vi "AlgoVita Telemetry Tool.vi"() -> ()   [LabVIEW 2020]
uses:
  Typedef Command List.ctl
  <vilib>/Instr/_visa.llb/VISA Configure Serial Port (Instr).vi
  MICS_ID Global.vi
panel:
  out "CRC Errors":u16=2650
  out "Corrected Blocks":u16=2650
  in  "PRIMARY MICS Dongle Address":refnum<visa-resource-name>="COM5"
  out "MAX_RETRIES":bool
  in  "stop":bool
  out "ERROR":bool
  out "SESSION":bool
  out "IDLE":bool
  out "Response":string
  in  "Tab Control":T1(tab)
  in  "Open Session":bool caption="Search for Device"
  in  "Close Session":bool caption="Search for Device"
  in  "Detected MICS IDs":i32(listbox)
  out "Error Monitor":errorcluster
  in  "Dongle Reset":bool caption="Search for Device"
  in  "BASE STATION RF CONTROL":T2={"CCA Mode"=FALSE, "Manual RF CH:"=2, "Base Station CCA Results"=[], "Update CCA"=FALSE, "RSSI Measurement"=0, "Use Averaging?"=TRUE, "400MHz Wakeup"=FALSE, "Listen\nfor\nEmergency"=FALSE} {"RSSI Measurement" items=["External ADC"=0, "Internal ADC"=2]; "Manual RF CH:" max=11 step=1}
  in  "SESSION CONTROL":T3={"TARGET MICS ID"=0, "EXID"=16773121, "Company ID"=187, "Antenna Calibration "=TRUE} {"Company ID" format="%02x"; "EXID" format="%06x"; "TARGET MICS ID" format="%06x"}
  out "LINK QUALITY":T4={"MAX_BIT_ERROR"=FALSE, "MAX_RETRIES"=FALSE, "Corrected Blocks"=2650, "CRC Errors"=2650}
  out "DATA STATUS":T5={"TX_BlockCount"=2650, "RX_BlockCount"=2650, "DataErrorCount"=2650}
  out "STATUS FLAGS":T6
  out "LINK STATUS":T7={"ImplantID"=0, "CompanyID"=0, "RF_Channel"=4, "RX_Mod"=0, "TX_Mod"=0, "TXBlockSize"=15, "RXBlockSize"=15, "BlocksPerPack"=31} {"BlocksPerPack" items=["1"=1, "2"=2, "3"=3, "4"=4, "5"=5, "6"=6, "7"=7, "8"=8, "9"=9, "10"=10, "11"=11, "12"=12, "13"=13, "14"=14, "15"=15, "16"=16, "17"=17, "18"=18, "19"=19, "20"=20, "21"=21, "22"=22, "23"=23, "24"=24, "25"=25, "26"=26, "27"=27, "28"=28, "29"=29, "30"=30, "31"=31]; "RXBlockSize" items=["2"=2, "3"=3, "4"=4, "5"=5, "6"=6, "7"=7, "8"=8, "9"=9, "10"=10, "11"=11, "12"=12, "13"=13, "14"=14, "15"=15, "16"=16, "17"=17, "18"=18, "19"=19, "20"=20, "21"=21, "22"=22, "23"=23, "24"=24, "25"=25, "26"=26, "27"=27, "28"=28, "29"=29, "30"=30, "31"=31]; "TXBlockSize" items=["2"=2, "3"=3, "4"=4, "5"=5, "6"=6, "7"=7, "8"=8, "9"=9, "10"=10, "11"=11, "12"=12, "13"=13, "14"=14, "15"=15, "16"=16, "17"=17, "18"=18, "19"=19, "20"=20, "21"=21, "22"=22, "23"=23, "24"=24, "25"=25, "26"=26, "27"=27, "28"=28, "29"=29, "30"=30, "31"=31]; "TX_Mod" items=["2FSK-FB"=0, "2FSK"=2, "4FSK"=3]; "RX_Mod" items=["2FSK-FB"=0, "2FSK"=8, "4FSK"=12]; "RF_Channel" items=["0", "1", "2", "3", "4", "5", "6", "7", "8", "9"]; "CompanyID" format="%02x"; "ImplantID" format="%06x"}
  out "BASE STATION INFO":string
  in  "Query Error":bool caption="Search for Device"
  in  "BaseStationInfo":enum32{"Type", "Name", "Version", "Error"}(radio)=enum."Error"
  in  "Search for Device":bool
  in  "Device Found?":bool
  in  "Dwell Time (mS)":u32=250
  out "Time to Open Session, Secs":dbl
  out "Error Flag":string="ERROR"
  in  "Clear Error":bool caption="Search for Device"
  in  "TelemGetZarlinkTrim1":bool caption="Search for Device"
  in  "TelemGetGenCals":bool caption="Search for Device"
  in  "TelemOpenLeadLimits":bool caption="Search for Device"
  in  "TelemGetIdentity":bool caption="Search for Device"
  in  "TelemTuneMICS":bool caption="Search for Device"
  in  "TelemStorage":bool caption="Search for Device"
  in  "TelemReset":bool caption="Search for Device"
  in  "TelemGetStatus":bool caption="Search for Device"
  in  "CopyDataToParams":bool caption="Search for Device"
  in  "Load Template":bool caption="Search for Device"
  in  "Telem Driver":bool caption="Search for Device"
  in  "Parameters":string
  out "Data":string
  out "bChecksum Valid":bool
  out "tChecksum Valid":bool
  out "Response Token":string
  out "Response Code":string
  in  "Command":T8
  in  "CP_DATA IN":u8[](array[numeric])
  out "CP_DATA OUT":u8[](array[numeric])
  out "Offset":u16
  out "Bias":u16
  out "Input":u16
  out "Charge/Temp Warning":bool
  out "Temp Cal":bool
  in  "VBAT Polling Speed":enum32{"3s", "5s", "10s", "15s"}(radio)=enum."5s"
  in  "Get VBAT Cont":bool
  in  "Get VBAT Single":bool
  out "Thermometer":dbl(slide) scale=36.0..43.0
  out "Reported Temperature Status":string
  out "Temperature History":dbl(graph)
  out "T1 Cal Factor":dbl format="%_7g"
  out "T1 Ohms":dbl
  out "TEMP (°C)":dbl format="%.3f"
  out "Reported Charging Status":string
  out "Battery Status (Volts)":dbl(slide) scale=3.5..4.12
  out "VRECT Input Power":u8(knob) scale=0.0..255.0
  out "VBAT Cal":dbl format="%_7g"
  out "ADC Counts":dbl
  out "VBAT (Volts)":dbl format="%.3f"
  out "Charging Status":string
  out "Active":i32
  in  "Discharge Target":dbl=3.87
  in  "Discharge":T9(array[cluster]) {"MICS ID" format="%06x"; "VBAT" format="%_3g"}
  in  "LoadPatProgSlot":u8=1 min=1 max=10 step=1
  in  "LoadPatProgFromDevice":bool caption="Search for Device"
  in  "ResetPatProgToDefaults":bool caption="Search for Device"
  in  "LoadPatProgFromFile":bool caption="Search for Device"
  in  "SavePatProgToFile":bool caption="Search for Device"
  in  "PulsePW":u16
  in  "PulsePWDn":bool
  in  "PulsePWUp":bool
  in  "Pulse #":u8=1 min=1 max=4 step=1
  in  "PulseAmpl":u16
  in  "PulseAmpDn":bool
  in  "PulseAmpUp":bool
  in  "StopStimulation":bool caption="Search for Device"
  in  "StartStimulation":bool caption="Search for Device"
  in  "SetPatProgActive":bool caption="Search for Device"
  in  "SendPatProgToDevice":bool caption="Search for Device"
  in  "UpdatePatProgString":bool caption="Search for Device"
  in  "Patient Program String":string
  in  "Freq Index":u8
  in  "ProgAmpls":u16[](array[numeric])
  in  "FreqDn":bool
  in  "FreqUp":bool
  in  "ProgAmpDn":bool
  in  "ProgAmpUp":bool
  in  "PatStim":T10={"PA"={"Defined"=FALSE, "Amplitudes"=[0, 0, 0, 0, 0, 0, 0, 0, 0, 0, 0, 0, 0, 0, 0, 0, 0, 0, 0, 0, 0, 0, 0, 0, 0, 0], "Pulse Name"="", "Label.Ch"=["ch1", "ch2", "ch3", "ch4", "ch5", "ch6", "ch7", "ch8", "ch9", "ch10", "ch11", "ch12", "ch13", "ch14", "ch15", "ch16", "ch17", "ch18", "ch19", "ch20", "ch21", "ch22", "ch23", "ch24", "ch25", "ch26"], "Amp Low Limit (uA)"=0, "Amp Step (uA)"=0, "Amp Step Index"=0, "PW Low Limit (uS)"=0, "PW High Limit (uS)"=0, "PW Default (uS)"=0}, "Allowed Freq Indexes"=[], "PB"={"Defined"=FALSE, "Amplitudes"=[0, 0, 0, 0, 0, 0, 0, 0, 0, 0, 0, 0, 0, 0, 0, 0, 0, 0, 0, 0, 0, 0, 0, 0, 0, 0], "Pulse Name"="", "Label.Ch"=["ch1", "ch2", "ch3", "ch4", "ch5", "ch6", "ch7", "ch8", "ch9", "ch10", "ch11", "ch12", "ch13", "ch14", "ch15", "ch16", "ch17", "ch18", "ch19", "ch20", "ch21", "ch22", "ch23", "ch24", "ch25", "ch26"], "Amp Low Limit (uA)"=0, "Amp Step (uA)"=0, "Amp Step Index"=0, "PW Low Limit (uS)"=0, "PW High Limit (uS)"=0, "PW Default (uS)"=0}, "PC"={"Defined"=FALSE, "Amplitudes"=[0, 0, 0, 0, 0, 0, 0, 0, 0, 0, 0, 0, 0, 0, 0, 0, 0, 0, 0, 0, 0, 0, 0, 0, 0, 0], "Pulse Name"="", "Label.Ch"=["ch1", "ch2", "ch3", "ch4", "ch5", "ch6", "ch7", "ch8", "ch9", "ch10", "ch11", "ch12", "ch13", "ch14", "ch15", "ch16", "ch17", "ch18", "ch19", "ch20", "ch21", "ch22", "ch23", "ch24", "ch25", "ch26"], "Amp Low Limit (uA)"=0, "Amp Step (uA)"=0, "Amp Step Index"=0, "PW Low Limit (uS)"=0, "PW High Limit (uS)"=0, "PW Default (uS)"=0}, "PD"={"Defined"=FALSE, "Amplitudes"=[0, 0, 0, 0, 0, 0, 0, 0, 0, 0, 0, 0, 0, 0, 0, 0, 0, 0, 0, 0, 0, 0, 0, 0, 0, 0], "Pulse Name"="", "Label.Ch"=["ch1", "ch2", "ch3", "ch4", "ch5", "ch6", "ch7", "ch8", "ch9", "ch10", "ch11", "ch12", "ch13", "ch14", "ch15", "ch16", "ch17", "ch18", "ch19", "ch20", "ch21", "ch22", "ch23", "ch24", "ch25", "ch26"], "Amp Low Limit (uA)"=0, "Amp Step (uA)"=0, "Amp Step Index"=0, "PW Low Limit (uS)"=0, "PW High Limit (uS)"=0, "PW Default (uS)"=0}, "label.freqindex"=[], "Default Freq Index"=1, "Program Name"="", "Program Number"=0, "Program Defined"=FALSE, "Program Disabled"=FALSE} {"Default Freq Index" min=1 max=64 step=1; "Allowed Freq Indexes" format="%02x"}
  in  "RFStop":bool
  out "RFST":T11(ring)
  in  "Save RF Scan Report":bool
  in  "Test Device Info (for report):":string
  in  "Run RF Job":bool
  in  "Load RF Job":bool
  in  "Save RF Job":bool
  in  "Test Job Note":string
  in  "Test Job":T12(array[cluster]) {"Attenuator, dB" min=0.0 max=31.25 step=0.25 format="%.2f"}
  out "Wakeup Scan Results":string
  out "RFScanStat":T13 {"Job" scale=0.0..1.0; "Section" scale=0.0..1.0}
  in  "Test Drive Level":enum16{"Low (200uA)", "High (500uA)"}(ring)=enum."High (500uA)"
  in  "Quick Imp Meas":bool
  in  "Channel B":u8=1 min=1 max=25 step=1
  in  "Channel A":u8=1 min=1 max=25 step=1
  in  "Matrix Imp Meas":bool
  in  "Single Imp Meas":bool
  out "Impedance Measurement Results":string
  in  "Clear Device Data":bool
  in  "DevDataSaveAll":bool
  in  "ConstSetAll":bool
  in  "ConstGetAll":bool
  in  "ConstantsGet":bool
  in  "ConstantsSet":bool
  in  "DevDataSave":bool
  in  "ConstantsLoad":bool
  in  "DevDataTabs":T14(tab)=enum."Device Identity"
  out "Activity Log":string
  out "Error Log":string
  out "xPG Identity Data":string
  out "General Calibration Data":string
  out "Pulse Constants Data":string
  out "Program Constants Data":string
  out "HV Calibrations Data":string
  in  "ChanCalTabs":enum32{"0-3mA", "3-6mA", "6-9mA", "9-15mA"}(tab)
  out "Channel Cals 0-3mA":string
  out "Channel Cals 3-6mA":string
  out "Channel Cals 6-9mA":string
  out "Channel Cals 9-15mA":string
  in  "TrimListTabs":T15(tab)
  out "Trim List 0":string
  out "Trim List 1":string
  out "Trim List 2":string
  out "Trim List 3":string
  out "Lead Limits":string
  out "Configurable Device Params":string
  out "Event Counters Data":string
  in  "CPDataTabs":T16(tab)
  out "CP Data 0":string
  out "CP Data 1":string
  out "CP Data 2":string
  out "CP Data 3":string
  out "CP Data 4":string
  out "CP Data 5":string
  out "CP Data 6":string
  out "CP Data 7":string
  in  "ProgramData":T17(tab)
  out "Program Data 1":string
  out "Program Data 2":string
  out "Program Data 3":string
  out "Program Data 4":string
  out "Program Data 5":string
  out "Program Data 6":string
  out "Program Data 7":string
  out "Program Data 8":string
  out "Program Data 9":string
  out "Program Data 10":string
  out "LINK QUALITY MONITOR":T4={"MAX_BIT_ERROR"=FALSE, "MAX_RETRIES"=FALSE, "Corrected Blocks"=2650, "CRC Errors"=2650}
  in  "AttenZero":bool caption="Search for Device"
  in  "Atten -1 dB":bool caption="Search for Device"
  in  "Atten +1 dB":bool caption="Search for Device"
  in  "Set Attenuator":bool caption="Search for Device"
  in  "Get Attenuator":bool caption="Search for Device"
  in  "Attenuation (dB)":dbl min=0.0 max=31.75 step=0.25 format="%.2g"
  out "RSSI Remote 2.45":i16
  out "RSSI Remote 400":i16
  out "RSSI Base 400":i16
  in  "Get RSSI Remote 400":bool
  in  "Remote 400MHz RSSI Mode":T18(ring)=enum."Peak, 10 Rdngs"
  in  "Measurement Type":T19(ring)
  in  "Remote 2.45G RSSI Mode":enum16{"Single Reading", "Average, 20 Rdngs"}(ring)=enum."Average, 20 Rdngs"
  in  "Base 400MHz RSSI Mode":enum16{"Single Reading", "Average, 10 Rdngs"}(ring)=enum."Average, 10 Rdngs"
  in  "Get RSSI Remote 2.45":bool
  in  "Get RSSI Base 400":bool
  in  "400MHz Power - Remote":u8 max=63 step=1 format="%02x"
  in  "Set Remote Pwr":bool
  in  "Set Base Pwr":bool
  in  "245TX Power (dBm)":i8(ring) items=["-29"=-29, "-4"=-4, "-2"=-2, "0"=0, "2"=2, "4"=4, "6"=6, "8"=8, "10"=10, "12"=12, "14"=14, "16"=16, "18"=18, "20"=20, "22"=22, "24"=24, "26"=26, "27"=27]
  in  "400MHz Power - Base":u8 max=63 step=1 format="%02x"
  in  "Set CW":bool
  in  "TX Mode":bool
  in  "Frequency Range":enum16{"2.45GHz", "400MHz"}(ring)
  in  "400MHz Channel":u8 max=11
  out "Wakeup Cal Results":string
  in  "Wakeup Cal Tool":bool caption="Search for Device"
  in  "Enable \"C\" Table":bool
  in  "Enable \"D\" Table":bool
  in  "Valid Entries \"C\"":u8
  in  "Valid Entries \"D\"":u8
  in  "Set_INFO_D":bool caption="Search for Device"
  in  "Get_INFO_D":bool caption="Search for Device"
  in  "Set_INFO_C":bool caption="Search for Device"
  in  "Get_INFO_C":bool caption="Search for Device"
  in  "CalData_C":u8[][](array[numeric]) format="%02x"
  in  "CalData_D":u8[][](array[numeric]) format="%02x"
  in  "File Path":path
  in  "ZL Mass Read":bool caption="Search for Device"
  out "Get Data Dec":u8
  in  "Register":u16(ring)=1000 items=["---MANUAL ENTRY---"=1000, "REG_NOREG"=0, "REG_RXBUFF_USED"=1, "REG_RXBUFF_BSIZE"=2, "REG_TXBUFF_USED"=3, "REG_TXBUFF_BSIZE"=4, "REG_TXBUFF_MAXPACKSIZE"=5, "REG_MAC_ERRCLR"=6, "REG_MAC_TRAINNUM"=7, "REG_MAC_SYNCMATCH"=8, "REG_MAC_SYNC1"=9, "REG_MAC_SYNC2"=10, "REG_MAC_SYNC3"=11, "REG_MAC_SYNC4"=12, "REG_MAC_SYNC5"=13, "REG_MAC_MAXBERR"=14, "REG_MAC_ECCORR"=15, "REG_MAC_CRCERR"=16, "REG_MAC_BLKCNT1"=17, "REG_MAC_BLKCNT2"=18, "REG_MAC_IMDTRANSID1"=19, "REG_MAC_IMDTRANSID2"=20, "REG_MAC_IMDTRANSID3"=21, "REG_MAC_COMPANYID"=22, "REG_MAC_MODUSER"=23, "REG_MAC_CHANNEL"=25, "REG_MAC_CLEARWDOG"=26, "REG_MAC_CKCORRTHRESH"=27, "REG_HK_TXADDR"=28, "REG_HK_TXDATA"=29, "REG_HK_TXREPLY"=30, "REG_HK_USERDATA"=31, "REG_HK_USERSTATUS"=32, "REG_HK_LASTADDRESS"=33, "REG_HK_MODE"=34, "REG_MAC_STATUSSEQ"=35, "REG_MAC_MAXRETRIES"=36, "REG_MAC_RESENDTIME"=37, "REG_MAC_POWERSAVETIME"=38, "REG_MAC_HEAD_DET"=39, "REG_MAC_CTRL"=41, "REG_MAC_INITCOM"=42, "REG_INTERFACE_MODE"=43, "REG_TXRXBUFF_BOTH"=44, "REG_TXRXBUFF"=45, "REG_IRQ_RAWSTATUS1"=46, "REG_IRQ_ENABLE1"=47, "REG_IRQ_ENABLESET1"=48, "REG_IRQ_ENABLECLEAR1"=49, "REG_IRQ_RAWSTATUS2"=50, "REG_IRQ_ENABLE2"=51, "REG_IRQ_ENABLESET2"=52, "REG_IRQ_ENABLECLEAR2"=53, "REG_IRQ_STATUS1"=54, "REG_IRQ_STATUS2"=55, "REG_IRQ_AUXSTATUS"=56, "REG_TXBUFF_OVERFLOW"=57, "REG_PO0"=58, "REG_P01"=59, "REG_P02"=60, "REG_P03"=61, "REG_GP0"=62, "REG_GPI"=63, "REG_WAKEUP_245IN"=64, "REG_WAKEUP_COMPANYID"=65, "REG_WAKEUP_IMDTRANSID1"=66, "REG_WAKEUP_IMDTRANSID2"=67, "REG_WAKEUP_IMDTRANSID3"=68, "REG_WAKEUP_CHANNEL"=69, "REG_WAKEUP_MODUSER"=70, "REG_WAKEUP_DEVICEMODE"=71, "REG_WAKEUP_WK_RX_CTRL1"=72, "REG_WAKEUP_STACK_ADDR"=73, "REG_WAKEUP_CTRL"=74, "REG_WAKEUP_STROSCRTRIM"=75, "REG_WAKEUP_BIASTRIM"=76, "REG_WAKEUP_ANT245TUNE"=77, "REG_WAKEUP_WK_RX_RTRIMDET"=78, "REG_WAKEUP_WK_RX_RTRIMDEMOD"=79, "REG_WAKEUP_WK_RX_RSSIGAIN"=80, "REG_WAKEUP_LNAFREQ1"=81, "REG_WAKEUP_STACK"=83, "REG_WAKUP_XOSU"=84, "REG_WAKUP_CNTDROPOUT"=85, "REG_WAKEUP_CRCCTRL"=86, "REG_WAKEUP_CRCWORD1"=87, "REG_WAKEUP_CRCWORD2"=88, "REG_WAKEUP_WK_RX_CTRIM"=89, "REG_WAKEUP_VDDATRIM"=90, "REG_WAKEUP_VDDDTRIM"=91, "REG_WAKEUP_TESTIOBUFEN"=92, "REG_WAKEUP_TESTIOCLAMP"=93, "CORE_RESET_ADDRESS"=94, "CHIP_RESET_ADDRESS"=95, "REG_RF_TXGENCTRL"=96, "REG_RF_TXIFCTRL"=97, "REG_RF_TXRF_SEL_CTRL"=98, "REG_RF_TXRFPWRDEFAULTSET"=99, "REG_RF_RSSITRIM"=100, "REG_RF_TXIFOSCTUNE"=101, "REG_RF_TXIFGAINIMB"=102, "REG_RF_TXIFLOCK"=103, "REG_RF_RXRFLNAGAINTRIM"=104, "REG_RF_RXBIASTR"=105, "REG_RF_RXGENCTRL"=106, "REG_RF_RXIFADCDECLEV"=107, "REG_RF_RXIFDETFILTERTUNE"=108, "REG_RF_RXIFFILTERTUNE"=109, "REG_RF_GENENABLES"=110, "REG_RF_SYNTH_CHANNEL"=111, "REG_TX_RAMP_RTRIM"=112, "REG_TX_RAMP_CTRIM"=113, "REG_RF_XO_TRIM"=114, "REG_RF_SYNTH_SET_TRIM"=115, "REG_RF_ADCCTRL"=116, "REG_RF_ADCOUTPUT"=117, "REG_RF_TXIFAMP"=118, "REG_RF_SYNTH_RTRIM"=119, "REG_RF_SYNTH_CTRIM"=120, "REG_RF_SYNTH_CT"=121, "REG_RF_TXMIXER_IOSTRIM_HIGH_IP"=122, "REG_RF_TXMIXER_IOSTRIM_HIGH_IN"=123, "REG_RF_TXMIXER_IOSTRIM_HIGH_QP"=124, "REG_RF_TXMIXER_IOSTRIM_HIGH_QN"=125, "REG_HX_WUADDR"=126, "REG_REVISION"=127, "REG_NOREG_TEST"=128, "REG_DTEST_RXBUFF"=129, "REG_RXBUFF_NEXT_BLOCK"=130, "REG_RXBUFF_FIRST_IN_PACK"=131, "REG_RXBUFF_FIRST_EMPTY"=132, "REG_MAC_BYPASS"=133, "REG_DTEST_TXBUFF"=134, "REG_TXBUFF_NEXT_BLOCK"=135, "REG_TXBUFF_FIRST_IN_PACK"=136, "REG_TXBUFF_FIRST_EMPTY"=137, "REG_DTEST_SEQ"=138, "REG_DTEST_CKCORR"=139, "REG_MAC_TOPSTATE"=140, "REG_DTEST_INTERFACE"=141, "REG_IFACE_TXRX_BYPASS"=142, "REG_MAC_TXRXWAIT"=143, "REG_MAC_TXRFRAMP"=144, "REG_MAC_TRAINWORD"=145, "REG_MAC_TRAINWORD2"=146, "REG_MAC_SETTINGS"=147, "REG_MAC_CALSELECT1"=148, "REG_MAC_CALSELECT2"=149, "REG_MAC_ANTMATCHSEL"=150, "REG_MAC_ANTTUNESEL1"=151, "REG_MAC_ANTTUNESEL2"=152, "REG_MAC_ANTTUNESEL3"=153, "REG_MAC_ANTTUNESTEP"=154, "REG_MAC_WUMODEBURST"=156, "REG_MAC_WUOFFSHORT"=157, "REG_MAC_WUOFFLONG"=158, "REG_MAC_CLKRECCTRL"=159, "REG_HK_MODE_P2"=162, "REG_MAC_ANTTUNERES1"=164, "REG_MAC_ANTTUNERES2"=165, "REG_INTERFACE_MODE_TEST"=171, "REG_TXRXBUFF_BOTH_P2"=172, "REG_TXRXBUFF_P2"=173, "REG_IRQ_RAWSTATUS1_P2"=174, "REG_MAC_TXIFSTATUS1"=176, "REG_MAC_TXIFSTATUS2"=177, "REG_IRQ_RAWSTATUS2_P2"=178, "REG_MAC_TXIFRAMPDELAY"=179, "REG_MAC_TXIFRAMPSLOPE"=180, "REG_MAX_TXIFRAMP"=181, "REG_IRQ_STATUS1_P2"=182, "REG_IRQ_STATUS2_P2"=183, "REG_IRQ_AUXSTATUS_P2"=184, "REG_MAC_UNLOCK"=188, "REG_MAC_TXIFFREQ"=190, "REG_WAKEUP_TESTCTRL1"=192, "REG_WAKEUP_RX_EN_CNT"=193, "REG_WAKEUP_TESTENABLES"=194, "REG_WAKEUP_DTBI_CTRL"=195, "REG_WAKEUP_DTBO_CTRL"=196, "REG_WAKEUP_TESTIOBUFTEST"=197, "REG_WAKEUP_WK_RX_TESTCTRL1"=198, "REG_WAKEUP_WK_RX_TESTCTRL2"=199, "REG_WAKEUP_SENS_SEQUENCE_CTRL"=200, "REG_WAKEUP_LNABIAS"=201, "REG_WAKEUP_DET_TH_TRIM1"=202, "REG_WAKEUP_LNABIAS_NOM1"=203, "REG_WAKEUP_RX_TSHORT_TRIM1"=204, "REG_WAKEUP_LNABIAS_NOM2"=205, "REG_WAKEUP_RX_TLONG_TRIM1"=206, "REG_WAKEUP_LNA_NEGRTRIM_NOM1"=207, "REG_WAKEUP_RX_TBURST_TRIM1"=208, "REG_WAKEUP_RX_LNA_NEGRTRIM_NOM2"=209, "REG_WAKEUP_RX_BB_G_BW_SEL1"=210, "REG_WAKEUP_WK_RX_DET_IOSTRIM1"=212, "REG_WAKEUP_WK_RX_CTRL2"=214, "REG_WAKEUP_WK_RX_RSSIVOSTRIM"=215, "REG_WAKEUP_LNANEGR_EFF"=216, "REG_WAKEUP_XOSU_FAST"=217, "REG_WAKEUP_STROSCPWIDTH1"=218, "REG_WAKEUP_STROSCPERIOD1"=220, "REG_WAKEUP_STROSCPERIOD2"=221, "REG_WAKEUP_WK_RX_LNA_NEGRTRIM1"=222, "REG_RF_TXTESTENABLE"=224, "REG_RF_TXIFTESTMODE"=225, "REG_RF_RXTESTENABLE"=226, "REG_RF_RXIFTESTCTRL1"=227, "REG_RF_RXIFTESTCTRL2"=228, "REG_RF_RXIFTESTCTRL3"=229, "REG_RF_SYNTH_TESTCTRL1"=230, "REG_RF_SYNTH_TESTCTRL2"=231, "REG_RF_SYNTH_TESTCTRL3"=232, "REG_RF_ADCTEST1"=237, "REG_RF_ADCTEST2"=238, "REG_RF_TXMIXER_IOSTRIM_LOW_IP"=240, "REG_RF_TXMIXER_IOSTRIM_LOW_IN"=241, "REG_RF_TXMIXER_ISOTRIM_LOW_QP"=242, "REG_RF_TXMIXER_IOSTRIM_LOW_QN"=243, "REG_RF_SYNTH_KPD"=244, "REG_RF_SYNTH_LOLEV"=245, "REG_RF_TXRFPWRTUNEANTSET"=246, "REG_RF_TXPD_GAIN_CTRL"=247, "REG_RF_SYNTH_STARTUP"=248, "REG_RF_TXRFANTTUNE_TXMODE"=249, "REG_RF_TXRFANTTUNE_RXMODE"=250, "REG_RF_RXRFANTTUNE_TXMODE"=251, "REG_RF_RXRFANTTUNE_RXMODE"=252, "REG_ANTMATCH1"=253, "REG_ANTMATCH2"=254, "REG_REVISION_P2"=255]
  in  "Set Register":bool caption="Search for Device"
  in  "Get Register":bool caption="Search for Device"
  in  "Use Remote?":bool
  out "Get Data":u8 format="%02x"
  in  "Set Data":u8 format="%02x"
  in  "Address":u16 format="%04x"
  in  "Do Calibration":bool caption="Search for Device"
  in  "CAL_WAKEUP_STROBE_OSC":bool
  in  "MICS Channel":i8
  in  "Execute on Remote?(F)":bool
  in  "CAL_TX_IF_OSC":bool
  in  "CAL_FM_DETECT_AND_RX_IF":bool
  in  "CAL_RX_ADC":bool
  in  "CAL_400_MHZ_TX":bool
  in  "CAL_400_MHZ_RX":bool
  in  "CAL_400_MHZ_ANT":bool
  in  "CAL_24MHZ_CRYSTAL_OSC":bool
  in  "SECONDARY MICS Dongle Address":refnum<visa-resource-name>="COM9"
  out "error out":errorcluster
  in  "error in (no error)":errorcluster
  in  "Default MICS Config":T20={"ConfigFlags"=0, "ImplantID"=1048576, "CompanyID"=187, "Normal_Comm"={"RF_Channel"=4, "UserData"=0, "TX_Mod"=0, "RX_Mod"=0, "RX_BlockSize"=15, "BlockPerPack"=31, "TX_BlockSize"=15}, "Emerg_Comm"={"RF_Channel"=5, "UserData"=0, "TX_Mod"=0, "RX_Mod"=0, "TX_BlockSize"=15, "BlockPerPack"=31, "RX_BlockSize"=15}, "ImplantRev"=5, "245TX_PowerCal"=10, "245TX_Power"=24, "CCA_RSSI_Thresholds"={"ch0"=2650, "ch1"=2650, "ch2"=2650, "ch3"=2650, "ch4"=2650, "ch5"=2650, "ch6"=2650, "ch7"=2650, "ch8"=2650, "ch9"=2650}} {"ImplantID" format="%x"; "Normal_Comm"."RF_Channel" items=["0", "1", "2", "3", "4", "5", "6", "7", "8", "9"]; "Normal_Comm"."UserData" items=["0 - 000"=0, "1 - 001"=16, "2 - 010"=32, "3 - 011"=48, "4 - 100"=64, "5 - 101"=80, "6 - 110"=96, "7 - 111"=112]; "Normal_Comm"."TX_Mod" items=["2FSK-FB"=0, "2FSK"=2, "4FSK"=3]; "Normal_Comm"."RX_Mod" items=["2FSK-FB"=0, "2FSK"=8, "4FSK"=12]; "Normal_Comm"."RX_BlockSize" items=["2"=2, "3"=3, "4"=4, "5"=5, "6"=6, "7"=7, "8"=8, "9"=9, "10"=10, "11"=11, "12"=12, "13"=13, "14"=14, "15"=15, "16"=16, "17"=17, "18"=18, "19"=19, "20"=20, "21"=21, "22"=22, "23"=23, "24"=24, "25"=25, "26"=26, "27"=27, "28"=28, "29"=29, "30"=30, "31"=31]; "Normal_Comm"."BlockPerPack" items=["1"=1, "2"=2, "3"=3, "4"=4, "5"=5, "6"=6, "7"=7, "8"=8, "9"=9, "10"=10, "11"=11, "12"=12, "13"=13, "14"=14, "15"=15, "16"=16, "17"=17, "18"=18, "19"=19, "20"=20, "21"=21, "22"=22, "23"=23, "24"=24, "25"=25, "26"=26, "27"=27, "28"=28, "29"=29, "30"=30, "31"=31]; "Normal_Comm"."TX_BlockSize" items=["2"=2, "3"=3, "4"=4, "5"=5, "6"=6, "7"=7, "8"=8, "9"=9, "10"=10, "11"=11, "12"=12, "13"=13, "14"=14, "15"=15, "16"=16, "17"=17, "18"=18, "19"=19, "20"=20, "21"=21, "22"=22, "23"=23, "24"=24, "25"=25, "26"=26, "27"=27, "28"=28, "29"=29, "30"=30, "31"=31]; "Emerg_Comm"."RF_Channel" items=["0", "1", "2", "3", "4", "5", "6", "7", "8", "9"]; "Emerg_Comm"."UserData" items=["0 - 000"=0, "1 - 001"=16, "2 - 010"=32, "3 - 011"=48, "4 - 100"=64, "5 - 101"=80, "6 - 110"=96, "7 - 111"=112]; "Emerg_Comm"."TX_Mod" items=["2FSK-FB"=0, "2FSK"=2, "4FSK"=3]; "Emerg_Comm"."RX_Mod" items=["2FSK-FB"=0, "2FSK"=8, "4FSK"=12]; "Emerg_Comm"."TX_BlockSize" items=["2"=2, "3"=3, "4"=4, "5"=5, "6"=6, "7"=7, "8"=8, "9"=9, "10"=10, "11"=11, "12"=12, "13"=13, "14"=14, "15"=15, "16"=16, "17"=17, "18"=18, "19"=19, "20"=20, "21"=21, "22"=22, "23"=23, "24"=24, "25"=25, "26"=26, "27"=27, "28"=28, "29"=29, "30"=30, "31"=31]; "Emerg_Comm"."BlockPerPack" items=["1"=1, "2"=2, "3"=3, "4"=4, "5"=5, "6"=6, "7"=7, "8"=8, "9"=9, "10"=10, "11"=11, "12"=12, "13"=13, "14"=14, "15"=15, "16"=16, "17"=17, "18"=18, "19"=19, "20"=20, "21"=21, "22"=22, "23"=23, "24"=24, "25"=25, "26"=26, "27"=27, "28"=28, "29"=29, "30"=30, "31"=31]; "Emerg_Comm"."RX_BlockSize" items=["2"=2, "3"=3, "4"=4, "5"=5, "6"=6, "7"=7, "8"=8, "9"=9, "10"=10, "11"=11, "12"=12, "13"=13, "14"=14, "15"=15, "16"=16, "17"=17, "18"=18, "19"=19, "20"=20, "21"=21, "22"=22, "23"=23, "24"=24, "25"=25, "26"=26, "27"=27, "28"=28, "29"=29, "30"=30, "31"=31]; "ImplantRev" items=["ZL70100"=0, "ZL70101"=1, "ZL70102"=4, "ZL70103"=5]; "245TX_PowerCal" items=["-29"=-29, "-4"=-4, "-2"=-2, "0"=0, "2"=2, "4"=4, "6"=6, "8"=8, "10"=10, "12"=12, "14"=14, "16"=16, "18"=18, "20"=20, "22"=22, "24"=24, "26"=26, "27"=27]; "245TX_Power" items=["-29"=-29, "-4"=-4, "-2"=-2, "0"=0, "2"=2, "4"=4, "6"=6, "8"=8, "10"=10, "12"=12, "14"=14, "16"=16, "18"=18, "20"=20, "22"=22, "24"=24, "26"=26, "27"=27]}
  in  "Enable WD?":bool
  in  "Wait Time (S)":u8=5
  in  "Discharge Delay":u32
  in  "Tick Count":u32
  in  "AttenMode":enum16{"Null", "Increment", "Decrement", "Zero"}(ring)
  out "Busy Flag":string="BUSY"
  out "Working MICS Config":T20
  # "Double-Click to Select"
  # "400MHz\nWakeup"
  # "Auto CCA"
  # "NOTE:  Changing the active tab will suspend the operation of the Mass Battery Discharge Tool!"
  # "CHARGING STATUS"
  # "DEVICE TEMPERATURE"
  # "MASS BATTERY DISCHARGE TOOL"
  # "Volts"
  # "x"
  # "="
  # "x"
  # "="
  # "-Abort"
  # "(Input-Offset)"
  # "R="
  # "----------------- *47000"
  # "-Critical"
  # "(Bias-Input)"
  # "-Warn"
  # "++++"
  # "When charging with manual power control,\nmaintain \"VRECT Input Power\" in the range\nof 130-150 (the \"Green\" zone on meter)."
  # "MICS ID"
  # "PA"
  # "PB"
  # "PC"
  # "PD"
  # "Program Adjust"
  # "Pulse Adjust"
  # "Pulse D"
  # "Pulse C"
  # "Pulse B"
  # "Pulse A"
  # "MICS WAKEUP SCAN"
  # "All CH referenced to STCH14."
  # "IMPEDANCE MEASUREMENT"
  # "WARNING: \"Full Matrix\"\nImpedance Measurements\ncan take several minutes!"
  # "ATTENUATOR"
  # "RSSI MEASUREMENTS"
  # "BASE STATION 400MHz RSSI"
  # "REMOTE 400MHz RSSI"
  # "(Must be in session)"
  # "REMOTE 2.45GHz RSSI"
  # "(Must be in session)"
  # "DEVICE RF POWER SETTINGS"
  # "BASE STATION"
  # "REMOTE DEVICE"
  # "(Must be in session)"
  # "CW TEST MODE CONTROL"
  # "ON"
  # "OFF"
  # "ZL REGISTER PEEK AND POKE"
  # "ZL REGISTER MASS READ TO FILE"
  # "MICS DONGLE CALIBRATION"
  # "INFO_D"
  # "Index"
  # "Address"
  # "Data"
  # "Use \"Register\" menu list for named registers,\nor leave it on \"Manual Entry\" and use the \n\"Address\" control to select a register address.\n          (Add 128 (0x80) to P2 addresses)"
  # "Use this function to copy all Zarlink registers to\na text file."
  # "INFO_C"
  # "Index"
  # "Address"
  # "Data"
  # "WAKEUP CALIBRATOR TOOL"
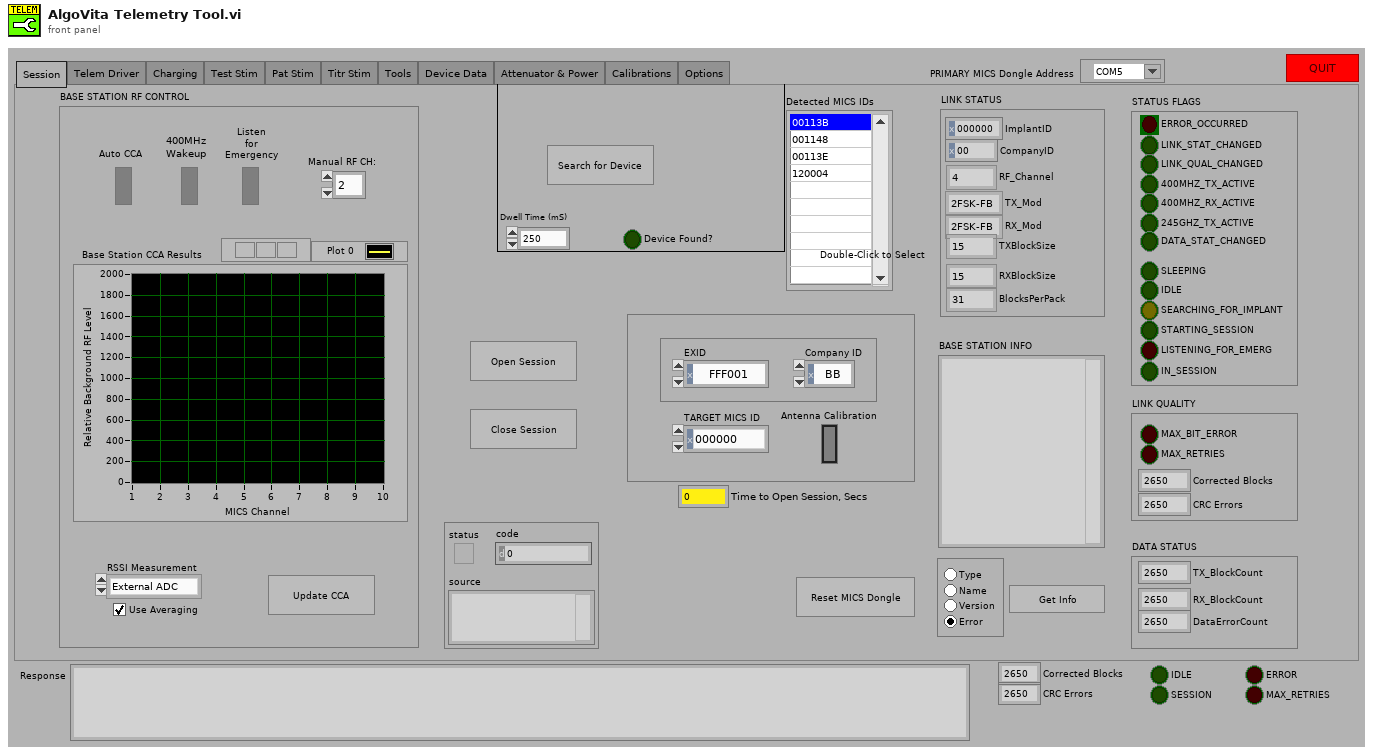
[diagram p1: front panel]
types:
  T1 = enum32{"Session", "Telem Driver", "Charging", "Test Stim", "Pat Stim", "Titr Stim", "Tools", "Device Data", "Attenuator & Power", "Calibrations", "Options"}
  T2 = cluster{"CCA Mode":bool, "Manual RF CH:":u8, "Base Station CCA Results":dbl[], "Update CCA":bool, "RSSI Measurement":u16, "Use Averaging?":bool, "400MHz Wakeup":bool, "Listen\nfor\nEmergency":bool}
  T3 = cluster{"TARGET MICS ID":u32, "EXID":u32, "Company ID":u8, "Antenna Calibration ":bool}
  T4 = cluster{"MAX_BIT_ERROR":bool, "MAX_RETRIES":bool, "Corrected Blocks":u16, "CRC Errors":u16}
  T5 = cluster{"TX_BlockCount":u16, "RX_BlockCount":u16, "DataErrorCount":u16}
  T6 = cluster{"ERROR_OCCURRED":bool, "LINK_STAT_CHANGED":bool, "LINK_QUAL_CHANGED":bool, "400MHZ_TX_ACTIVE":bool, "400MHZ_RX_ACTIVE":bool, "245GHZ_TX_ACTIVE":bool, "DATA_STAT_CHANGED":bool, "SLEEPING":bool, "IDLE":bool, "SEARCHING_FOR_IMPLANT":bool, "STARTING_SESSION":bool, "LISTENING_FOR_EMERG":bool, "IN_SESSION":bool}
  T7 = cluster{"ImplantID":u32, "CompanyID":u8, "RF_Channel":u8, "RX_Mod":u8, "TX_Mod":u8, "TXBlockSize":u8, "RXBlockSize":u8, "BlocksPerPack":u8}
  T8 = typedef "Typedef Command List.ctl" = enum16{"Get xPG Status", "xPG Stimulation", "Select Program", "Increment Program Amplitude", "Decrement Program Amplitude", "Get PoP Constants", "Get PPC Constants", "Get Program Names", "Set Pulse Amplitude", "Increment Pulse Amplitude", "Decrement Pulse Amplitude", "Get Pulse Widths", "Set Pulse Widths", "Increment Pulse Width", "Decrement Pulse Width", "Get Program Frequency", "Set Program Frequency", "Increment Program Frequency", "Decrement Program Frequency", "Inject Event", "Charging Control", "Get xPG Identity", "Set xPG Identity", "Restore Program Defaults", "Get Program Definition", "Set Program Definition", "Get Program Constants", "Set Program Constants", "Get Configurable Device Parameters", "Set Configurable Device Parameters", "Get Pulse Constants", "Set Pulse Constants", "Get Lead Limits", "Set Lead Limits", "Get Channel Calibrations", "Set Channel Calibrations", "<reserved 2>", "<reserved 3>", "<reserved 4>", "<reserved 5>", "<reserved 6>", "<reserved 7>", "Get Stim Asic HV Calibrations", "Set Stim Asic HV Calibrations", "<reserved 8>", "<reserved 9>", "Get CP Data", "Set CP Data", "Clear Log", "Read Log", "Append Log", "Get Patient Program Runtime", "Set Patient Program Runtime", "Impedance Measurement", "Enter Storage Mode", "Echo Short", "Echo Long", "Get General Calibration", "Set General Calibration", "Get Trim List", "Set Trim List", "Get Counter", "Set Counter", "Get Test Stimulation", "Set Test Stimulation", "Get Titration Stimulation", "Set Titration Stimulation", "Get Ramp Time", "Set Ramp Time", "Get VBAT", "Set Software Description Block", "Get Software Description Block", "Write Memory", "Read Memory", "Reset xPG", "Erase Flash Block", "Write Vectors", "Read Vectors", "Diagnostic Data", "Set Background Impedance", "Get Background Impedence ", "Set Test Waveform", "Calibrate Channel", "Get Log Range", "Reserved 0x55", "Reserved 0x56", "MICS Options", "Pair PPC", "Pair POP", "Stop Bootloader", "Tune MICS", "MICS Diagnostics", "Undefined"}
  T9 = cluster{"Activate":bool, "Stop":bool, "VBAT":dbl, "Discharging":bool, "Ready":bool, "MICS ID":u32}[]
  T10 = cluster{"PA":cluster{"Defined":bool, "Amplitudes":i8[], "Pulse Name":string, "Label.Ch":string[], "Amp Low Limit (uA)":u16, "Amp Step (uA)":u16, "Amp Step Index":u16, "PW Low Limit (uS)":u16, "PW High Limit (uS)":u16, "PW Default (uS)":u16}, "Allowed Freq Indexes":u8[], "PB":cluster{"Defined":bool, "Amplitudes":i8[], "Pulse Name":string, "Label.Ch":string[], "Amp Low Limit (uA)":u16, "Amp Step (uA)":u16, "Amp Step Index":u16, "PW Low Limit (uS)":u16, "PW High Limit (uS)":u16, "PW Default (uS)":u16}, "PC":cluster{"Defined":bool, "Amplitudes":i8[], "Pulse Name":string, "Label.Ch":string[], "Amp Low Limit (uA)":u16, "Amp Step (uA)":u16, "Amp Step Index":u16, "PW Low Limit (uS)":u16, "PW High Limit (uS)":u16, "PW Default (uS)":u16}, "PD":cluster{"Defined":bool, "Amplitudes":i8[], "Pulse Name":string, "Label.Ch":string[], "Amp Low Limit (uA)":u16, "Amp Step (uA)":u16, "Amp Step Index":u16, "PW Low Limit (uS)":u16, "PW High Limit (uS)":u16, "PW Default (uS)":u16}, "label.freqindex":string[], "Default Freq Index":u8, "Program Name":string, "Program Number":u8, "Program Defined":bool, "Program Disabled":bool}
  T11 = enum16{"Not Running", "Idle Interval...", "Opening Session..."}
  T12 = cluster{"Number of Runs":dbl, "2.45G_TX_Pwr":enum16{"-29", "-4", "-2", "0", "2", "4", "6", "8", "10", "12", "14", "16", "18", "20", "22", "24", "26", "27"}, "400M_TX_Pwr":enum8{"Default", "1", "2", "3", "4", "5", "6", "7", "8", "9", "10", "11", "12", "13", "14", "15", "16", "17", "18", "19", "20", "21", "22", "23", "24", "25", "26", "27", "28", "29", "30", "31"}, "Idle Interval, S":dbl, "Attenuator, dB":dbl, "MICS Chan":enum16{"CH 1", "CH 2", "CH 3", "CH 4", "CH 5", "CH 6", "CH 7", "CH 8", "CH 9", "CH 10"}, "Random\nOffset":bool}[]
  T13 = cluster{"Section":dbl, "Job":dbl, "Last Open Session Time, S":dbl, "Session Verified?":bool, "Average Open Session Time, S":dbl, "# of Open Session Failures":u16}
  T14 = enum32{"Activity Log", "Error Log", "Device Identity", "General Cals", "Pulse Constants", "Program Constants", "HV Cals", "Channel Cals", "Trim Lists", "Lead Limits", "Configurable Device Params", "Event Counters", "CP Data", "Stim Programs"}
  T15 = enum32{"Trim List 0", "Trim List 1", "Trim List 2", "Trim List 3"}
  T16 = enum32{"CP Data 0", "CP Data 1", "CP Data 2", "CP Data 3", "CP Data 4", "CP Data 5", "CP Data 6", "CP Data 7"}
  T17 = enum32{"Program 1", "Program 2", "Program 3", "Program 4", "Program 5", "Program 6", "Program 7", "Program 8", "Program 9", "Program 10"}
  T18 = enum16{"Single Reading", "Average, 10 Rdngs", "Peak, 10 Rdngs"}
  T19 = enum8{"EXT_RSSI_EXT_ADC (0)", "EXT_RSSI_INT_ADC (1)", "INT_RSSI_INT_ADC (2)"}
  T20 = cluster{"ConfigFlags":u8, "ImplantID":u32, "CompanyID":u8, "Normal_Comm":cluster{"RF_Channel":u8, "UserData":u8, "TX_Mod":u8, "RX_Mod":u8, "RX_BlockSize":u8, "BlockPerPack":u8, "TX_BlockSize":u8}, "Emerg_Comm":cluster{"RF_Channel":u8, "UserData":u8, "TX_Mod":u8, "RX_Mod":u8, "TX_BlockSize":u8, "BlockPerPack":u8, "RX_BlockSize":u8}, "ImplantRev":u8, "245TX_PowerCal":i8, "245TX_Power":i8, "CCA_RSSI_Thresholds":cluster{"ch0":u16, "ch1":u16, "ch2":u16, "ch3":u16, "ch4":u16, "ch5":u16, "ch6":u16, "ch7":u16, "ch8":u16, "ch9":u16}}
  T21 = cluster{"Command":T8, "Function":enum16{"Open Session", "Close Session", "Downlink Only", "Uplink Only", "Transceive (DN -> UP)"}, "MICS_ID":u32, "EXID":u32, "Use Local":bool, "Transceive Delay mS":dbl, "CP_DATA IN":u8[], "Parameters":string}
  T22 = enum16{"Open Session", "Close Session", "Downlink Only", "Uplink Only", "Transceive (DN -> UP)"}
  T23 = enum8{"Enabled", "Disabled", "Disabled and Grayed Out"}
  T24 = cluster{"Activate":bool, "Stop":bool, "VBAT":dbl, "Discharging":bool, "Ready":bool, "MICS ID":u32}
  T25 = enum16{"Start Search", "Continue Search", "End Search"}
  T26 = enum16{"open", "replace", "create", "open or create", "replace or create", "replace or create with confirmation"}
  T27 = enum16{"Get Device Type", "Get Device Name", "Get Device Version", "Get Device Error"}
  T28 = cluster{"Response Token":string, "Response Code":string, "bChecksum Valid":bool, "tChecksum Valid":bool, "CP_DATA OUT":u8[], "Data":string}
  T29 = cluster{"Allowed Freq Indexes[0]":u8, "Allowed Freq Indexes[1]":u8, "Allowed Freq Indexes[2]":u8, "Allowed Freq Indexes[3]":u8, "Allowed Freq Indexes[4]":u8, "Allowed Freq Indexes[5]":u8, "Allowed Freq Indexes[6]":u8, "Allowed Freq Indexes[7]":u8}
  T30 = cluster{"Number of Runs":dbl, "2.45G_TX_Pwr":enum16{"-29", "-4", "-2", "0", "2", "4", "6", "8", "10", "12", "14", "16", "18", "20", "22", "24", "26", "27"}, "400M_TX_Pwr":enum8{"Default", "1", "2", "3", "4", "5", "6", "7", "8", "9", "10", "11", "12", "13", "14", "15", "16", "17", "18", "19", "20", "21", "22", "23", "24", "25", "26", "27", "28", "29", "30", "31"}, "Idle Interval, S":dbl, "Attenuator, dB":dbl, "MICS Chan":enum16{"CH 1", "CH 2", "CH 3", "CH 4", "CH 5", "CH 6", "CH 7", "CH 8", "CH 9", "CH 10"}, "Random\nOffset":bool}
  T31 = enum16{"-29", "-4", "-2", "0", "2", "4", "6", "8", "10", "12", "14", "16", "18", "20", "22", "24", "26", "27"}
  T32 = enum8{"Default", "1", "2", "3", "4", "5", "6", "7", "8", "9", "10", "11", "12", "13", "14", "15", "16", "17", "18", "19", "20", "21", "22", "23", "24", "25", "26", "27", "28", "29", "30", "31"}
  T33 = enum16{"CH 1", "CH 2", "CH 3", "CH 4", "CH 5", "CH 6", "CH 7", "CH 8", "CH 9", "CH 10"}
  T34 = cluster{"Test Job Note":string, "Test Job":cluster{"Number of Runs":dbl, "2.45G_TX_Pwr":enum16{"-29", "-4", "-2", "0", "2", "4", "6", "8", "10", "12", "14", "16", "18", "20", "22", "24", "26", "27"}, "400M_TX_Pwr":enum8{"Default", "1", "2", "3", "4", "5", "6", "7", "8", "9", "10", "11", "12", "13", "14", "15", "16", "17", "18", "19", "20", "21", "22", "23", "24", "25", "26", "27", "28", "29", "30", "31"}, "Idle Interval, S":dbl, "Attenuator, dB":dbl, "MICS Chan":enum16{"CH 1", "CH 2", "CH 3", "CH 4", "CH 5", "CH 6", "CH 7", "CH 8", "CH 9", "CH 10"}, "Verify\nSessions":bool}[]}
  T35 = cluster{"Number of Runs":dbl, "2.45G_TX_Pwr":enum16{"-29", "-4", "-2", "0", "2", "4", "6", "8", "10", "12", "14", "16", "18", "20", "22", "24", "26", "27"}, "400M_TX_Pwr":enum8{"Default", "1", "2", "3", "4", "5", "6", "7", "8", "9", "10", "11", "12", "13", "14", "15", "16", "17", "18", "19", "20", "21", "22", "23", "24", "25", "26", "27", "28", "29", "30", "31"}, "Idle Interval, S":dbl, "Attenuator, dB":dbl, "MICS Chan":enum16{"CH 1", "CH 2", "CH 3", "CH 4", "CH 5", "CH 6", "CH 7", "CH 8", "CH 9", "CH 10"}, "Verify\nSessions":bool}[]
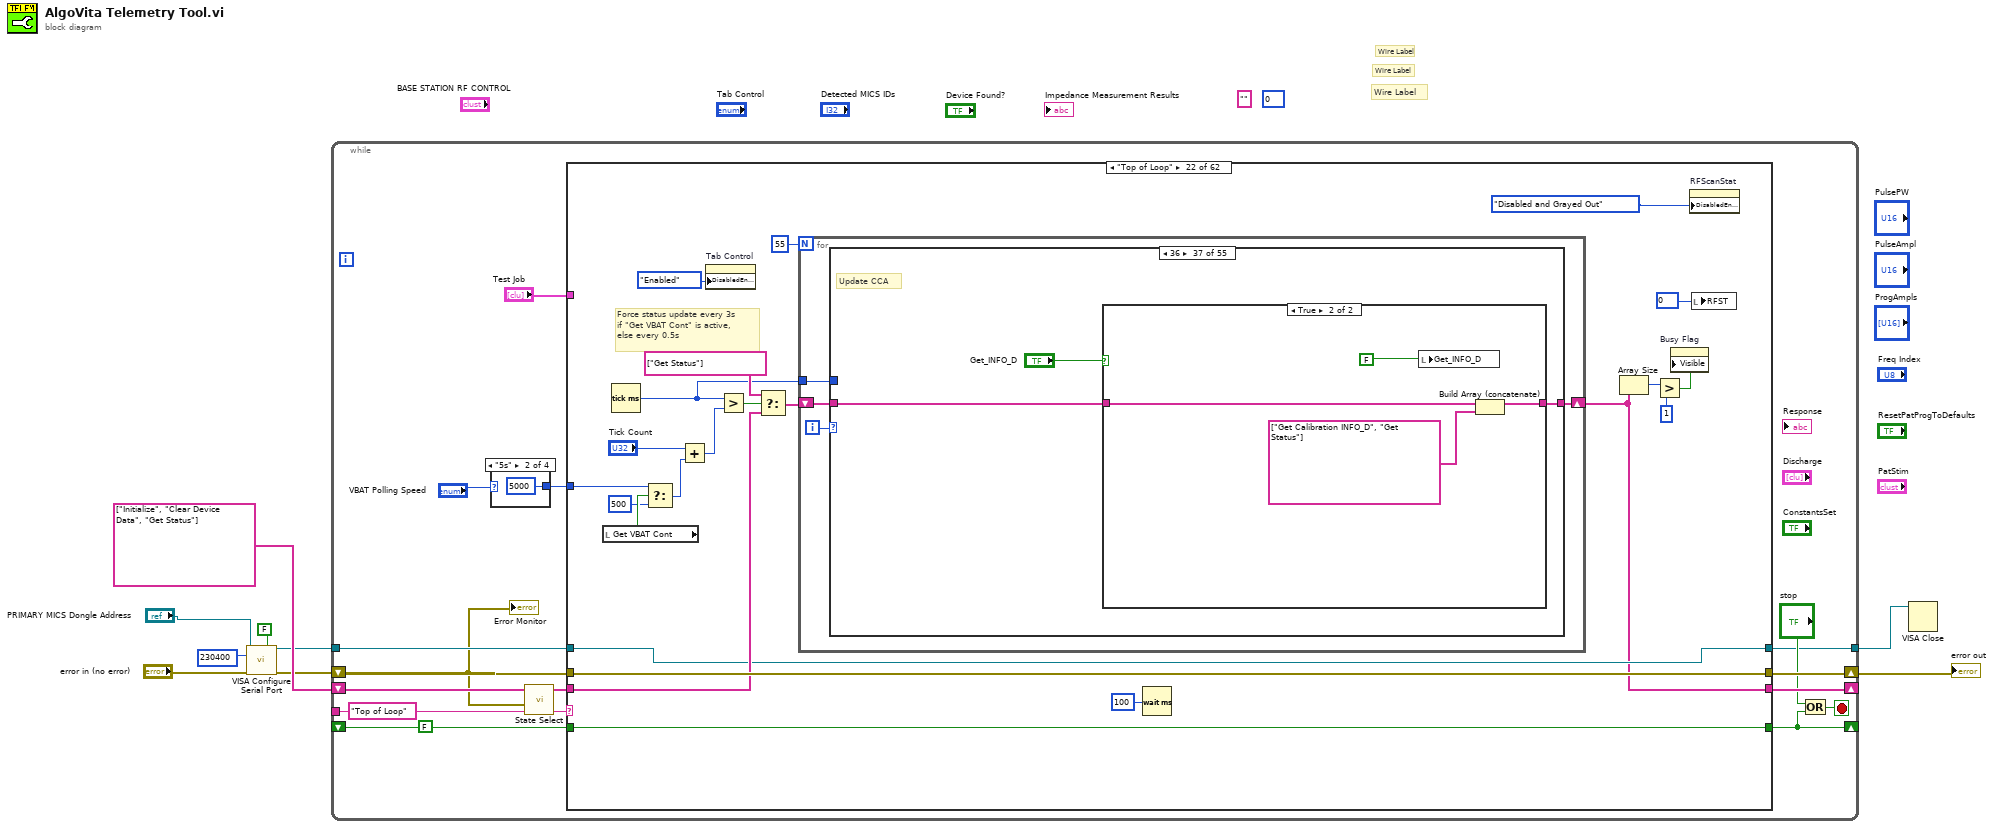
[diagram p0: block diagram]
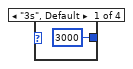
[diagram p2: hidden frame]
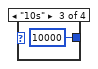
[diagram p3: hidden frame]
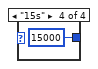
[diagram p4: hidden frame]
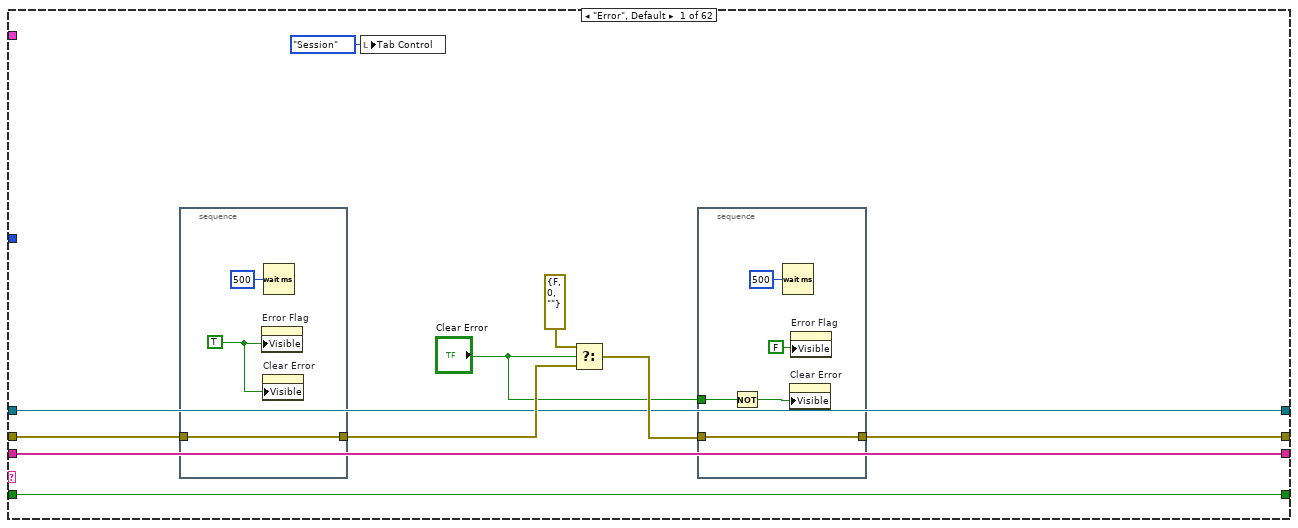
[diagram p5: hidden frame]
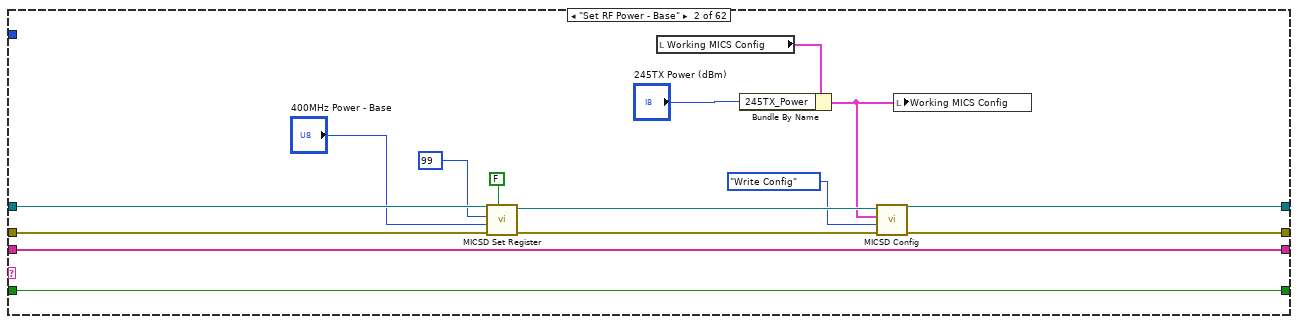
[diagram p6: hidden frame]
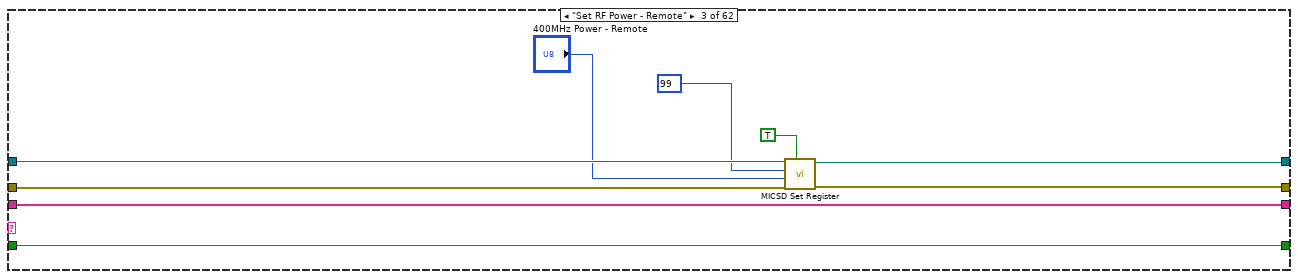
[diagram p7: hidden frame]
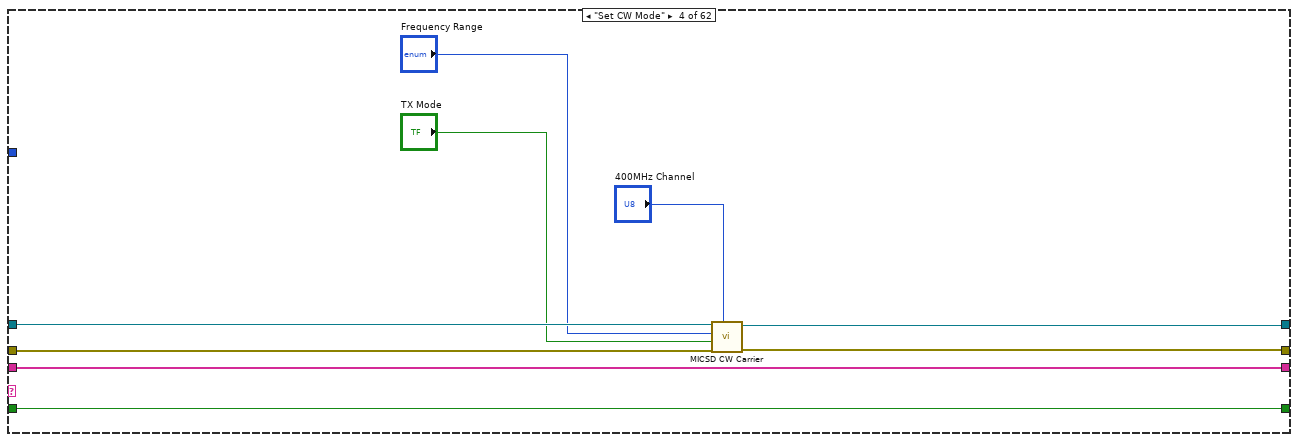
[diagram p8: hidden frame]
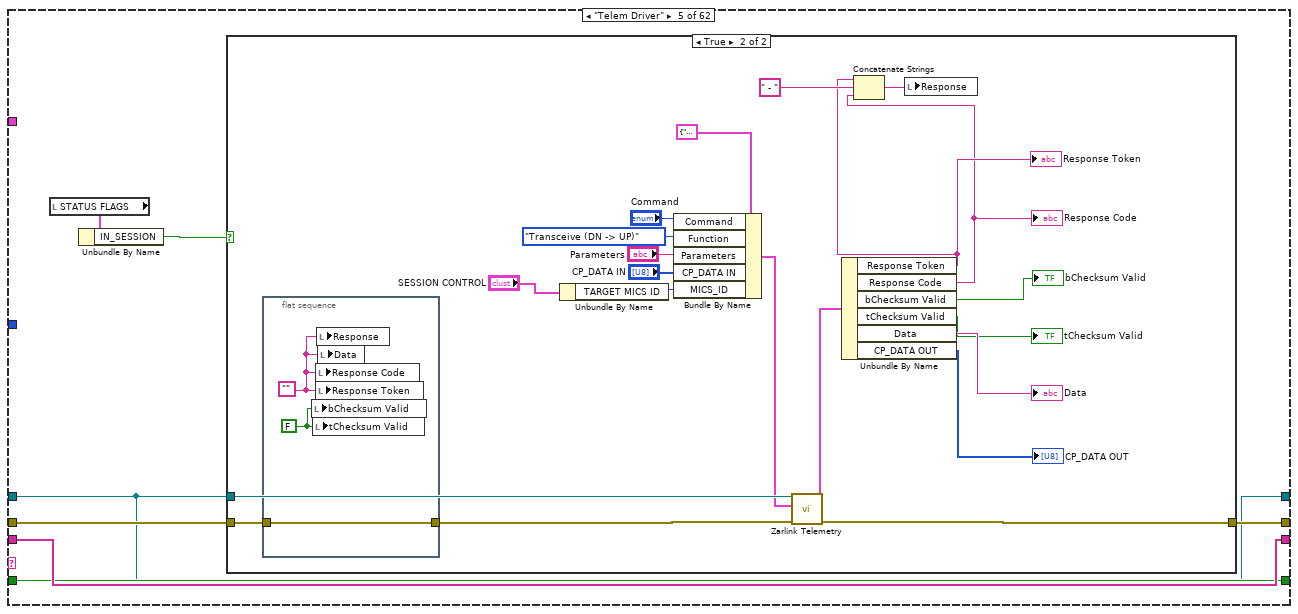
[diagram p9: hidden frame]
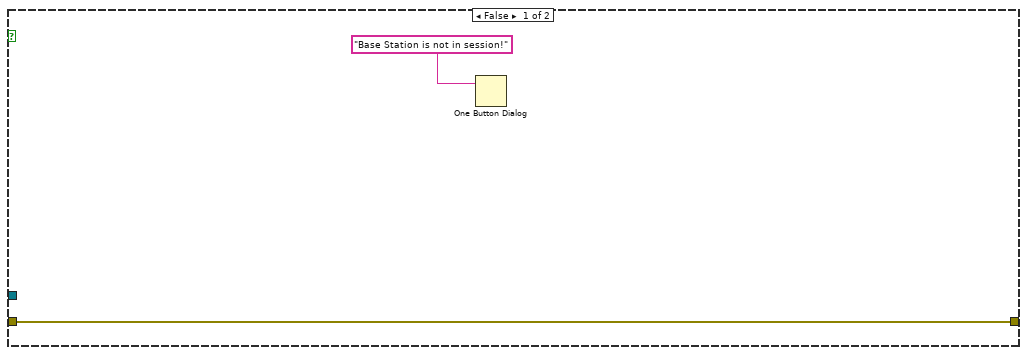
[diagram p10: hidden frame]
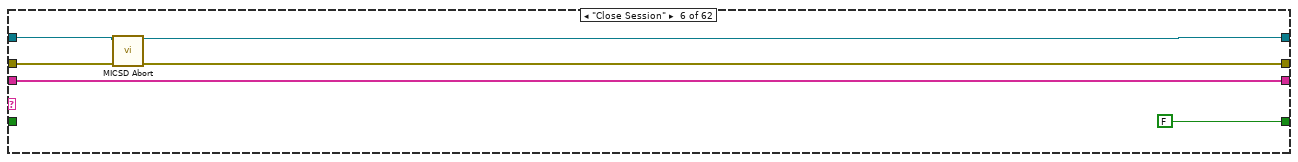
[diagram p11: hidden frame]
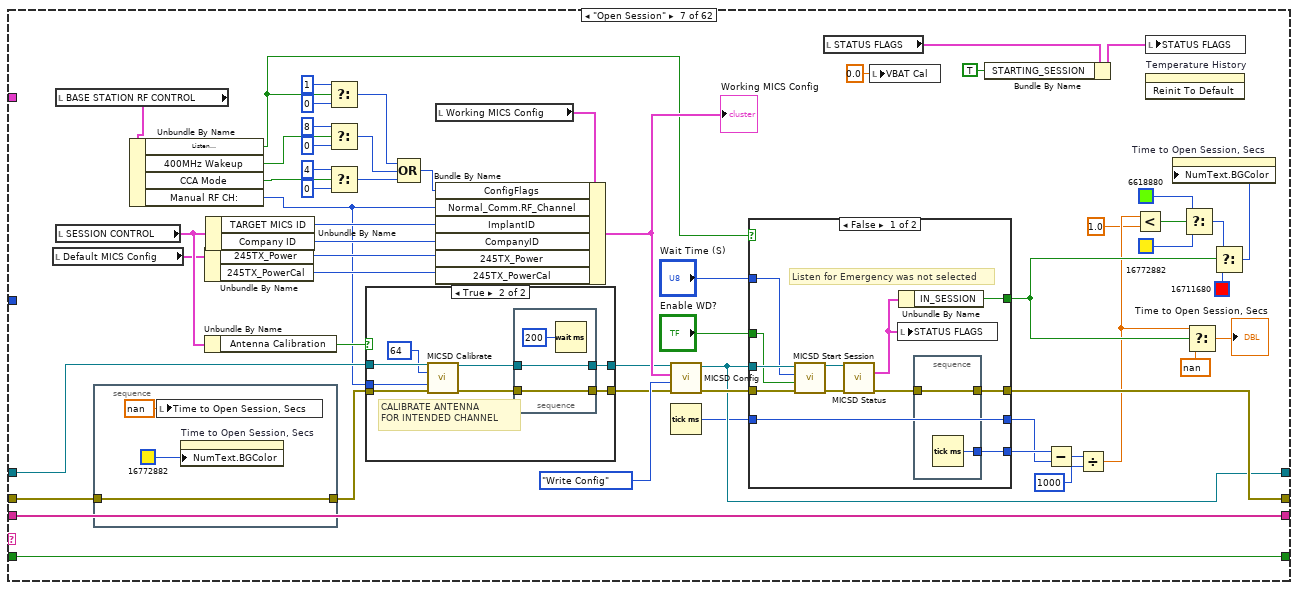
[diagram p12: hidden frame]
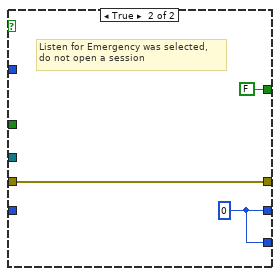
[diagram p14: hidden frame]
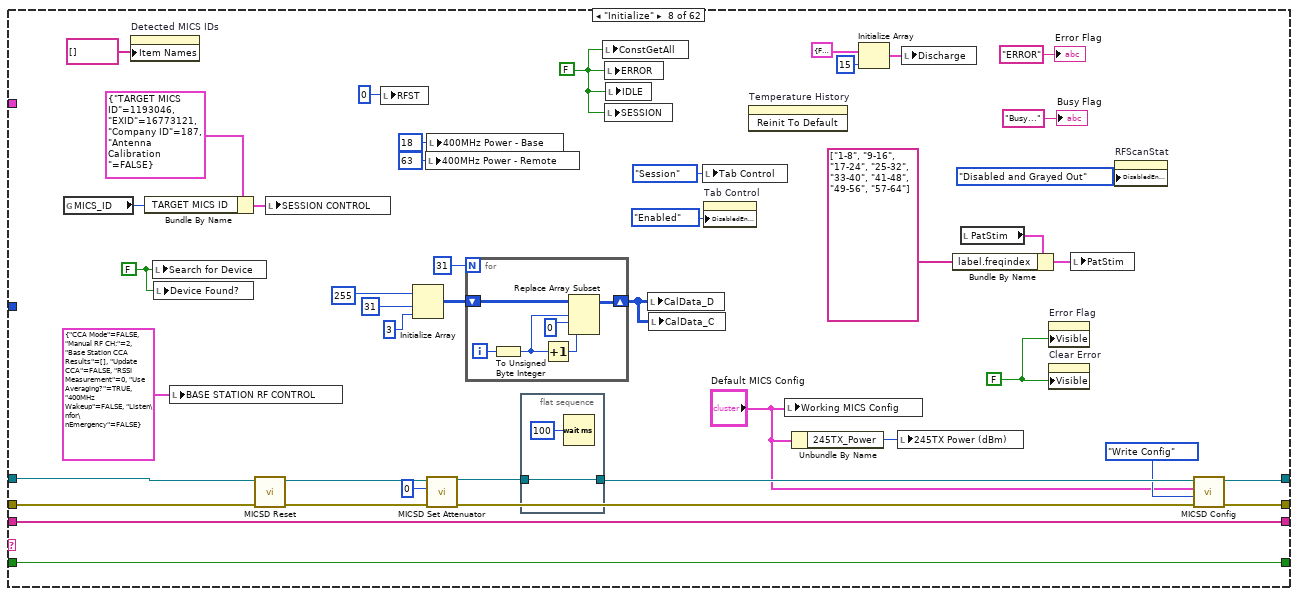
[diagram p15: hidden frame]
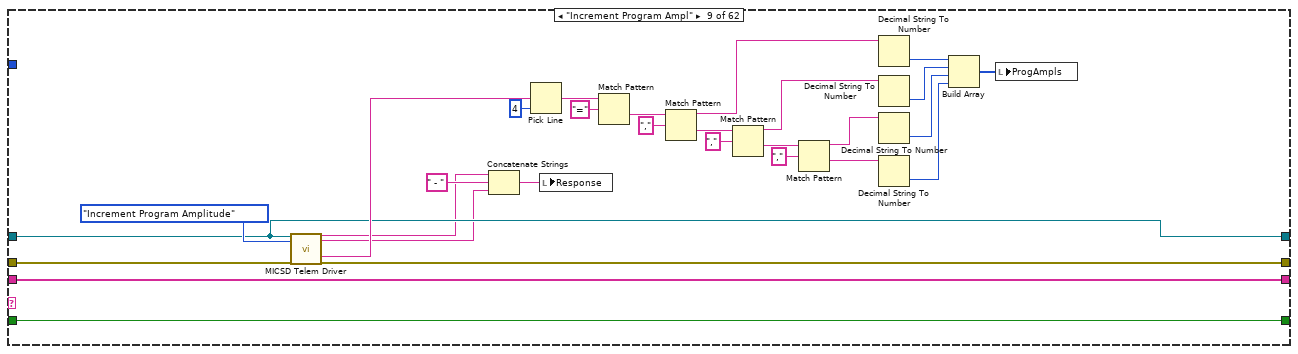
[diagram p16: hidden frame]
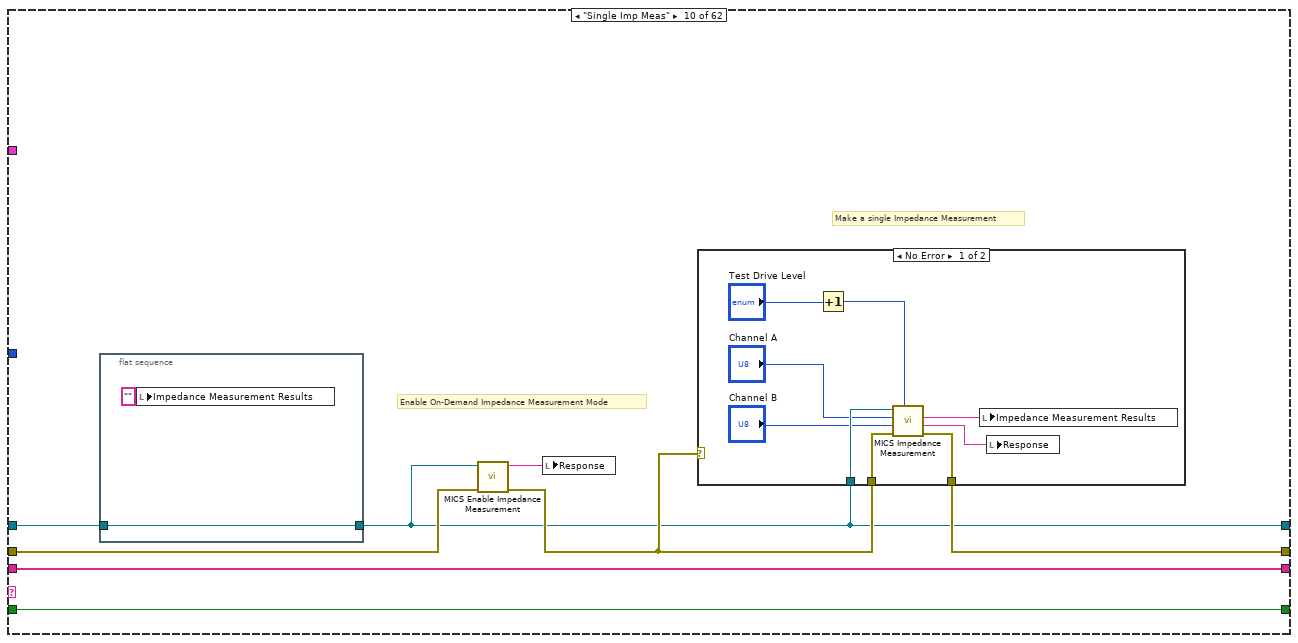
[diagram p17: hidden frame]
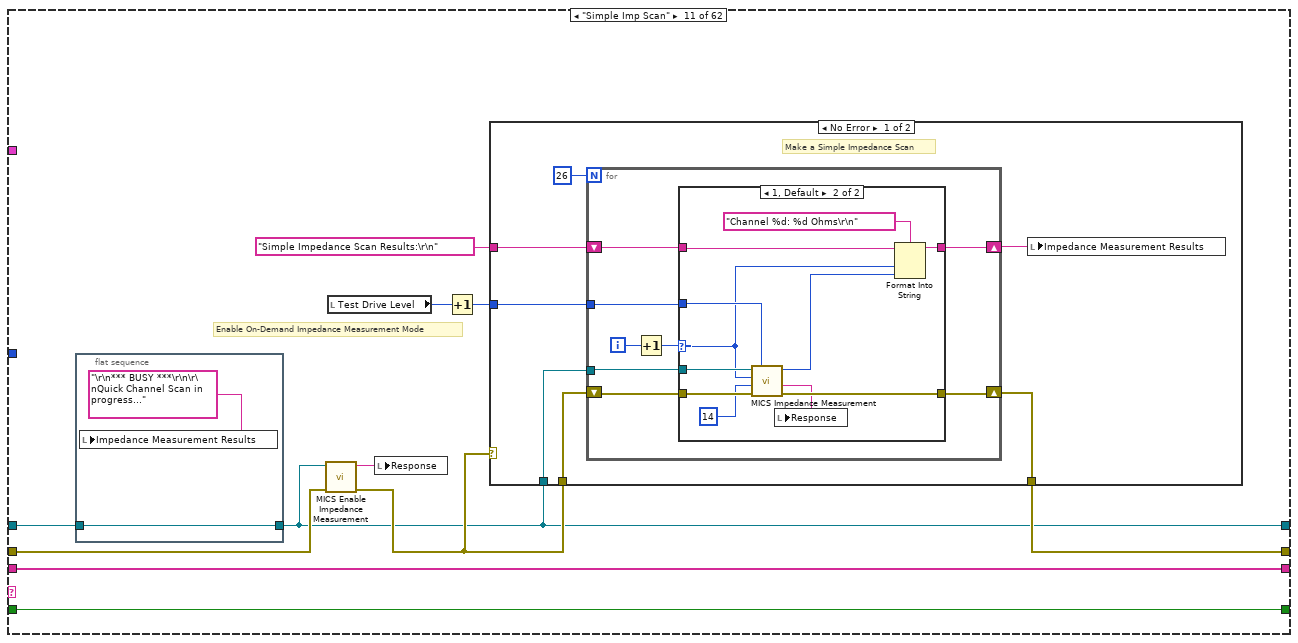
[diagram p19: hidden frame]
diagram:
  (unwired) u8 0
  (unwired) ""
  # "Wire Label"
  # "Wire Label"
  # "Wire Label"
  n1 = call-poly "VISA Configure Serial Port"("VISA resource name"="PRIMARY MICS Dongle Address", "Enable Termination\nChar (T)"=FALSE ("Enable Termination\nChar (T)"), "baud rate (9600)"=u32 230400, "error in (no error)"="error in (no error)") -> ("VISA resource name out"=w4:refnum<visa-resource-name>, "error out"=w5:errorcluster)  [unwired: 10 in]
  n2 = while {
    shift-right: [w26] -> w10
    shift-left: w5 -> [w19]
    shift-right: [w17] -> _
    shift-left: FALSE -> [w27]
    tunnel: w4 -> [w25]
    shift-right: [w20] -> _
    shift-left: string[] ["Initialize", "Clear Device Data", "Get Status"] -> [w22]
    tunnel: "Top of Loop" -> [w23]
    tunnel: [w15] -> w1
    stop <- w18 stop-if-true
    n3 = case shown="\"5s\"" "VBAT Polling Speed" {
      tunnel: [u32 3000 ("y") u32 5000 ("y") u32 10000 ("y") u32 15000 ("y")] -> w13
      frame "3s", Default {
      }
      frame "5s" {
      }
      frame "10s" {
      }
      frame "15s" {
      }
    }
    n4 = call "State Select.vi"("State In"=w23, "error in (no error)"=w19, "States Array In"=w22) -> ("State Out"=w24:string, "States Array Out"=w21:string[])  [unwired: 7 in]
    n5 = case shown="\"Top of Loop\"" w24 {
      tunnel: w27 -> [w40 w64 w73 w82 w88 _ w177 w253 w291 w299 w322 w364 w444 w458 w472 w490 w508 w526 w544 _ w626 w922 w1486 w1609 w2055 w2309 w2321 w2418 w2985 w3126 w3140 w3151 w3162 w3171 w3187 w3200 w3210 w3226 w3252 w3276 w3310 w3331 w3357 w3401 w3414 w3423 w3433 w3445 w3459 w3479 w3489 w3490 w3509 w3510 w3612 w3628 w3648 w3655 w3669 w3872 w3901 w3925]
      tunnel: [w40 w64 w73 w82 w88 FALSE w177 w253 w291 w299 w322 w364 w444 w458 w472 w490 w508 w526 w544 FALSE w626 w922 w1486 w1609 w2055 w2309 w2321 w2418 w2985 w3126 w3140 w3151 w3162 w3171 w3187 w3200 w3210 w3226 w3252 w3276 w3310 w3331 w3357 w3401 w3414 w3423 w3433 w3445 w3459 w3479 w3489 w3490 w3509 w3510 w3612 w3628 w3648 w3655 w3669 w3872 w3901 w3925] -> w17
      tunnel: w19 -> [w38 w61 w71 w79 w86 w119 w134 w219 w289 w296 w319 w361 w442 w456 w470 w488 w506 w524 w542 w574 w623 w924 w1477 w1606 w2053 w2308 w2318 w2412 w2983 w3124 w3138 w3149 w3160 w3169 w3185 w3198 w3202 w3222 w3250 w3279 w3313 w3345 w3371 w3399 w3413 w3422 w3429 w3444 w3458 w3477 w3486 w3492 w3506 w3511 w3603 w3627 w3647 w3656 w3668 _ _ _]
      tunnel: [w35 w54 w68 w78 w87 w118 w175 w223 w287 w297 w320 w362 w440 w454 w468 w486 w504 w522 w540 w575 w624 w924 w1468 w1605 w2052 w2308 w2316 w2415 w2983 w3123 w3137 w3148 w3159 w3167 w3184 w3197 w3202 w3222 w3248 w3263 w3297 w3342 w3368 w3395 w3408 w3421 w3428 w3442 w3452 w3475 w3481 w3492 w3504 w3511 w3566 w3627 w3646 w3656 _ w3874 w3902 w3926] -> w26
      tunnel: w25 -> [w33 w62 w70 w80 w85 w117 w170 w218 w267 w293 w316 w358 w420 w452 w466 w484 w502 w520 w538 w551 w615 w914 w1480 w1602 w2049 w2306 w2319 w2416 w2982 w3116 w3131 w3142 w3153 w3168 w3182 w3195 w3208 w3224 w3249 w3278 w3312 w3344 w3370 w3398 w3412 w3419 w3430 w3443 w3457 w3476 w3487 w3493 w3505 w3512 w3565 w3626 w3631 w3657 w3664 w3870 w3899 w3923]
      tunnel: w21 -> [w41 w63 w72 w81 w89 w120 w178 w254 w290 w298 w321 w363 w443 w457 w471 w489 w507 w525 w543 w576 w625 w919 w1479 w1608 w2054 w2307 w2320 w2417 w2984 w3125 w3139 w3150 w3161 w3170 w3186 w3199 w3209 w3225 w3251 w3277 w3311 w3332 w3358 w3400 w3415 w3424 w3434 w3446 w3460 w3478 w3488 w3491 w3508 _ _ _ _ _ w3665 w3871 w3900 w3924]
      tunnel: [w41 w63 w72 w81 w89 w120 w178 w254 w290 w298 w321 w363 w443 w457 w471 w489 w507 w525 w543 w576 w625 w913 w1479 w1608 w2054 w2307 w2320 w2417 w2984 w3125 w3139 w3150 w3161 w3170 w3186 w3199 w3209 w3225 w3251 w3277 w3311 w3332 w3358 w3400 w3415 w3424 w3434 w3446 w3460 w3478 w3488 w3491 w3508 w3515 string[] ["Close Session", "Discharge Control"] ("States Array Out") w3618 string[] ["Close Session", "Discharge Control"] ("States Array Out") w3654 w3665 w3871 w3900 w3924] -> w20
      tunnel: [w33 w53 w69 w77 w85 w116 w155 w222 w267 w292 w315 w357 w420 w452 w466 w484 w502 w520 w538 w573 w615 w914 w1467 w1601 w2048 w2306 w2319 w2416 w2982 w3116 w3131 w3142 w3153 w3166 w3183 w3196 w3208 w3224 w3247 w3264 w3298 w3343 w3369 w3397 w3407 w3420 w3430 w3441 w3456 w3474 w3482 w3493 w3497 w3512 w3565 w3626 w3631 w3657 w3664 w3870 w3899 w3923] -> w15
      tunnel: w13 -> [_ _ _ _ _ _ _ _ _ _ _ _ _ _ _ _ _ _ _ _ _ w905 _ _ _ _ _ _ _ _ _ _ _ _ _ _ _ _ _ _ _ _ _ _ _ _ _ _ _ _ _ _ _ _ _ _ _ _ _ _ _ _]
      tunnel: "Test Job" -> [_ _ _ _ _ _ _ _ _ _ _ _ _ _ _ _ _ _ _ _ _ _ _ _ _ _ _ _ _ _ _ _ _ _ _ _ _ _ _ _ _ _ _ _ _ _ _ _ _ _ _ _ _ _ _ _ _ _ w3667 _ _ _]
      frame "Error", Default {
        n6 = stacked-sequence {
          tunnel: w38 -> [w48]
          tunnel: [w48] -> w37
          frame #0 {
            w47 = TRUE ("Visible")
            n7 = property on="Error Flag" class="Str"("Visible"=w47) -> ()  [unwired: 2 in, 2 out]
            n8 = property on="Clear Error" class="Bool"("Visible"=w47) -> ()  [unwired: 2 in, 2 out]
            n9 = Wait (ms)(milliseconds to wait=u32 500) -> ()  [unwired: 1 out]
          }
        }
        n10 = local write "Tab Control"(T1."Session" ("Tab Control")) -> ()
        n11 = Select(t=errorcluster {"status"=FALSE, "code"=0, "source"=""}, s="Clear Error", f=w37) -> (s? t:f=w36:errorcluster)
        n12 = stacked-sequence {
          tunnel: w36 -> [w45]
          tunnel: [w45] -> w35
          tunnel: "Clear Error" -> [w43]
          frame #0 {
            n13 = Not(x=w43) -> (.not. x?=w42:bool)
            n14 = Wait (ms)(milliseconds to wait=u32 500) -> ()  [unwired: 1 out]
            n15 = property on="Clear Error" class="Bool"("Visible"=w42) -> ()  [unwired: 2 in, 2 out]
            n16 = property on="Error Flag" class="Str"("Visible"=FALSE) -> ()  [unwired: 2 in, 2 out]
          }
        }
      }
      frame "Set RF Power - Base" {
        n17 = call "MICSD Set Register.vi"("Execute on Remote?(F)"=FALSE, "error in (no error)"=w61, "Data"="400MHz Power - Base", "Address"=u16 99, "VISA Resource Name"=w62) -> ("error out"=w55:errorcluster, "dup VISA Resource Name"=w52:refnum<visa-resource-name>)  [unwired: 5 in]
        n18 = local read "Working MICS Config"() -> (w57:T20)
        n19 = Bundle By Name(cluster=w57, "245TX_Power"="245TX Power (dBm)") -> (w50:T20)
        n20 = call "MICSD Config.vi"("error in (no error)"=w55, "Function"=enum16{"Write Config", "Read Config"}."Write Config", "MICS_Config_In"=w50, "VISA Resource Name"=w52) -> ("error out"=w54:errorcluster, "dup VISA Resource Name"=w53:refnum<visa-resource-name>)  [unwired: 5 in, 1 out]
        n21 = local write "Working MICS Config"(w50) -> ()
      }
      frame "Set RF Power - Remote" {
        n22 = call "MICSD Set Register.vi"("Execute on Remote?(F)"=TRUE, "error in (no error)"=w71, "Data"="400MHz Power - Remote", "Address"=u16 99, "VISA Resource Name"=w70) -> ("error out"=w68:errorcluster, "dup VISA Resource Name"=w69:refnum<visa-resource-name>)  [unwired: 5 in]
      }
      frame "Set CW Mode" {
        n23 = call "MICSD CW Carrier.vi"("400MHz Channel"="400MHz Channel", "error in (no error)"=w79, "TX Mode (Off)"="TX Mode", "Frequency Range"="Frequency Range", "VISA Resource Name"=w80) -> ("error out"=w78:errorcluster, "dup VISA Resource Name"=w77:refnum<visa-resource-name>)  [unwired: 5 in]
      }
      frame "Telem Driver" {
        n24 = local read "STATUS FLAGS"() -> (w84:T6)
        n25 = Unbundle By Name(w84) -> ("IN_SESSION"=w83:bool)
        n26 = case shown="True" w83 {
          tunnel: [w90 w112] -> w87
          tunnel: w86 -> [w90 w109]
          tunnel: w85 -> [_ w107]
          frame False {
            n27 = One Button Dialog(message="Base Station is not in session!") -> ()  [unwired: 1 in, 1 out]
          }
          frame True {
            n28 = flat-sequence {
              tunnel: w109 -> [w113]
              tunnel: [w113] -> w108
              frame #0 {
                w114 = ""
                w115 = FALSE
                n29 = local write "bChecksum Valid"(w115) -> ()
                n30 = local write "tChecksum Valid"(w115) -> ()
                n31 = local write "Response Code"(w114) -> ()
                n32 = local write "Response Token"(w114) -> ()
                n33 = local write "Response"(w114) -> ()
                n34 = local write "Data"(w114) -> ()
              }
            }
            n35 = Unbundle By Name("SESSION CONTROL") -> ("TARGET MICS ID"=w93:u32)
            n36 = Bundle By Name(cluster=T21 {"Command"=enum."Get xPG Status", "Function"=enum."Downlink Only", "MICS_ID"=0, "EXID"=16773121, "Use Local"=FALSE, "Transceive Delay mS"=200.0, "CP_DATA IN"=[], "Parameters"=""} ("Input"), "Command"="Command", "Function"=T22."Transceive (DN -> UP)", "Parameters"="Parameters", "CP_DATA IN"="CP_DATA IN", "MICS_ID"=w93) -> (w102:T21)
            n37 = call "Zarlink Telemetry.vi"("error in (no error)"=w108, "Input"=w102, "MICS Dongle Address"=w107) -> ("error out"=w112:errorcluster, "Output"=w101:T28)  [unwired: 6 in, 1 out]
            n38 = Unbundle By Name(w101) -> ("Response Token"=w96:string, "Response Code"=w95:string, "bChecksum Valid"=→"bChecksum Valid":bool, "tChecksum Valid"=→"tChecksum Valid":bool, "Data"=→"Data":string, "CP_DATA OUT"=→"CP_DATA OUT":u8[])
            "Response Token" <- w96
            "Response Code" <- w95
            n39 = Concatenate Strings(w96, " - ", w95) -> (w111:string)
            n40 = local write "Response"(w111) -> ()
          }
        }
      }
      frame "Close Session" {
        n41 = call "MICSD Abort.vi"("error in (no error)"=w119, "VISA Resource Name"=w117) -> ("error out"=w118:errorcluster, "dup VISA Resource Name"=w116:refnum<visa-resource-name>)  [unwired: 8 in]
      }
      frame "Open Session" {
        n42 = local read "Default MICS Config"() -> (w143:T20)
        n43 = local read "BASE STATION RF CONTROL"() -> (w162:T2)
        n44 = local read "SESSION CONTROL"() -> (w154:T3)
        n45 = stacked-sequence {
          tunnel: w134 -> [w181]
          tunnel: [w181] -> w133
          frame #0 {
            n46 = local write "Time to Open Session, Secs"(nan ("Time to Open Session, Secs")) -> ()
            n47 = property on="Time to Open Session, Secs" class="DigNum (strict)"("NumText.BGColor"=u32 16772882) -> ()  [unwired: 2 in, 2 out]
          }
        }
        n48 = Unbundle By Name(w162) -> ("Listen\nfor\nEmergency"=w157:bool, "400MHz Wakeup"=w156:bool, "CCA Mode"=w161:bool, "Manual RF CH:"=w140:u8)
        n49 = Unbundle By Name(w143) -> ("245TX_Power"=w142:i8, "245TX_PowerCal"=w141:i8)
        n50 = Unbundle By Name(w154) -> ("Antenna Calibration"=w153:bool)
        n51 = Unbundle By Name(w154) -> ("TARGET MICS ID"=w171:u32, "Company ID"=w172:u8)
        n52 = Select(t=u8 1, s=w157, f=u8 0) -> (s? t:f=w158:u8)
        n53 = Select(t=u8 8, s=w156, f=u8 0) -> (s? t:f=w164:u8)
        n54 = Select(t=u8 4, s=w161, f=u8 0) -> (s? t:f=w163:u8)
        n55 = case shown="True" w153 {
          tunnel: [w182 w184] -> w151
          tunnel: w133 -> [w182 w191]
          tunnel: w170 -> [w183 w190]
          tunnel: w140 -> [_ w189]
          tunnel: [w183 w186] -> w152
          frame False {
            # "DO NOT\nCALIBRATE ANTENNA!"
          }
          frame True {
            # "CALIBRATE ANTENNA\nFOR INTENDED CHANNEL"
            n56 = call "MICSD Calibrate.vi"("VISA Resource Name"=w190, "CalSelect1"=u8 64, "Channel"=w189, "error in (no error)"=w191) -> ("dup VISA Resource Name"=w187:refnum<visa-resource-name>, "error out"=w185:errorcluster)  [unwired: 10 in]
            n57 = stacked-sequence {
              tunnel: w187 -> [w193]
              tunnel: [w193] -> w186
              tunnel: w185 -> [w192]
              tunnel: [w192] -> w184
              frame #0 {
                n58 = Wait (ms)(milliseconds to wait=u32 200) -> ()  [unwired: 1 out]
              }
            }
          }
        }
        n59 = Compound Arithmetic op=OR(w158, w164, w163) -> (w165:u8)
        n60 = local read "Working MICS Config"() -> (w150:T20)
        n61 = Bundle By Name(cluster=w150, "ConfigFlags"=w165, "Normal_Comm.RF_Channel"=w140, "ImplantID"=w171, "CompanyID"=w172, "245TX_Power"=w142, "245TX_PowerCal"=w141) -> (w173:T20)
        "Working MICS Config" <- w173
        n62 = call "MICSD Config.vi"("error in (no error)"=w151, "Function"=enum16{"Write Config", "Read Config"}."Write Config", "MICS_Config_In"=w173, "VISA Resource Name"=w152) -> ("error out"=w176:errorcluster, "dup VISA Resource Name"=w155:refnum<visa-resource-name>)  [unwired: 5 in, 1 out]
        n63 = Tick Count (ms)() -> (millisecond timer value=w139:u32)
        n64 = case shown="False" w157 {
          tunnel: w176 -> [w206 w211]
          tunnel: w155 -> [w205 _]
          tunnel: [w199 w211] -> w175
          tunnel: "Wait Time (S)" -> [w202 _]
          tunnel: "Enable WD?" -> [w201 _]
          tunnel: w139 -> [w198 _]
          tunnel: [w198 w210] -> w137
          tunnel: [w197 w210] -> w138
          tunnel: [w195 FALSE ("IN_SESSION")] -> w130
          frame False {
            # "Listen for Emergency was not selected"
            n65 = call "MICSD Start Session.vi"("error in (no error)"=w206, "Enable Watchdog?(T)"=w201, "Wait Time (S)"=w202, "VISA Resource Name"=w205) -> ("error out"=w204:errorcluster, "dup VISA Resource Name"=w203:refnum<visa-resource-name>)  [unwired: 6 in]
            n66 = call "MICSD Status.vi"("VISA Resource Name"=w203, "error in (no error)"=w204) -> ("Status Flags"=w196:T6, "error out"=w200:errorcluster)  [unwired: 7 in, 5 out]
            n67 = local write "STATUS FLAGS"(w196) -> ()
            n68 = Unbundle By Name(w196) -> ("IN_SESSION"=w195:bool)
            n69 = stacked-sequence {
              tunnel: w200 -> [w208]
              tunnel: [w208] -> w199
              tunnel: [w207] -> w197
              frame #0 {
                n70 = Tick Count (ms)() -> (millisecond timer value=w207:u32)
              }
            }
          }
          frame True {
            w210 = u32 0 ("millisecond timer value")
            # "Listen for Emergency was selected, \ndo not open a session"
          }
        }
        n71 = local read "STATUS FLAGS"() -> (w146:T6)
        n72 = local write "VBAT Cal"(0.0 ("VBAT Cal")) -> ()
        n73 = Bundle By Name(cluster=w146, "STARTING_SESSION"=TRUE) -> (w145:T6)
        n74 = Subtract(x=w138, y=w137) -> (x-y=w136:u32)
        n75 = Divide(x=w136, y=u32 1000) -> (x/y=w124:dbl)
        n76 = Less?(x=w124, y=1.0) -> (x < y?=w122:bool)
        n77 = local write "STATUS FLAGS"(w145) -> ()
        n78 = invoke on="Temperature History" class="WFChart (strict)" method="Reinit To Default"() -> ()  [unwired: 3 in, 3 out]
        n79 = Select(t=u32 6618880, s=w122, f=u32 16772882) -> (s? t:f=w127:u32)
        n80 = Select(t=w124, s=w130, f=nan ("Time to Open Session, Secs")) -> (s? t:f=→"Time to Open Session, Secs":dbl)
        n81 = Select(t=w127, s=w130, f=u32 16711680) -> (s? t:f=w131:u32)
        n82 = property on="Time to Open Session, Secs" class="DigNum (strict)"("NumText.BGColor"=w131) -> ()  [unwired: 2 in, 2 out]
      }
      frame "Initialize" {
        w227 = FALSE ("Device Found?")
        w252 = FALSE ("Visible")
        w229 = FALSE
        n83 = global read "MICS_ID Global.vi" "MICS_ID"() -> (w242:u32)
        n84 = property on="Detected MICS IDs" class="LstBox (strict)"("Item Names"=string[] []) -> ()  [unwired: 2 in, 2 out]
        n85 = Bundle By Name(cluster=T3 {"TARGET MICS ID"=1193046, "EXID"=16773121, "Company ID"=187, "Antenna Calibration "=FALSE} ("SESSION CONTROL"), "TARGET MICS ID"=w242) -> (w243:T3)
        n86 = local write "Search for Device"(w227) -> ()
        n87 = local write "Device Found?"(w227) -> ()
        n88 = local write "BASE STATION RF CONTROL"(T2 {"CCA Mode"=FALSE, "Manual RF CH:"=2, "Base Station CCA Results"=[], "Update CCA"=FALSE, "RSSI Measurement"=0, "Use Averaging?"=TRUE, "400MHz Wakeup"=FALSE, "Listen\nfor\nEmergency"=FALSE} ("Base Station RF Control")) -> ()
        n89 = call "MICSD Reset.vi"("error in (no error)"=w219, "VISA Resource Name"=w218) -> ("error out"=w217:errorcluster, "dup VISA Resource Name"=w216:refnum<visa-resource-name>)  [unwired: 8 in]
        n90 = local write "SESSION CONTROL"(w243) -> ()
        n91 = local write "RFST"(u16 0) -> ()
        n92 = Initialize Array(u8 255, 31 ("dimension size"), 3 ("dimension size")) -> (w233:u8[][])
        n93 = local write "400MHz Power - Remote"(u8 63 ("400MHz Power - Remote")) -> ()
        n94 = local write "400MHz Power - Base"(u8 18 ("400MHz Power - Base")) -> ()
        n95 = call "MICSD Set Attenuator.vi"("error in (no error)"=w217, "Attenuation"=u8 0, "VISA Resource Name"=w216) -> ("error out"=w225:errorcluster, "dup VISA Resource Name"=w245:refnum<visa-resource-name>)  [unwired: 7 in]
        n96 = for {
          N: 31 -> [_]
          shift-right: [w260] -> w234
          shift-left: w233 -> [w259]
          i -> [w256]
          n97 = To Unsigned Byte Integer(number=w256) -> (unsigned 8bit integer=w255:u8)
          n98 = Increment(x=w255) -> (x+1=w258:u8)
          n99 = Replace Array Subset(array=w259, new element=w258, index (row)=w255, index (col)=0 ("disabled index (row)")) -> (w260:u8[][])
        }
        n100 = flat-sequence {
          tunnel: w245 -> [w262]
          tunnel: [w262] -> w224
          frame #0 {
            n101 = Wait (ms)(milliseconds to wait=u32 100) -> ()  [unwired: 1 out]
          }
        }
        n102 = local write "ConstGetAll"(w229) -> ()
        n103 = local write "ERROR"(w229) -> ()
        n104 = local write "SESSION"(w229) -> ()
        n105 = local write "IDLE"(w229) -> ()
        n106 = local write "CalData_D"(w234) -> ()
        n107 = local write "CalData_C"(w234) -> ()
        n108 = local write "Tab Control"(T1."Session" ("Tab Control")) -> ()
        n109 = property on="Tab Control" class="TabCtl (strict)"("DisabledEnum"=T23."Enabled" ("Disabled")) -> ()  [unwired: 2 in, 2 out]
        n110 = invoke on="Temperature History" class="WFChart (strict)" method="Reinit To Default"() -> ()  [unwired: 3 in, 3 out]
        n111 = local write "Working MICS Config"("Default MICS Config") -> ()
        n112 = Unbundle By Name("Default MICS Config") -> ("245TX_Power"=w241:i8)
        n113 = Initialize Array(T24 {"Activate"=FALSE, "Stop"=FALSE, "VBAT"=0.0, "Discharging"=FALSE, "Ready"=FALSE, "MICS ID"=0} ("Channel"), 15 ("dimension size")) -> (w238:T9)
        n114 = local write "245TX Power (dBm)"(w241) -> ()
        n115 = local write "Discharge"(w238) -> ()
        n116 = local read "PatStim"() -> (w248:T10)
        n117 = Bundle By Name(cluster=w248, "label.freqindex"=string[] ["1-8", "9-16", "17-24", "25-32", "33-40", "41-48", "49-56", "57-64"]) -> (w249:T10)
        n118 = property on="Error Flag" class="Str"("Visible"=w252) -> ()  [unwired: 2 in, 2 out]
        n119 = property on="Clear Error" class="Bool"("Visible"=w252) -> ()  [unwired: 2 in, 2 out]
        n120 = local write "PatStim"(w249) -> ()
        n121 = property on="RFScanStat" class="Clust (strict)"("DisabledEnum"=T23."Disabled and Grayed Out" ("Disabled")) -> ()  [unwired: 2 in, 2 out]
        n122 = call "MICSD Config.vi"("error in (no error)"=w225, "Function"=enum16{"Write Config", "Read Config"}."Write Config", "MICS_Config_In"="Default MICS Config", "VISA Resource Name"=w224) -> ("error out"=w223:errorcluster, "dup VISA Resource Name"=w222:refnum<visa-resource-name>)  [unwired: 5 in, 1 out]
        "Error Flag" <- "ERROR" ("Error Flag")
        "Busy Flag" <- "Busy..." ("Busy Flag")
      }
      frame "Increment Program Ampl" {
        n123 = call "MICSD Telem Driver.vi"("VISA Resource Name"=w267, "Command"=Typedef_Command_List."Increment Program Amplitude", "error in (no error)"=w289) -> ("Response Token"=w264:string, "Response Code"=w263:string, "Data"=w268:string, "error out"=w287:errorcluster)  [unwired: 10 in, 3 out]
        n124 = Concatenate Strings(w264, " - ", w263) -> (w265:string)
        n125 = Pick Line(multi-line string=w268, line index=4) -> (output string=w284:string)  [unwired: 1 in]
        n126 = local write "Response"(w265) -> ()
        n127 = Match Pattern(string=w284, regular expression="=") -> (after substring=w282:string)  [unwired: 1 in, 3 out]
        n128 = Match Pattern(string=w282, regular expression=",") -> (before substring=w281:string, after substring=w280:string)  [unwired: 1 in, 2 out]
        n129 = Match Pattern(string=w280, regular expression=",") -> (before substring=w276:string, after substring=w277:string)  [unwired: 1 in, 2 out]
        n130 = Match Pattern(string=w277, regular expression=",") -> (before substring=w275:string, after substring=w274:string)  [unwired: 1 in, 2 out]
        n131 = Decimal String To Number(string=w281) -> (number=w273:i32)  [unwired: 2 in, 1 out]
        n132 = Decimal String To Number(string=w276) -> (number=w272:i32)  [unwired: 2 in, 1 out]
        n133 = Decimal String To Number(string=w275) -> (number=w271:i32)  [unwired: 2 in, 1 out]
        n134 = Decimal String To Number(string=w274) -> (number=w270:i32)  [unwired: 2 in, 1 out]
        n135 = Build Array(w273, w272, w271, w270) -> (w269:i32[])
        n136 = local write "ProgAmpls"(w269) -> ()
      }
      frame "Single Imp Meas" {
        # "Enable On-Demand Impedance Measurement Mode"
        # "Make a single Impedance Measurement"
        n137 = flat-sequence {
          tunnel: w293 -> [w300]
          tunnel: [w300] -> w292
          frame #0 {
            n138 = local write "Impedance Measurement Results"("" ("Impedance Measurement Results")) -> ()
          }
        }
        n139 = call "MICS Enable Impedance Measurement.vi"("error in"=w296, "VISA resource name in"=w292) -> ("error out"=w295:errorcluster, "Response"=w294:string)  [unwired: 8 in]
        n140 = local write "Response"(w294) -> ()
        n141 = case shown="No Error" w295 {
          tunnel: [w309 w311] -> w297
          tunnel: w292 -> [w308 _]
          tunnel: w295 -> [w304 w311]
          frame No Error {
            n142 = Increment(x="Test Drive Level") -> (x+1=w305:enum16{"Low (200uA)", "High (500uA)"})
            n143 = call "MICS Impedance Measurement.vi"("Test Current"=w305, "error in"=w304, "Channel B"="Channel B", "Channel A"="Channel A", "VISA resource name in"=w308) -> ("error out"=w309:errorcluster, "Response Data"=w303:string, "Text Out"=w302:string)  [unwired: 3 in, 1 out]
            n144 = local write "Impedance Measurement Results"(w302) -> ()
            n145 = local write "Response"(w303) -> ()
          }
          frame Error {
          }
        }
      }
      frame "Simple Imp Scan" {
        # "Enable On-Demand Impedance Measurement Mode"
        n146 = flat-sequence {
          tunnel: w316 -> [w323]
          tunnel: [w323] -> w315
          frame #0 {
            n147 = local write "Impedance Measurement Results"("\r\n*** BUSY ***\r\n\r\nQuick Channel Scan in progress..." ("Impedance Measurement Results")) -> ()
          }
        }
        n148 = call "MICS Enable Impedance Measurement.vi"("error in"=w319, "VISA resource name in"=w315) -> ("error out"=w318:errorcluster, "Response"=w317:string)  [unwired: 8 in]
        n149 = local read "Test Drive Level"() -> (w314:enum16{"Low (200uA)", "High (500uA)"})
        n150 = local write "Response"(w317) -> ()
        n151 = Increment(x=w314) -> (x+1=w313:enum16{"Low (200uA)", "High (500uA)"})
        n152 = case shown="No Error" w318 {
          tunnel: [w331 w353] -> w320
          tunnel: w315 -> [w330 _]
          tunnel: w318 -> [w329 w353]
          tunnel: w313 -> [w328 _]
          tunnel: "Simple Impedance Scan Results:\r\n" ("Impedance Measurement Results") -> [w326 _]
          frame No Error {
            # "Make a Simple Impedance Scan"
            n153 = for {
              N: 26 -> [_]
              tunnel: w330 -> [w338]
              tunnel: w328 -> [w336]
              shift-right: [w339] -> w331
              shift-left: w329 -> [w337]
              shift-right: [w332] -> w325
              shift-left: w326 -> [w333]
              i -> [w335]
              n154 = Increment(x=w335) -> (x+1=w334:i32)
              n155 = case shown="1, Default" w334 {
                selector: w334 -> [_ w343]
                tunnel: [w341 w352] -> w339
                tunnel: w338 -> [_ w351]
                tunnel: w337 -> [w341 w350]
                tunnel: w336 -> [_ w348]
                tunnel: w333 -> [w340 w345]
                tunnel: [w340 w346] -> w332
                frame 14 {
                }
                frame 1, Default {
                  n156 = call "MICS Impedance Measurement.vi"("Test Current"=w348, "error in"=w350, "Channel B"=u8 14, "Channel A"=w343, "VISA resource name in"=w351) -> ("error out"=w352:errorcluster, "Response Data"=w349:string, "Impedance (Ohms)"=w342:u16)  [unwired: 3 in, 1 out]
                  n157 = local write "Response"(w349) -> ()
                  n158 = Format Into String(format string="Channel %d: %d Ohms\r\n", initial string=w345, w343, w342) -> (resulting string=w346:string)  [unwired: 1 in, 1 out]
                }
              }
            }
            n159 = local write "Impedance Measurement Results"(w325) -> ()
          }
          frame Error {
          }
        }
      }
      frame "Matrix Imp Scan" {
        # "Enable On-Demand Impedance Measurement Mode"
        n160 = flat-sequence {
          tunnel: w358 -> [w365]
          tunnel: [w365] -> w357
          frame #0 {
            n161 = local write "Impedance Measurement Results"("" ("Impedance Measurement Results")) -> ()
          }
        }
        n162 = local read "Test Drive Level"() -> (w356:enum16{"Low (200uA)", "High (500uA)"})
        n163 = call "MICS Enable Impedance Measurement.vi"("error in"=w361, "VISA resource name in"=w357) -> ("error out"=w360:errorcluster, "Response"=w359:string)  [unwired: 8 in]
        n164 = local write "Response"(w359) -> ()
        n165 = Increment(x=w356) -> (x+1=w355:enum16{"Low (200uA)", "High (500uA)"})
        n166 = case shown="No Error" w360 {
          tunnel: [w373 w415] -> w362
          tunnel: w357 -> [w372 _]
          tunnel: w360 -> [w371 w415]
          tunnel: w355 -> [w370 _]
          tunnel: "Matrix Impedance Scan Results (in Ohms):\r\n     ,CH01,CH02,CH03,CH04,CH05,CH06,CH07,CH08,CH09,CH10,CH11,CH12,CH13,CH14,CH15,CH16,CH17,CH18,CH19,CH20,CH21,CH22,CH23,CH24,CH25,CH26\r\n" ("Impedance Measurement Results") -> [w368 _]
          frame No Error {
            # "Make a Matrix Impedance Scan"
            n167 = for {
              N: 26 -> [_]
              tunnel: w372 -> [w389]
              tunnel: w370 -> [w387]
              shift-right: [w390] -> w373
              shift-left: w371 -> [w388]
              shift-right: [w382] -> w367
              shift-left: w368 -> [w381]
              i -> [w385]
              n168 = Increment(x=w385) -> (x+1=w376:i32)
              n169 = Number To Decimal String(number=w376, width (-)=i16 2) -> (decimal integer string=w377:string)
              n170 = Format Into String(format string="CH%s:,", initial string=w381, w377) -> (resulting string=w380:string)  [unwired: 1 in, 1 out]
              n171 = for {
                N: 26 -> [_]
                tunnel: w389 -> [w401]
                tunnel: w387 -> [w399]
                shift-right: [w402] -> w390
                shift-left: w388 -> [w400]
                tunnel: w376 -> [w395]
                shift-right: [w392] -> w384
                shift-left: w380 -> [w393]
                i -> [w398]
                n172 = Increment(x=w398) -> (x+1=w396:i32)
                n173 = Equal?(x=w396, y=w395) -> (x = y?=w397:bool)
                n174 = case shown="False" w397 {
                  tunnel: [w404 w414] -> w402
                  tunnel: w401 -> [_ w413]
                  tunnel: w400 -> [w404 w412]
                  tunnel: w399 -> [_ w410]
                  tunnel: w396 -> [_ w409]
                  tunnel: w395 -> [_ w408]
                  tunnel: [" N/A" w406] -> w394
                  frame True {
                  }
                  frame False {
                    n175 = call "MICS Impedance Measurement.vi"("Test Current"=w410, "error in"=w412, "Channel B"=w408, "Channel A"=w409, "VISA resource name in"=w413) -> ("error out"=w414:errorcluster, "Response Data"=w411:string, "Impedance (Ohms)"=w407:u16)  [unwired: 3 in, 1 out]
                    n176 = local write "Response"(w411) -> ()
                    n177 = Number To Decimal String(number=w407, width (-)=i16 4) -> (decimal integer string=w406:string)
                  }
                }
                n178 = Concatenate Strings(w393, w394, ",") -> (w392:string)
              }
              n179 = Format Into String(format string="\r\n*** BUSY ***\r\n\r\nScanning Row %d of 26...", w376) -> (resulting string=w374:string)  [unwired: 2 in, 1 out]
              n180 = local write "Impedance Measurement Results"(w374) -> ()
              n181 = Concatenate Strings(w384, "\r\n") -> (w382:string)
            }
            n182 = local write "Impedance Measurement Results"(w367) -> ()
          }
          frame Error {
          }
        }
      }
      frame "Decrement Program Ampl" {
        n183 = call "MICSD Telem Driver.vi"("VISA Resource Name"=w420, "Command"=Typedef_Command_List."Decrement Program Amplitude", "error in (no error)"=w442) -> ("Response Token"=w417:string, "Response Code"=w418:string, "Data"=w421:string, "error out"=w440:errorcluster)  [unwired: 10 in, 3 out]
        n184 = Concatenate Strings(w417, " - ", w418) -> (w416:string)
        n185 = Pick Line(multi-line string=w421, line index=4) -> (output string=w437:string)  [unwired: 1 in]
        n186 = local write "Response"(w416) -> ()
        n187 = Match Pattern(string=w437, regular expression="=") -> (after substring=w435:string)  [unwired: 1 in, 3 out]
        n188 = Match Pattern(string=w435, regular expression=",") -> (before substring=w434:string, after substring=w433:string)  [unwired: 1 in, 2 out]
        n189 = Match Pattern(string=w433, regular expression=",") -> (before substring=w429:string, after substring=w430:string)  [unwired: 1 in, 2 out]
        n190 = Match Pattern(string=w430, regular expression=",") -> (before substring=w428:string, after substring=w427:string)  [unwired: 1 in, 2 out]
        n191 = Decimal String To Number(string=w434) -> (number=w426:i32)  [unwired: 2 in, 1 out]
        n192 = Decimal String To Number(string=w429) -> (number=w425:i32)  [unwired: 2 in, 1 out]
        n193 = Decimal String To Number(string=w428) -> (number=w424:i32)  [unwired: 2 in, 1 out]
        n194 = Decimal String To Number(string=w427) -> (number=w423:i32)  [unwired: 2 in, 1 out]
        n195 = Build Array(w426, w425, w424, w423) -> (w422:i32[])
        n196 = local write "ProgAmpls"(w422) -> ()
      }
      frame "Increment Program Freq" {
        n197 = call "MICSD Telem Driver.vi"("VISA Resource Name"=w452, "Command"=Typedef_Command_List."Increment Program Frequency", "error in (no error)"=w456) -> ("Response Token"=w449:string, "Response Code"=w450:string, "Data"=w445:string, "error out"=w454:errorcluster)  [unwired: 10 in, 3 out]
        n198 = Concatenate Strings(w449, " - ", w450) -> (w448:string)
        n199 = local write "Response"(w448) -> ()
        n200 = Match Pattern(string=w445, regular expression="=") -> (after substring=w447:string)  [unwired: 1 in, 3 out]
        n201 = Decimal String To Number(string=w447) -> (number=w446:i32)  [unwired: 2 in, 1 out]
        n202 = local write "Freq Index"(w446) -> ()
      }
      frame "Decrement Program Freq" {
        n203 = call "MICSD Telem Driver.vi"("VISA Resource Name"=w466, "Command"=Typedef_Command_List."Decrement Program Frequency", "error in (no error)"=w470) -> ("Response Token"=w463:string, "Response Code"=w464:string, "Data"=w459:string, "error out"=w468:errorcluster)  [unwired: 10 in, 3 out]
        n204 = Concatenate Strings(w463, " - ", w464) -> (w462:string)
        n205 = local write "Response"(w462) -> ()
        n206 = Match Pattern(string=w459, regular expression="=") -> (after substring=w461:string)  [unwired: 1 in, 3 out]
        n207 = Decimal String To Number(string=w461) -> (number=w460:i32)  [unwired: 2 in, 1 out]
        n208 = local write "Freq Index"(w460) -> ()
      }
      frame "PulseWidthUp" {
        n209 = Number To Decimal String(number="Pulse #") -> (decimal integer string=w477:string)  [unwired: 1 in]
        n210 = Concatenate Strings("PulseIndex=", w477) -> (w475:string)
        n211 = call "MICSD Telem Driver.vi"("VISA Resource Name"=w484, "Command"=Typedef_Command_List."Increment Pulse Width", "Parameters"=w475, "error in (no error)"=w488) -> ("Response Token"=w481:string, "Response Code"=w482:string, "Data"=w478:string, "error out"=w486:errorcluster)  [unwired: 9 in, 3 out]
        n212 = Concatenate Strings(w481, " - ", w482) -> (w480:string)
        n213 = local write "Response"(w480) -> ()
        n214 = Match Pattern(string=w478, regular expression="=") -> (after substring=w479:string)  [unwired: 1 in, 3 out]
        n215 = Decimal String To Number(string=w479) -> (number=w473:i32)  [unwired: 2 in, 1 out]
        n216 = local write "PulsePW"(w473) -> ()
      }
      frame "PulseWidthDown" {
        n217 = local read "Pulse #"() -> (w492:u8)
        n218 = Number To Decimal String(number=w492) -> (decimal integer string=w495:string)  [unwired: 1 in]
        n219 = Concatenate Strings("PulseIndex=", w495) -> (w493:string)
        n220 = call "MICSD Telem Driver.vi"("VISA Resource Name"=w502, "Command"=Typedef_Command_List."Decrement Pulse Width", "Parameters"=w493, "error in (no error)"=w506) -> ("Response Token"=w499:string, "Response Code"=w500:string, "Data"=w496:string, "error out"=w504:errorcluster)  [unwired: 9 in, 3 out]
        n221 = Concatenate Strings(w499, " - ", w500) -> (w498:string)
        n222 = local write "Response"(w498) -> ()
        n223 = Match Pattern(string=w496, regular expression="=") -> (after substring=w497:string)  [unwired: 1 in, 3 out]
        n224 = Decimal String To Number(string=w497) -> (number=w491:i32)  [unwired: 2 in, 1 out]
        n225 = local write "PulsePW"(w491) -> ()
      }
      frame "PulseAmplUp" {
        n226 = local read "Pulse #"() -> (w510:u8)
        n227 = Number To Decimal String(number=w510) -> (decimal integer string=w513:string)  [unwired: 1 in]
        n228 = Concatenate Strings("PulseIndex=", w513) -> (w511:string)
        n229 = call "MICSD Telem Driver.vi"("VISA Resource Name"=w520, "Command"=Typedef_Command_List."Increment Pulse Amplitude", "Parameters"=w511, "error in (no error)"=w524) -> ("Response Token"=w517:string, "Response Code"=w518:string, "Data"=w514:string, "error out"=w522:errorcluster)  [unwired: 9 in, 3 out]
        n230 = Concatenate Strings(w517, " - ", w518) -> (w516:string)
        n231 = local write "Response"(w516) -> ()
        n232 = Match Pattern(string=w514, regular expression="=") -> (after substring=w515:string)  [unwired: 1 in, 3 out]
        n233 = Decimal String To Number(string=w515) -> (number=w509:i32)  [unwired: 2 in, 1 out]
        n234 = local write "PulseAmpl"(w509) -> ()
      }
      frame "PulseAmplDown" {
        n235 = local read "Pulse #"() -> (w528:u8)
        n236 = Number To Decimal String(number=w528) -> (decimal integer string=w531:string)  [unwired: 1 in]
        n237 = Concatenate Strings("PulseIndex=", w531) -> (w529:string)
        n238 = call "MICSD Telem Driver.vi"("VISA Resource Name"=w538, "Command"=Typedef_Command_List."Decrement Pulse Amplitude", "Parameters"=w529, "error in (no error)"=w542) -> ("Response Token"=w535:string, "Response Code"=w536:string, "Data"=w532:string, "error out"=w540:errorcluster)  [unwired: 9 in, 3 out]
        n239 = Concatenate Strings(w535, " - ", w536) -> (w534:string)
        n240 = local write "Response"(w534) -> ()
        n241 = Match Pattern(string=w532, regular expression="=") -> (after substring=w533:string)  [unwired: 1 in, 3 out]
        n242 = Decimal String To Number(string=w533) -> (number=w527:i32)  [unwired: 2 in, 1 out]
        n243 = local write "PulseAmpl"(w527) -> ()
      }
      frame "Search for Device" {
        n244 = local read "SESSION CONTROL"() -> (w570:T3)
        n245 = local read "BASE STATION RF CONTROL"() -> (w559:T2)
        n246 = Unbundle By Name(w559) -> ("Listen\nfor\nEmergency"=w553:bool, "400MHz Wakeup"=w547:bool, "CCA Mode"=w558:bool, "Manual RF CH:"=w557:u8)
        n247 = stacked-sequence {
          tunnel: w574 -> [w607]
          tunnel: [w607] -> w550
          frame #0 {
            w603 = FALSE ("Device Found?")
            n248 = local read "STATUS FLAGS"() -> (w606:T6)
            n249 = Bundle By Name(cluster=w606, "SLEEPING"=w603, "IDLE"=w603, "SEARCHING_FOR_IMPLANT"=TRUE ("Device Found?"), "STARTING_SESSION"=w603, "LISTENING_FOR_EMERG"=w603, "IN_SESSION"=w603) -> (w605:T6)
            n250 = local write "ERROR"(w603) -> ()
            n251 = local write "SESSION"(w603) -> ()
            n252 = local write "IDLE"(w603) -> ()
            n253 = local write "Device Found?"(FALSE ("Device Found?")) -> ()
            n254 = local write "STATUS FLAGS"(w605) -> ()
          }
        }
        n255 = Unbundle By Name(w570) -> ("TARGET MICS ID"=w568:u32, "Company ID"=w569:u8)
        n256 = Select(t=u8 1, s=w553, f=u8 0) -> (s? t:f=w554:u8)
        n257 = Select(t=u8 8, s=w547, f=u8 0) -> (s? t:f=w561:u8)
        n258 = Select(t=u8 4, s=w558, f=u8 0) -> (s? t:f=w560:u8)
        n259 = Decrement(x=w557) -> (x-1=w567:u8)
        n260 = Compound Arithmetic op=OR(w554, w561, w560) -> (w562:u8)
        n261 = local read "Default MICS Config"() -> (w552:T20)
        n262 = Bundle By Name(cluster=w552, "ConfigFlags"=w562, "Normal_Comm.RF_Channel"=w567, "ImplantID"=w568, "CompanyID"=w569) -> (w571:T20)
        n263 = call "MICSD Config.vi"("error in (no error)"=w550, "Function"=enum16{"Write Config", "Read Config"}."Write Config", "MICS_Config_In"=w571, "VISA Resource Name"=w551) -> ("error out"=w548:errorcluster, "dup VISA Resource Name"=w549:refnum<visa-resource-name>)  [unwired: 5 in, 1 out]
        n264 = while {
          tunnel: [w598] -> w573
          tunnel: w549 -> [w595]
          tunnel: w547 -> [w592]
          shift-right: [w588] -> _
          shift-left: T25."Start Search" ("Mode") -> [w586]
          shift-right: [w582] -> w575
          shift-left: w548 -> [w594]
          tunnel: "Dwell Time (mS)" -> [w578]
          stop <- w583 stop-if-true
          w587 = T25."End Search" ("Mode")
          w593 = FALSE  # Any Company?(T)
          # "Make the first ID found the default target."
          n265 = call "MICSD Search for Implant.vi"("VISA Resource Name"=w595, "Search Time (mS)"=w578, "Enable Watchdog?(T)"=w592, "Any Company?(T)"=w593, "error in (no error)"=w594, "Mode"=w586) -> ("dup VISA Resource Name"=w598:refnum<visa-resource-name>, "Device Found?"=w579:bool, "Detected MICS IDs"=w585:u32[], "error out"=w582:errorcluster)  [unwired: 6 in]
          n266 = local read "SESSION CONTROL"() -> (w597:T3)
          n267 = for {
            tunnel: w585 -> [w601] mode=indexing
            tunnel: [w599] -> w590 mode=indexing
            n268 = Number To Hexadecimal String(1:i16 6 ("width (-)"), 2:w601) -> (0:w599:string)
          }
          n269 = Index Array(array=w585) -> (element=w591:u32)  [unwired: 1 in]
          n270 = local write "Device Found?"(w579) -> ()
          n271 = Bundle By Name(cluster=w597, "TARGET MICS ID"=w591) -> (w596:T3)
          n272 = global write "MICS_ID Global.vi" "MICS_ID"(w591) -> ()
          n273 = property on="Detected MICS IDs" class="LstBox (strict)"("Item Names"=w590) -> ()  [unwired: 2 in, 2 out]
          n274 = local write "SESSION CONTROL"(w596) -> ()
          n275 = local read "Search for Device"() -> (w580:bool)
          n276 = Unbundle By Name(w582) -> ("status"=w581:bool)
          n277 = Select(t=T25."Continue Search" ("Mode"), s=w580, f=w587) -> (s? t:f=w588:T25)
          n278 = Equal?(x=w587, y=w586) -> (x = y?=w584:bool)
          n279 = Or(x=w584, y=w581) -> (x .or. y?=w583:bool)
        }
      }
      frame "Uplink Patient Program" {
        n280 = Number To Decimal String(number="LoadPatProgSlot") -> (decimal integer string=w620:string)  [unwired: 1 in]
        n281 = Concatenate Strings("program=", w620) -> (w618:string)
        n282 = call "MICSD Telem Driver.vi"("VISA Resource Name"=w615, "Command"=Typedef_Command_List."Get Program Definition", "Parameters"=w618, "error in (no error)"=w623) -> ("Response Token"=w612:string, "Response Code"=w611:string, "Data"=w617:string, "error out"=w624:errorcluster)  [unwired: 9 in, 3 out]
        n283 = local read "PatStim"() -> (w616:T10)
        n284 = Concatenate Strings(w612, " - ", w611) -> (w613:string)
        n285 = local write "Response"(w613) -> ()
        n286 = Match Pattern(string=w611, regular expression="COMMAND ACCEPTED" ("Response Code")) -> (offset past match=w609:i32)  [unwired: 1 in, 3 out]
        n287 = Greater Than 0?(x=w609) -> (x > 0?=w608:bool)
        n288 = case shown="True" w608 {
          tunnel: w617 -> [_ w629]
          tunnel: w616 -> [_ w630]
          frame False {
            n289 = One Button Dialog(message="\"Get Program Definition\" telemetry command failed!") -> ()  [unwired: 1 in, 1 out]
          }
          frame True {
            n290 = for {
              N: 11 -> [_]
              shift-right: [w632] -> w631
              shift-left: w630 -> [w634]
              tunnel: w629 -> [w633]
              i -> [w635]
              n291 = case shown="10" w635 {
                tunnel: w634 -> [w641 w659 w697 w734 w767 w800 w833 w847 w862 w877 w892]
                tunnel: w633 -> [w647 w660 w685 w726 w759 w792 w825 w845 w860 w875 w890]
                tunnel: [w640 w658 w696 w733 w766 w799 w832 w846 w861 w876 w891] -> w632
                frame 0, Default {
                  w642 = "YES"
                  w648 = "="
                  n292 = Pick Line(multi-line string=w647, line index=0) -> (output string=w655:string)  [unwired: 1 in]
                  n293 = Pick Line(multi-line string=w647, line index=1) -> (output string=w653:string)  [unwired: 1 in]
                  n294 = Pick Line(multi-line string=w647, line index=2) -> (output string=w651:string)  [unwired: 1 in]
                  n295 = Pick Line(multi-line string=w647, line index=3) -> (output string=w649:string)  [unwired: 1 in]
                  n296 = Match Pattern(string=w655, regular expression=w648) -> (after substring=w646:string)  [unwired: 1 in, 3 out]
                  n297 = Match Pattern(string=w653, regular expression=w648) -> (after substring=w644:string)  [unwired: 1 in, 3 out]
                  n298 = Match Pattern(string=w651, regular expression=w648) -> (after substring=w643:string)  [unwired: 1 in, 3 out]
                  n299 = Match Pattern(string=w649, regular expression=w648) -> (after substring=w639:string)  [unwired: 1 in, 3 out]
                  n300 = Equal?(x=w644, y=w642) -> (x = y?=w637:bool)
                  n301 = Equal?(x=w643, y=w642) -> (x = y?=w638:bool)
                  n302 = Decimal String To Number(string=w646, default (0L)=u8 0 ("line index")) -> (number=w636:u8)  [unwired: 1 in, 1 out]
                  n303 = Bundle By Name(cluster=w641, "Program Number"=w636, "Program Defined"=w637, "Program Disabled"=w638, "Program Name"=w639) -> (w640:T10)
                }
                frame 1 {
                  n304 = for {
                    N: 8 -> [w665]
                    tunnel: w660 -> [w668]
                    tunnel: [w666] -> w657 mode=indexing
                    i -> [w669]
                    n305 = Multiply(x=w665, y=w669) -> (x*y=w664:i32)
                    n306 = Add(x=w664, y=4) -> (x+y=w662:i32)
                    n307 = for {
                      N: w665 -> [_]
                      tunnel: w662 -> [w671]
                      tunnel: w668 -> [w680]
                      shift-right: [w675] -> w666
                      shift-left: u8 0 ("y") -> [w676]
                      i -> [w670]
                      n308 = Add(x=w670, y=w671) -> (x+y=w672:i32)
                      n309 = Pick Line(multi-line string=w680, line index=w672) -> (output string=w683:string)  [unwired: 1 in]
                      n310 = Match Pattern(string=w683, regular expression="=") -> (after substring=w682:string)  [unwired: 1 in, 3 out]
                      n311 = Equal?(x=w682, y="YES") -> (x = y?=w678:bool)
                      n312 = Boolean To (0,1)(Boolean=w678) -> (0, 1=w677:i16)
                      n313 = Logical Shift(y=w670, x=w677) -> (x << y=w674:i16)
                      n314 = To Unsigned Byte Integer(number=w674) -> (unsigned 8bit integer=w673:u8)
                      n315 = Add(x=w676, y=w673) -> (x+y=w675:u8)
                    }
                  }
                  n316 = Bundle By Name(cluster=w659, "Allowed Freq Indexes"=w657) -> (w658:T10)
                }
                frame 2 {
                  w686 = "YES"
                  w687 = "="
                  n317 = Pick Line(multi-line string=w685, line index=68) -> (output string=w708:string)  [unwired: 1 in]
                  n318 = Pick Line(multi-line string=w685, line index=69) -> (output string=w706:string)  [unwired: 1 in]
                  n319 = Pick Line(multi-line string=w685, line index=70) -> (output string=w704:string)  [unwired: 1 in]
                  n320 = Pick Line(multi-line string=w685, line index=71) -> (output string=w702:string)  [unwired: 1 in]
                  n321 = Pick Line(multi-line string=w685, line index=72) -> (output string=w689:string)  [unwired: 1 in]
                  n322 = Match Pattern(string=w708, regular expression=w687) -> (after substring=w701:string)  [unwired: 1 in, 3 out]
                  n323 = Match Pattern(string=w706, regular expression=w687) -> (after substring=w699:string)  [unwired: 1 in, 3 out]
                  n324 = Match Pattern(string=w704, regular expression=w687) -> (after substring=w698:string)  [unwired: 1 in, 3 out]
                  n325 = Match Pattern(string=w702, regular expression=w687) -> (after substring=w692:string)  [unwired: 1 in, 3 out]
                  n326 = Match Pattern(string=w689, regular expression=w687) -> (after substring=w688:string)  [unwired: 1 in, 3 out]
                  n327 = Equal?(x=w699, y=w686) -> (x = y?=w694:bool)
                  n328 = Equal?(x=w698, y=w686) -> (x = y?=w695:bool)
                  n329 = Equal?(x=w692, y=w686) -> (x = y?=w691:bool)
                  n330 = Equal?(x=w688, y=w686) -> (x = y?=w684:bool)
                  n331 = Decimal String To Number(string=w701, default (0L)=u8 0 ("line index")) -> (number=w693:u8)  [unwired: 1 in, 1 out]
                  n332 = Bundle By Name(cluster=w697, "Default Freq Index"=w693, "PA.Defined"=w694, "PB.Defined"=w695, "PC.Defined"=w691, "PD.Defined"=w684) -> (w696:T10)
                }
                frame 3 {
                  w717 = u16 0  # U16
                  w716 = u8 0  # U8
                  w725 = "="
                  n333 = Pick Line(multi-line string=w726, line index=75) -> (output string=w741:string)  [unwired: 1 in]
                  n334 = Pick Line(multi-line string=w726, line index=76) -> (output string=w739:string)  [unwired: 1 in]
                  n335 = Pick Line(multi-line string=w726, line index=77) -> (output string=w737:string)  [unwired: 1 in]
                  n336 = Pick Line(multi-line string=w726, line index=78) -> (output string=w735:string)  [unwired: 1 in]
                  n337 = Pick Line(multi-line string=w726, line index=79) -> (output string=w731:string)  [unwired: 1 in]
                  n338 = Pick Line(multi-line string=w726, line index=80) -> (output string=w729:string)  [unwired: 1 in]
                  n339 = Pick Line(multi-line string=w726, line index=81) -> (output string=w727:string)  [unwired: 1 in]
                  n340 = Match Pattern(string=w741, regular expression=w725) -> (after substring=w718:string)  [unwired: 1 in, 3 out]
                  n341 = Match Pattern(string=w739, regular expression=w725) -> (after substring=w724:string)  [unwired: 1 in, 3 out]
                  n342 = Match Pattern(string=w737, regular expression=w725) -> (after substring=w719:string)  [unwired: 1 in, 3 out]
                  n343 = Match Pattern(string=w735, regular expression=w725) -> (after substring=w720:string)  [unwired: 1 in, 3 out]
                  n344 = Match Pattern(string=w731, regular expression=w725) -> (after substring=w721:string)  [unwired: 1 in, 3 out]
                  n345 = Match Pattern(string=w729, regular expression=w725) -> (after substring=w722:string)  [unwired: 1 in, 3 out]
                  n346 = Match Pattern(string=w727, regular expression=w725) -> (after substring=w723:string)  [unwired: 1 in, 3 out]
                  n347 = Decimal String To Number(string=w724, default (0L)=w717) -> (number=w715:u16)  [unwired: 1 in, 1 out]
                  n348 = Decimal String To Number(string=w719, default (0L)=w717) -> (number=w714:u16)  [unwired: 1 in, 1 out]
                  n349 = Decimal String To Number(string=w720, default (0L)=w716) -> (number=w713:u8)  [unwired: 1 in, 1 out]
                  n350 = Decimal String To Number(string=w721, default (0L)=w717) -> (number=w712:u16)  [unwired: 1 in, 1 out]
                  n351 = Decimal String To Number(string=w722, default (0L)=w717) -> (number=w711:u16)  [unwired: 1 in, 1 out]
                  n352 = Decimal String To Number(string=w723, default (0L)=w717) -> (number=w710:u16)  [unwired: 1 in, 1 out]
                  n353 = Bundle By Name(cluster=w734, "PA.Pulse Name"=w718, "PA.Amp Low Limit (uA)"=w715, "PA.Amp Step (uA)"=w714, "PA.Amp Step Index"=w713, "PA.PW Low Limit (uS)"=w712, "PA.PW High Limit (uS)"=w711, "PA.PW Default (uS)"=w710) -> (w733:T10)
                }
                frame 4 {
                  w750 = u16 0  # U16
                  w749 = u8 0  # U8
                  w758 = "="
                  n354 = Pick Line(multi-line string=w759, line index=110) -> (output string=w774:string)  [unwired: 1 in]
                  n355 = Pick Line(multi-line string=w759, line index=111) -> (output string=w772:string)  [unwired: 1 in]
                  n356 = Pick Line(multi-line string=w759, line index=112) -> (output string=w770:string)  [unwired: 1 in]
                  n357 = Pick Line(multi-line string=w759, line index=113) -> (output string=w768:string)  [unwired: 1 in]
                  n358 = Pick Line(multi-line string=w759, line index=114) -> (output string=w764:string)  [unwired: 1 in]
                  n359 = Pick Line(multi-line string=w759, line index=115) -> (output string=w762:string)  [unwired: 1 in]
                  n360 = Pick Line(multi-line string=w759, line index=116) -> (output string=w760:string)  [unwired: 1 in]
                  n361 = Match Pattern(string=w774, regular expression=w758) -> (after substring=w751:string)  [unwired: 1 in, 3 out]
                  n362 = Match Pattern(string=w772, regular expression=w758) -> (after substring=w757:string)  [unwired: 1 in, 3 out]
                  n363 = Match Pattern(string=w770, regular expression=w758) -> (after substring=w752:string)  [unwired: 1 in, 3 out]
                  n364 = Match Pattern(string=w768, regular expression=w758) -> (after substring=w753:string)  [unwired: 1 in, 3 out]
                  n365 = Match Pattern(string=w764, regular expression=w758) -> (after substring=w754:string)  [unwired: 1 in, 3 out]
                  n366 = Match Pattern(string=w762, regular expression=w758) -> (after substring=w755:string)  [unwired: 1 in, 3 out]
                  n367 = Match Pattern(string=w760, regular expression=w758) -> (after substring=w756:string)  [unwired: 1 in, 3 out]
                  n368 = Decimal String To Number(string=w757, default (0L)=w750) -> (number=w748:u16)  [unwired: 1 in, 1 out]
                  n369 = Decimal String To Number(string=w752, default (0L)=w750) -> (number=w747:u16)  [unwired: 1 in, 1 out]
                  n370 = Decimal String To Number(string=w753, default (0L)=w749) -> (number=w746:u8)  [unwired: 1 in, 1 out]
                  n371 = Decimal String To Number(string=w754, default (0L)=w750) -> (number=w745:u16)  [unwired: 1 in, 1 out]
                  n372 = Decimal String To Number(string=w755, default (0L)=w750) -> (number=w744:u16)  [unwired: 1 in, 1 out]
                  n373 = Decimal String To Number(string=w756, default (0L)=w750) -> (number=w743:u16)  [unwired: 1 in, 1 out]
                  n374 = Bundle By Name(cluster=w767, "PB.Pulse Name"=w751, "PB.Amp Low Limit (uA)"=w748, "PB.Amp Step (uA)"=w747, "PB.Amp Step Index"=w746, "PB.PW Low Limit (uS)"=w745, "PB.PW High Limit (uS)"=w744, "PB.PW Default (uS)"=w743) -> (w766:T10)
                }
                frame 5 {
                  w783 = u16 0  # U16
                  w782 = u8 0  # U8
                  w791 = "="
                  n375 = Pick Line(multi-line string=w792, line index=145) -> (output string=w807:string)  [unwired: 1 in]
                  n376 = Pick Line(multi-line string=w792, line index=146) -> (output string=w805:string)  [unwired: 1 in]
                  n377 = Pick Line(multi-line string=w792, line index=147) -> (output string=w803:string)  [unwired: 1 in]
                  n378 = Pick Line(multi-line string=w792, line index=148) -> (output string=w801:string)  [unwired: 1 in]
                  n379 = Pick Line(multi-line string=w792, line index=149) -> (output string=w797:string)  [unwired: 1 in]
                  n380 = Pick Line(multi-line string=w792, line index=150) -> (output string=w795:string)  [unwired: 1 in]
                  n381 = Pick Line(multi-line string=w792, line index=151) -> (output string=w793:string)  [unwired: 1 in]
                  n382 = Match Pattern(string=w807, regular expression=w791) -> (after substring=w784:string)  [unwired: 1 in, 3 out]
                  n383 = Match Pattern(string=w805, regular expression=w791) -> (after substring=w790:string)  [unwired: 1 in, 3 out]
                  n384 = Match Pattern(string=w803, regular expression=w791) -> (after substring=w785:string)  [unwired: 1 in, 3 out]
                  n385 = Match Pattern(string=w801, regular expression=w791) -> (after substring=w786:string)  [unwired: 1 in, 3 out]
                  n386 = Match Pattern(string=w797, regular expression=w791) -> (after substring=w787:string)  [unwired: 1 in, 3 out]
                  n387 = Match Pattern(string=w795, regular expression=w791) -> (after substring=w788:string)  [unwired: 1 in, 3 out]
                  n388 = Match Pattern(string=w793, regular expression=w791) -> (after substring=w789:string)  [unwired: 1 in, 3 out]
                  n389 = Decimal String To Number(string=w790, default (0L)=w783) -> (number=w781:u16)  [unwired: 1 in, 1 out]
                  n390 = Decimal String To Number(string=w785, default (0L)=w783) -> (number=w780:u16)  [unwired: 1 in, 1 out]
                  n391 = Decimal String To Number(string=w786, default (0L)=w782) -> (number=w779:u8)  [unwired: 1 in, 1 out]
                  n392 = Decimal String To Number(string=w787, default (0L)=w783) -> (number=w778:u16)  [unwired: 1 in, 1 out]
                  n393 = Decimal String To Number(string=w788, default (0L)=w783) -> (number=w777:u16)  [unwired: 1 in, 1 out]
                  n394 = Decimal String To Number(string=w789, default (0L)=w783) -> (number=w776:u16)  [unwired: 1 in, 1 out]
                  n395 = Bundle By Name(cluster=w800, "PC.Pulse Name"=w784, "PC.Amp Low Limit (uA)"=w781, "PC.Amp Step (uA)"=w780, "PC.Amp Step Index"=w779, "PC.PW Low Limit (uS)"=w778, "PC.PW High Limit (uS)"=w777, "PC.PW Default (uS)"=w776) -> (w799:T10)
                }
                frame 6 {
                  w816 = u16 0  # U16
                  w815 = u8 0  # U8
                  w824 = "="
                  n396 = Pick Line(multi-line string=w825, line index=180) -> (output string=w840:string)  [unwired: 1 in]
                  n397 = Pick Line(multi-line string=w825, line index=181) -> (output string=w838:string)  [unwired: 1 in]
                  n398 = Pick Line(multi-line string=w825, line index=182) -> (output string=w836:string)  [unwired: 1 in]
                  n399 = Pick Line(multi-line string=w825, line index=183) -> (output string=w834:string)  [unwired: 1 in]
                  n400 = Pick Line(multi-line string=w825, line index=184) -> (output string=w830:string)  [unwired: 1 in]
                  n401 = Pick Line(multi-line string=w825, line index=185) -> (output string=w828:string)  [unwired: 1 in]
                  n402 = Pick Line(multi-line string=w825, line index=186) -> (output string=w826:string)  [unwired: 1 in]
                  n403 = Match Pattern(string=w840, regular expression=w824) -> (after substring=w817:string)  [unwired: 1 in, 3 out]
                  n404 = Match Pattern(string=w838, regular expression=w824) -> (after substring=w823:string)  [unwired: 1 in, 3 out]
                  n405 = Match Pattern(string=w836, regular expression=w824) -> (after substring=w818:string)  [unwired: 1 in, 3 out]
                  n406 = Match Pattern(string=w834, regular expression=w824) -> (after substring=w819:string)  [unwired: 1 in, 3 out]
                  n407 = Match Pattern(string=w830, regular expression=w824) -> (after substring=w820:string)  [unwired: 1 in, 3 out]
                  n408 = Match Pattern(string=w828, regular expression=w824) -> (after substring=w821:string)  [unwired: 1 in, 3 out]
                  n409 = Match Pattern(string=w826, regular expression=w824) -> (after substring=w822:string)  [unwired: 1 in, 3 out]
                  n410 = Decimal String To Number(string=w823, default (0L)=w816) -> (number=w814:u16)  [unwired: 1 in, 1 out]
                  n411 = Decimal String To Number(string=w818, default (0L)=w816) -> (number=w813:u16)  [unwired: 1 in, 1 out]
                  n412 = Decimal String To Number(string=w819, default (0L)=w815) -> (number=w812:u8)  [unwired: 1 in, 1 out]
                  n413 = Decimal String To Number(string=w820, default (0L)=w816) -> (number=w811:u16)  [unwired: 1 in, 1 out]
                  n414 = Decimal String To Number(string=w821, default (0L)=w816) -> (number=w810:u16)  [unwired: 1 in, 1 out]
                  n415 = Decimal String To Number(string=w822, default (0L)=w816) -> (number=w809:u16)  [unwired: 1 in, 1 out]
                  n416 = Bundle By Name(cluster=w833, "PD.Pulse Name"=w817, "PD.Amp Low Limit (uA)"=w814, "PD.Amp Step (uA)"=w813, "PD.Amp Step Index"=w812, "PD.PW Low Limit (uS)"=w811, "PD.PW High Limit (uS)"=w810, "PD.PW Default (uS)"=w809) -> (w832:T10)
                }
                frame 7 {
                  n417 = for {
                    N: 26 -> [_]
                    tunnel: 82 ("line index") -> [w852]
                    tunnel: w845 -> [w854]
                    tunnel: [w848] -> w842 mode=indexing
                    i -> [w851]
                    n418 = Add(x=w851, y=w852) -> (x+y=w853:i32)
                    n419 = Pick Line(multi-line string=w854, line index=w853) -> (output string=w856:string)  [unwired: 1 in]
                    n420 = Match Pattern(string=w856, regular expression="=") -> (after substring=w850:string)  [unwired: 1 in, 3 out]
                    n421 = Decimal String To Number(string=w850, default (0L)=i8 0 ("default (0 I32)")) -> (number=w848:i8)  [unwired: 1 in, 1 out]
                  }
                  n422 = Bundle By Name(cluster=w847, "PA.Amplitudes"=w842) -> (w846:T10)
                }
                frame 8 {
                  n423 = for {
                    N: 26 -> [_]
                    tunnel: 117 ("line index") -> [w867]
                    tunnel: w860 -> [w869]
                    tunnel: [w863] -> w857 mode=indexing
                    i -> [w866]
                    n424 = Add(x=w866, y=w867) -> (x+y=w868:i32)
                    n425 = Pick Line(multi-line string=w869, line index=w868) -> (output string=w871:string)  [unwired: 1 in]
                    n426 = Match Pattern(string=w871, regular expression="=") -> (after substring=w865:string)  [unwired: 1 in, 3 out]
                    n427 = Decimal String To Number(string=w865, default (0L)=i8 0 ("default (0 I32)")) -> (number=w863:i8)  [unwired: 1 in, 1 out]
                  }
                  n428 = Bundle By Name(cluster=w862, "PB.Amplitudes"=w857) -> (w861:T10)
                }
                frame 9 {
                  n429 = for {
                    N: 26 -> [_]
                    tunnel: 152 ("line index") -> [w882]
                    tunnel: w875 -> [w884]
                    tunnel: [w878] -> w872 mode=indexing
                    i -> [w881]
                    n430 = Add(x=w881, y=w882) -> (x+y=w883:i32)
                    n431 = Pick Line(multi-line string=w884, line index=w883) -> (output string=w886:string)  [unwired: 1 in]
                    n432 = Match Pattern(string=w886, regular expression="=") -> (after substring=w880:string)  [unwired: 1 in, 3 out]
                    n433 = Decimal String To Number(string=w880, default (0L)=i8 0 ("default (0 I32)")) -> (number=w878:i8)  [unwired: 1 in, 1 out]
                  }
                  n434 = Bundle By Name(cluster=w877, "PC.Amplitudes"=w872) -> (w876:T10)
                }
                frame 10 {
                  n435 = for {
                    N: 26 -> [_]
                    tunnel: 187 ("line index") -> [w897]
                    tunnel: w890 -> [w899]
                    tunnel: [w893] -> w887 mode=indexing
                    i -> [w896]
                    n436 = Add(x=w896, y=w897) -> (x+y=w898:i32)
                    n437 = Pick Line(multi-line string=w899, line index=w898) -> (output string=w901:string)  [unwired: 1 in]
                    n438 = Match Pattern(string=w901, regular expression="=") -> (after substring=w895:string)  [unwired: 1 in, 3 out]
                    n439 = Decimal String To Number(string=w895, default (0L)=i8 0 ("default (0 I32)")) -> (number=w893:i8)  [unwired: 1 in, 1 out]
                  }
                  n440 = Bundle By Name(cluster=w892, "PD.Amplitudes"=w887) -> (w891:T10)
                }
              }
            }
            n441 = local write "PatStim"(w631) -> ()
          }
        }
      }
      frame "Top of Loop" {
        # "Force status update every 3s\nif \"Get VBAT Cont\" is active, \nelse every 0.5s"
        n442 = local read "Get VBAT Cont"() -> (w909:bool)
        n443 = Tick Count (ms)() -> (millisecond timer value=w906:u32)
        n444 = Select(t=w905, s=w909, f=u32 500 ("y")) -> (s? t:f=w907:u32)
        n445 = Add(x="Tick Count", y=w907) -> (x+y=w916:u32)
        n446 = property on="Tab Control" class="TabCtl (strict)"("DisabledEnum"=T23."Enabled" ("Disabled")) -> ()  [unwired: 2 in, 2 out]
        n447 = Greater?(x=w906, y=w916) -> (0:w915:bool)
        n448 = Select(t=string[] ["Get Status"], s=w915, f=w919) -> (s? t:f=w920:string[])
        n449 = for {
          N: 55 -> [_]
          shift-right: [w926] -> w913
          shift-left: w920 -> [w927]
          tunnel: w906 -> [w925]
          i -> [w928]
          n450 = case shown="36" w928 {
            tunnel: w927 -> [w932 w942 w949 w957 w965 w973 w981 w989 w997 w1005 w1013 w1021 w1029 w1037 w1045 w1053 w1061 w1073 w1094 w1102 w1110 w1118 w1126 w1134 w1142 w1150 w1158 w1166 w1174 w1188 w1204 w1212 w1220 w1228 w1236 w1250 w1264 w1272 w1280 w1288 w1296 w1304 w1312 w1323 w1331 w1339 w1346 w1354 w1362 w1370 w1378 w1386 w1394 w1402 w1418]
            tunnel: [w929 w941 w948 w956 w964 w972 w980 w988 w996 w1004 w1012 w1020 w1028 w1036 w1044 w1052 w1060 w1072 w1093 w1101 w1109 w1117 w1125 w1133 w1141 w1149 w1157 w1165 w1173 w1187 w1203 w1211 w1219 w1227 w1235 w1249 w1263 w1271 w1279 w1287 w1295 w1303 w1311 w1322 w1330 w1338 w1345 w1353 w1361 w1369 w1377 w1385 w1393 w1401 w1417] -> w926
            tunnel: w925 -> [_ _ _ _ _ _ _ _ _ _ _ _ _ _ _ _ _ _ _ _ _ _ _ _ _ _ _ _ _ w1180 _ _ _ _ _ _ _ _ _ _ _ _ _ _ _ _ _ _ _ _ _ _ _ _ _]
            frame 0, Default {
              # "Update CCA"
              n451 = local read "BASE STATION RF CONTROL"() -> (w930:T2)
              n452 = Unbundle By Name(w930) -> ("Update CCA"=w931:bool)
              n453 = case shown="True" w931 {
                tunnel: w932 -> [w933 w936]
                tunnel: w930 -> [_ w938]
                tunnel: [w933 w935] -> w929
                frame False {
                }
                frame True {
                  n454 = Bundle By Name(cluster=w938, "Update CCA"=FALSE ("CCA Mode")) -> (w939:T2)
                  n455 = local write "BASE STATION RF CONTROL"(w939) -> ()
                  n456 = Build Array (concatenate)(w936, string[] ["Get CCA", "Get Status"]) -> (w935:string[])
                }
              }
            }
            frame 1 {
              # "Update CCA"
              n457 = local read "Search for Device"() -> (w940:bool)
              n458 = case shown="True" w940 {
                tunnel: w942 -> [w943 w946]
                tunnel: [w943 w945] -> w941
                frame False {
                }
                frame True {
                  n459 = Build Array (concatenate)(w946, string[] ["Search for Device", "Get Status"]) -> (w945:string[])
                }
              }
            }
            frame 2 {
              # "Update CCA"
              n460 = case shown="True" "Open Session" {
                tunnel: w949 -> [w950 w954]
                tunnel: [w950 w953] -> w948
                frame False {
                }
                frame True {
                  n461 = local write "Open Session"(FALSE ("CCA Mode")) -> ()
                  n462 = Build Array (concatenate)(w954, string[] ["Open Session", "Get Status"]) -> (w953:string[])
                }
              }
            }
            frame 3 {
              # "Update CCA"
              n463 = case shown="True" "Close Session" {
                tunnel: w957 -> [w958 w962]
                tunnel: [w958 w961] -> w956
                frame False {
                }
                frame True {
                  n464 = local write "Close Session"(FALSE ("CCA Mode")) -> ()
                  n465 = Build Array (concatenate)(w962, string[] ["Close Session", "Get Status"]) -> (w961:string[])
                }
              }
            }
            frame 4 {
              # "Update CCA"
              n466 = case shown="True" "Telem Driver" {
                tunnel: w965 -> [w966 w970]
                tunnel: [w966 w969] -> w964
                frame False {
                }
                frame True {
                  n467 = local write "Telem Driver"(FALSE ("CCA Mode")) -> ()
                  n468 = Build Array (concatenate)(w970, string[] ["Telem Driver", "Get Status"]) -> (w969:string[])
                }
              }
            }
            frame 5 {
              # "Update CCA"
              n469 = case shown="False" "LoadPatProgFromDevice" {
                tunnel: w973 -> [w974 w978]
                tunnel: [w974 w977] -> w972
                frame False {
                }
                frame True {
                  n470 = local write "LoadPatProgFromDevice"(FALSE ("CCA Mode")) -> ()
                  n471 = Build Array (concatenate)(w978, string[] ["Uplink Patient Program", "Get Status"]) -> (w977:string[])
                }
              }
            }
            frame 6 {
              # "Update CCA"
              n472 = case shown="False" "Query Error" {
                tunnel: w981 -> [w982 w986]
                tunnel: [w982 w985] -> w980
                frame False {
                }
                frame True {
                  n473 = local write "Query Error"(FALSE ("CCA Mode")) -> ()
                  n474 = Build Array (concatenate)(w986, string[] ["Get BS Error", "Get Status"]) -> (w985:string[])
                }
              }
            }
            frame 7 {
              # "Update CCA"
              n475 = case shown="False" "UpdatePatProgString" {
                tunnel: w989 -> [w990 w994]
                tunnel: [w990 w993] -> w988
                frame False {
                }
                frame True {
                  n476 = local write "UpdatePatProgString"(FALSE ("CCA Mode")) -> ()
                  n477 = Build Array (concatenate)(w994, string[] ["Build Pat Prog String", "Get Status"]) -> (w993:string[])
                }
              }
            }
            frame 8 {
              # "Update CCA"
              n478 = case shown="False" "SendPatProgToDevice" {
                tunnel: w997 -> [w998 w1002]
                tunnel: [w998 w1001] -> w996
                frame False {
                }
                frame True {
                  n479 = local write "SendPatProgToDevice"(FALSE ("CCA Mode")) -> ()
                  n480 = Build Array (concatenate)(w1002, string[] ["Downlink Patient Program", "Get Status"]) -> (w1001:string[])
                }
              }
            }
            frame 9 {
              # "Update CCA"
              n481 = case shown="True" "SetPatProgActive" {
                tunnel: w1005 -> [w1006 w1010]
                tunnel: [w1006 w1009] -> w1004
                frame False {
                }
                frame True {
                  n482 = local write "SetPatProgActive"(FALSE ("CCA Mode")) -> ()
                  n483 = Build Array (concatenate)(w1010, string[] ["Set Program Active", "Get Status"]) -> (w1009:string[])
                }
              }
            }
            frame 10 {
              # "Update CCA"
              n484 = case shown="True" "StartStimulation" {
                tunnel: w1013 -> [w1014 w1018]
                tunnel: [w1014 w1017] -> w1012
                frame False {
                }
                frame True {
                  n485 = local write "StartStimulation"(FALSE ("CCA Mode")) -> ()
                  n486 = Build Array (concatenate)(w1018, string[] ["Start Patient Stim", "Get Status"]) -> (w1017:string[])
                }
              }
            }
            frame 11 {
              # "Update CCA"
              n487 = case shown="True" "StopStimulation" {
                tunnel: w1021 -> [w1022 w1026]
                tunnel: [w1022 w1025] -> w1020
                frame False {
                }
                frame True {
                  n488 = local write "StopStimulation"(FALSE ("CCA Mode")) -> ()
                  n489 = Build Array (concatenate)(w1026, string[] ["Stop Stimulation", "Get Status"]) -> (w1025:string[])
                }
              }
            }
            frame 12 {
              # "Update CCA"
              n490 = case shown="True" "ProgAmpUp" {
                tunnel: w1029 -> [w1030 w1034]
                tunnel: [w1030 w1033] -> w1028
                frame False {
                }
                frame True {
                  n491 = local write "ProgAmpUp"(FALSE ("CCA Mode")) -> ()
                  n492 = Build Array (concatenate)(w1034, string[] ["Increment Program Ampl", "Get Status"]) -> (w1033:string[])
                }
              }
            }
            frame 13 {
              # "Update CCA"
              n493 = case shown="True" "ProgAmpDn" {
                tunnel: w1037 -> [w1038 w1042]
                tunnel: [w1038 w1041] -> w1036
                frame False {
                }
                frame True {
                  n494 = local write "ProgAmpDn"(FALSE ("CCA Mode")) -> ()
                  n495 = Build Array (concatenate)(w1042, string[] ["Decrement Program Ampl", "Get Status"]) -> (w1041:string[])
                }
              }
            }
            frame 14 {
              # "Update CCA"
              n496 = case shown="True" "FreqUp" {
                tunnel: w1045 -> [w1046 w1050]
                tunnel: [w1046 w1049] -> w1044
                frame False {
                }
                frame True {
                  n497 = local write "FreqUp"(FALSE ("CCA Mode")) -> ()
                  n498 = Build Array (concatenate)(w1050, string[] ["Increment Program Freq", "Get Status"]) -> (w1049:string[])
                }
              }
            }
            frame 15 {
              # "Update CCA"
              n499 = case shown="True" "FreqDn" {
                tunnel: w1053 -> [w1054 w1058]
                tunnel: [w1054 w1057] -> w1052
                frame False {
                }
                frame True {
                  n500 = local write "FreqDn"(FALSE ("CCA Mode")) -> ()
                  n501 = Build Array (concatenate)(w1058, string[] ["Decrement Program Freq", "Get Status"]) -> (w1057:string[])
                }
              }
            }
            frame 16 {
              # "Update CCA"
              n502 = case shown="True" "Get Attenuator" {
                tunnel: w1061 -> [w1062 w1066]
                tunnel: [w1062 w1065] -> w1060
                frame False {
                }
                frame True {
                  n503 = local write "Get Attenuator"(FALSE ("CCA Mode")) -> ()
                  n504 = Build Array (concatenate)(w1066, string[] ["Get Attenuator", "Get Status"]) -> (w1065:string[])
                }
              }
            }
            frame 17 {
              # "Update CCA"
              n505 = Compound Arithmetic op=OR("Set Attenuator", "Atten +1 dB", "Atten -1 dB", "AttenZero") -> (w1067:bool)
              n506 = case shown="True" w1067 {
                tunnel: w1073 -> [w1074 w1086]
                tunnel: [w1074 w1085] -> w1072
                tunnel: "Set Attenuator" -> [_ w1079]
                tunnel: "Atten +1 dB" -> [_ w1080]
                tunnel: "Atten -1 dB" -> [_ w1081]
                tunnel: "AttenZero" -> [_ w1082]
                frame False {
                }
                frame True {
                  w1083 = FALSE ("CCA Mode")
                  n507 = Build Array(w1079, w1080, w1081, w1082) -> (w1078:bool[])
                  n508 = Boolean Array To Number(Boolean array=w1078) -> (number=w1077:u32)
                  n509 = case shown="1" w1077 {
                    tunnel: enum16{"Null", "Increment", "Decrement", "Zero"}."Null" ("AttenMode") -> [w1087 w1088 _ _ _]
                    tunnel: [w1087 w1088 enum16{"Null", "Increment", "Decrement", "Zero"}."Increment" ("AttenMode") enum16{"Null", "Increment", "Decrement", "Zero"}."Decrement" ("AttenMode") enum16{"Null", "Increment", "Decrement", "Zero"}."Zero" ("AttenMode")] -> w1075
                    frame 0, Default {
                    }
                    frame 1 {
                    }
                    frame 2 {
                    }
                    frame 4 {
                    }
                    frame 8 {
                    }
                  }
                  n510 = local write "AttenMode"(w1075) -> ()
                  n511 = local write "Atten -1 dB"(w1083) -> ()
                  n512 = local write "Set Attenuator"(w1083) -> ()
                  n513 = local write "Atten +1 dB"(w1083) -> ()
                  n514 = local write "AttenZero"(w1083) -> ()
                  n515 = Build Array (concatenate)(w1086, string[] ["Set Attenuator", "Get Status"]) -> (w1085:string[])
                }
              }
            }
            frame 18 {
              # "Update CCA"
              n516 = case shown="True" "Do Calibration" {
                tunnel: w1094 -> [w1095 w1099]
                tunnel: [w1095 w1098] -> w1093
                frame False {
                }
                frame True {
                  n517 = local write "Do Calibration"(FALSE ("CCA Mode")) -> ()
                  n518 = Build Array (concatenate)(w1099, string[] ["Run Calibration", "Get Status"]) -> (w1098:string[])
                }
              }
            }
            frame 19 {
              # "Update CCA"
              n519 = case shown="True" "Get Register" {
                tunnel: w1102 -> [w1103 w1107]
                tunnel: [w1103 w1106] -> w1101
                frame False {
                }
                frame True {
                  n520 = local write "Get Register"(FALSE ("CCA Mode")) -> ()
                  n521 = Build Array (concatenate)(w1107, string[] ["Get Register", "Get Status"]) -> (w1106:string[])
                }
              }
            }
            frame 20 {
              # "Update CCA"
              n522 = case shown="True" "Set Register" {
                tunnel: w1110 -> [w1111 w1115]
                tunnel: [w1111 w1114] -> w1109
                frame False {
                }
                frame True {
                  n523 = local write "Set Register"(FALSE ("CCA Mode")) -> ()
                  n524 = Build Array (concatenate)(w1115, string[] ["Set Register", "Get Status"]) -> (w1114:string[])
                }
              }
            }
            frame 21 {
              # "Update CCA"
              n525 = case shown="True" "LoadPatProgFromFile" {
                tunnel: w1118 -> [w1119 w1123]
                tunnel: [w1119 w1122] -> w1117
                frame False {
                }
                frame True {
                  n526 = local write "LoadPatProgFromFile"(FALSE ("CCA Mode")) -> ()
                  n527 = Build Array (concatenate)(w1123, string[] ["Load Pat Program", "Get Status"]) -> (w1122:string[])
                }
              }
            }
            frame 22 {
              # "Update CCA"
              n528 = case shown="True" "SavePatProgToFile" {
                tunnel: w1126 -> [w1127 w1131]
                tunnel: [w1127 w1130] -> w1125
                frame False {
                }
                frame True {
                  n529 = local write "SavePatProgToFile"(FALSE ("CCA Mode")) -> ()
                  n530 = Build Array (concatenate)(w1131, string[] ["Save Pat Program", "Get Status"]) -> (w1130:string[])
                }
              }
            }
            frame 23 {
              # "Update CCA"
              n531 = case shown="True" "Dongle Reset" {
                tunnel: w1134 -> [w1135 w1139]
                tunnel: [w1135 w1138] -> w1133
                frame False {
                }
                frame True {
                  n532 = local write "Dongle Reset"(FALSE ("CCA Mode")) -> ()
                  n533 = Build Array (concatenate)(w1139, string[] ["Reset Dongle", "Get Status"]) -> (w1138:string[])
                }
              }
            }
            frame 24 {
              # "Update CCA"
              n534 = case shown="True" "ZL Mass Read" {
                tunnel: w1142 -> [w1143 w1147]
                tunnel: [w1143 w1146] -> w1141
                frame False {
                }
                frame True {
                  n535 = local write "ZL Mass Read"(FALSE ("CCA Mode")) -> ()
                  n536 = Build Array (concatenate)(w1147, string[] ["ZL Register Mass Read", "Get Status"]) -> (w1146:string[])
                }
              }
            }
            frame 25 {
              # "Update CCA"
              n537 = case shown="True" "Set CW" {
                tunnel: w1150 -> [w1151 w1155]
                tunnel: [w1151 w1154] -> w1149
                frame False {
                }
                frame True {
                  n538 = local write "Set CW"(FALSE ("CCA Mode")) -> ()
                  n539 = Build Array (concatenate)(w1155, string[] ["Set CW Mode", "Get Status"]) -> (w1154:string[])
                }
              }
            }
            frame 26 {
              # "Update CCA"
              n540 = case shown="True" "Set Base Pwr" {
                tunnel: w1158 -> [w1159 w1163]
                tunnel: [w1159 w1162] -> w1157
                frame False {
                }
                frame True {
                  n541 = local write "Set Base Pwr"(FALSE ("CCA Mode")) -> ()
                  n542 = Build Array (concatenate)(w1163, string[] ["Set RF Power - Base", "Get Status"]) -> (w1162:string[])
                }
              }
            }
            frame 27 {
              # "Update CCA"
              n543 = case shown="True" "Set Remote Pwr" {
                tunnel: w1166 -> [w1167 w1171]
                tunnel: [w1167 w1170] -> w1165
                frame False {
                }
                frame True {
                  n544 = local write "Set Remote Pwr"(FALSE ("CCA Mode")) -> ()
                  n545 = Build Array (concatenate)(w1171, string[] ["Set RF Power - Remote", "Get Status"]) -> (w1170:string[])
                }
              }
            }
            frame 28 {
              # "Update CCA"
              n546 = case shown="True" "Load Template" {
                tunnel: w1174 -> [w1175 w1179]
                tunnel: [w1175 w1178] -> w1173
                frame False {
                }
                frame True {
                  n547 = local write "Load Template"(FALSE ("CCA Mode")) -> ()
                  n548 = Build Array (concatenate)(w1179, string[] ["Load Cmd Template", "Get Status"]) -> (w1178:string[])
                }
              }
            }
            frame 29 {
              # "Service Discharge Function"
              n549 = local read "Discharge"() -> (w1185:T9)
              n550 = Add(x=u32 5000 ("y"), y="Discharge Delay") -> (x+y=w1184:u32)
              n551 = Greater?(x=w1180, y=w1184) -> (0:w1181:bool)
              n552 = case shown="True" w1181 {
                tunnel: [FALSE w1191] -> w1186
                tunnel: w1185 -> [_ w1190]
                tunnel: w1180 -> [_ _]
                frame False {
                }
                frame True {
                  n553 = for {
                    shift-right: [w1195] -> w1191
                    shift-left: FALSE -> [w1194]
                    tunnel: w1190 -> [w1196] mode=indexing
                    n554 = Unbundle By Name(w1196) -> ("Activate"=w1193:bool)
                    n555 = Or(x=w1193, y=w1194) -> (x .or. y?=w1195:bool)
                  }
                }
              }
              n556 = case shown="True" w1186 {
                tunnel: w1188 -> [w1197 w1201]
                tunnel: [w1197 w1200] -> w1187
                frame False {
                }
                frame True {
                  n557 = Build Array (concatenate)(w1201, string[] ["Discharge Control"]) -> (w1200:string[])
                  "Active" <- -1
                }
              }
            }
            frame 30 {
              # "Update CCA"
              n558 = case shown="True" "PulsePWUp" {
                tunnel: w1204 -> [w1205 w1209]
                tunnel: [w1205 w1208] -> w1203
                frame False {
                }
                frame True {
                  n559 = local write "PulsePWUp"(FALSE ("CCA Mode")) -> ()
                  n560 = Build Array (concatenate)(w1209, string[] ["PulseWidthUp", "Get Status"]) -> (w1208:string[])
                }
              }
            }
            frame 31 {
              # "Update CCA"
              n561 = case shown="True" "PulsePWDn" {
                tunnel: w1212 -> [w1213 w1217]
                tunnel: [w1213 w1216] -> w1211
                frame False {
                }
                frame True {
                  n562 = local write "PulsePWDn"(FALSE ("CCA Mode")) -> ()
                  n563 = Build Array (concatenate)(w1217, string[] ["PulseWidthDown", "Get Status"]) -> (w1216:string[])
                }
              }
            }
            frame 32 {
              # "Update CCA"
              n564 = case shown="True" "PulseAmpUp" {
                tunnel: w1220 -> [w1221 w1225]
                tunnel: [w1221 w1224] -> w1219
                frame False {
                }
                frame True {
                  n565 = local write "PulseAmpUp"(FALSE ("CCA Mode")) -> ()
                  n566 = Build Array (concatenate)(w1225, string[] ["PulseAmplUp", "Get Status"]) -> (w1224:string[])
                }
              }
            }
            frame 33 {
              # "Update CCA"
              n567 = case shown="True" "PulseAmpDn" {
                tunnel: w1228 -> [w1229 w1233]
                tunnel: [w1229 w1232] -> w1227
                frame False {
                }
                frame True {
                  n568 = local write "PulseAmpDn"(FALSE ("CCA Mode")) -> ()
                  n569 = Build Array (concatenate)(w1233, string[] ["PulseAmplDown", "Get Status"]) -> (w1232:string[])
                }
              }
            }
            frame 34 {
              # "Update CCA"
              n570 = case shown="True" "Set_INFO_D" {
                tunnel: w1236 -> [w1237 w1243]
                tunnel: [w1237 w1242] -> w1235
                frame False {
                }
                frame True {
                  n571 = Two Button Dialog(message="You are about to overwrite the stored INFO_D Calibration Data!!  Do you wish to proceed?", 2:"Overwrite" ("T button name (\"OK\")")) -> (T button?=w1238:bool)  [unwired: 1 in]
                  n572 = case shown="True" w1238 {
                    tunnel: w1243 -> [w1244 w1247]
                    tunnel: [w1244 w1246] -> w1242
                    frame False {
                    }
                    frame True {
                      n573 = Build Array (concatenate)(w1247, string[] ["Set Calibration INFO_D", "Reset Dongle", "Get Status"]) -> (w1246:string[])
                    }
                  }
                  n574 = local write "Set_INFO_D"(FALSE ("CCA Mode")) -> ()
                }
              }
            }
            frame 35 {
              # "Update CCA"
              n575 = case shown="True" "Set_INFO_C" {
                tunnel: w1250 -> [w1251 w1257]
                tunnel: [w1251 w1256] -> w1249
                frame False {
                }
                frame True {
                  n576 = Two Button Dialog(message="You are about to overwrite the stored INFO_C Calibration Data!!  Do you wish to proceed?", 2:"Overwrite" ("T button name (\"OK\")")) -> (T button?=w1252:bool)  [unwired: 1 in]
                  n577 = case shown="True" w1252 {
                    tunnel: w1257 -> [w1258 w1261]
                    tunnel: [w1258 w1260] -> w1256
                    frame False {
                    }
                    frame True {
                      n578 = Build Array (concatenate)(w1261, string[] ["Set Calibration INFO_C", "Reset Dongle", "Get Status"]) -> (w1260:string[])
                    }
                  }
                  n579 = local write "Set_INFO_C"(FALSE ("CCA Mode")) -> ()
                }
              }
            }
            frame 36 {
              # "Update CCA"
              n580 = case shown="True" "Get_INFO_D" {
                tunnel: w1264 -> [w1265 w1269]
                tunnel: [w1265 w1268] -> w1263
                frame False {
                }
                frame True {
                  n581 = local write "Get_INFO_D"(FALSE ("CCA Mode")) -> ()
                  n582 = Build Array (concatenate)(w1269, string[] ["Get Calibration INFO_D", "Get Status"]) -> (w1268:string[])
                }
              }
            }
            frame 37 {
              # "Update CCA"
              n583 = case shown="True" "Get_INFO_C" {
                tunnel: w1272 -> [w1273 w1277]
                tunnel: [w1273 w1276] -> w1271
                frame False {
                }
                frame True {
                  n584 = local write "Get_INFO_C"(FALSE ("CCA Mode")) -> ()
                  n585 = Build Array (concatenate)(w1277, string[] ["Get Calibration INFO_C", "Get Status"]) -> (w1276:string[])
                }
              }
            }
            frame 38 {
              # "Update CCA"
              n586 = case shown="True" "Get RSSI Base 400" {
                tunnel: w1280 -> [w1281 w1285]
                tunnel: [w1281 w1284] -> w1279
                frame False {
                }
                frame True {
                  n587 = local write "Get RSSI Base 400"(FALSE ("CCA Mode")) -> ()
                  n588 = Build Array (concatenate)(w1285, string[] ["Get RSSI Base 400", "Get Status"]) -> (w1284:string[])
                }
              }
            }
            frame 39 {
              # "Update CCA"
              n589 = case shown="True" "Get RSSI Remote 400" {
                tunnel: w1288 -> [w1289 w1293]
                tunnel: [w1289 w1292] -> w1287
                frame False {
                }
                frame True {
                  n590 = local write "Get RSSI Remote 400"(FALSE ("CCA Mode")) -> ()
                  n591 = Build Array (concatenate)(w1293, string[] ["Get RSSI Remote 400", "Get Status"]) -> (w1292:string[])
                }
              }
            }
            frame 40 {
              # "Update CCA"
              n592 = case shown="True" "ConstantsGet" {
                tunnel: w1296 -> [w1297 w1301]
                tunnel: [w1297 w1300] -> w1295
                frame False {
                }
                frame True {
                  n593 = local write "ConstantsGet"(FALSE ("CCA Mode")) -> ()
                  n594 = Build Array (concatenate)(w1301, string[] ["Get Device Data", "Get Status"]) -> (w1300:string[])
                }
              }
            }
            frame 41 {
              # "Update CCA"
              n595 = case shown="True" "Clear Device Data" {
                tunnel: w1304 -> [w1305 w1309]
                tunnel: [w1305 w1308] -> w1303
                frame False {
                }
                frame True {
                  n596 = local write "Clear Device Data"(FALSE ("CCA Mode")) -> ()
                  n597 = Build Array (concatenate)(w1309, string[] ["Clear Device Data", "Get Status"]) -> (w1308:string[])
                }
              }
            }
            frame 42 {
              # "Update CCA"
              n598 = case shown="True" "DevDataSave" {
                tunnel: w1312 -> [w1313 w1318]
                tunnel: [w1313 w1317] -> w1311
                frame False {
                }
                frame True {
                  n599 = case shown="False" "DevDataSaveAll" {
                    tunnel: [string[] ["Save All Device Data", "Get Status"] string[] ["Save Partial Device Data", "Get Status"]] -> w1315
                    frame True {
                    }
                    frame False {
                    }
                  }
                  n600 = local write "DevDataSave"(FALSE ("CCA Mode")) -> ()
                  n601 = Build Array (concatenate)(w1318, w1315) -> (w1317:string[])
                }
              }
            }
            frame 43 {
              # "Update CCA"
              n602 = case shown="True" "Get RSSI Remote 2.45" {
                tunnel: w1323 -> [w1324 w1328]
                tunnel: [w1324 w1327] -> w1322
                frame False {
                }
                frame True {
                  n603 = local write "Get RSSI Remote 2.45"(FALSE ("CCA Mode")) -> ()
                  n604 = Build Array (concatenate)(w1328, string[] ["2.45GHz Remote RSSI", "Get Status"]) -> (w1327:string[])
                }
              }
            }
            frame 44 {
              # "Update CCA"
              n605 = case shown="True" "Wakeup Cal Tool" {
                tunnel: w1331 -> [w1332 w1336]
                tunnel: [w1332 w1335] -> w1330
                frame False {
                }
                frame True {
                  n606 = local write "Wakeup Cal Tool"(FALSE ("CCA Mode")) -> ()
                  n607 = Build Array (concatenate)(w1336, string[] ["Wakeup Calibrator Tool", "Get Status"]) -> (w1335:string[])
                }
              }
            }
            frame 45 {
              # "Update CCA"
              n608 = case shown="True" "CopyDataToParams" {
                tunnel: w1339 -> [w1340 w1342]
                tunnel: [w1340 w1342] -> w1338
                frame False {
                }
                frame True {
                  n609 = local read "Data"() -> (w1341:string)
                  n610 = local write "Parameters"(w1341) -> ()
                  n611 = local write "CopyDataToParams"(FALSE ("CCA Mode")) -> ()
                }
              }
            }
            frame 46 {
              # "Update CCA"
              n612 = case shown="True" "ConstantsLoad" {
                tunnel: w1346 -> [w1347 w1351]
                tunnel: [w1347 w1350] -> w1345
                frame False {
                }
                frame True {
                  n613 = local write "ConstantsLoad"(FALSE ("CCA Mode")) -> ()
                  n614 = Build Array (concatenate)(w1351, string[] ["Clear Device Data", "Load All Device Data", "Get Status"]) -> (w1350:string[])
                }
              }
            }
            frame 47 {
              # "Update CCA"
              n615 = case shown="True" "Single Imp Meas" {
                tunnel: w1354 -> [w1355 w1359]
                tunnel: [w1355 w1358] -> w1353
                frame False {
                }
                frame True {
                  n616 = local write "Single Imp Meas"(FALSE ("CCA Mode")) -> ()
                  n617 = Build Array (concatenate)(w1359, string[] ["Single Imp Meas", "Get Status"]) -> (w1358:string[])
                }
              }
            }
            frame 48 {
              # "Update CCA"
              n618 = case shown="True" "Quick Imp Meas" {
                tunnel: w1362 -> [w1363 w1367]
                tunnel: [w1363 w1366] -> w1361
                frame False {
                }
                frame True {
                  n619 = local write "Quick Imp Meas"(FALSE ("CCA Mode")) -> ()
                  n620 = Build Array (concatenate)(w1367, string[] ["Simple Imp Scan", "Get Status"]) -> (w1366:string[])
                }
              }
            }
            frame 49 {
              # "Update CCA"
              n621 = case shown="True" "Matrix Imp Meas" {
                tunnel: w1370 -> [w1371 w1375]
                tunnel: [w1371 w1374] -> w1369
                frame False {
                }
                frame True {
                  n622 = local write "Matrix Imp Meas"(FALSE ("CCA Mode")) -> ()
                  n623 = Build Array (concatenate)(w1375, string[] ["Matrix Imp Scan", "Get Status"]) -> (w1374:string[])
                }
              }
            }
            frame 50 {
              # "Run RF Job"
              n624 = case shown="True" "Run RF Job" {
                tunnel: w1378 -> [w1379 w1383]
                tunnel: [w1379 w1382] -> w1377
                frame False {
                }
                frame True {
                  n625 = local write "Run RF Job"(FALSE ("CCA Mode")) -> ()
                  n626 = Build Array (concatenate)(w1383, string[] ["Wakeup Scan Config"]) -> (w1382:string[])
                }
              }
            }
            frame 51 {
              # "Save RF Job"
              n627 = case shown="True" "Save RF Job" {
                tunnel: w1386 -> [w1387 w1391]
                tunnel: [w1387 w1390] -> w1385
                frame False {
                }
                frame True {
                  n628 = local write "Save RF Job"(FALSE ("CCA Mode")) -> ()
                  n629 = Build Array (concatenate)(w1391, string[] ["Save RF Job", "Get Status"]) -> (w1390:string[])
                }
              }
            }
            frame 52 {
              # "Load RF Job"
              n630 = case shown="True" "Load RF Job" {
                tunnel: w1394 -> [w1395 w1399]
                tunnel: [w1395 w1398] -> w1393
                frame False {
                }
                frame True {
                  n631 = local write "Load RF Job"(FALSE ("CCA Mode")) -> ()
                  n632 = Build Array (concatenate)(w1399, string[] ["Load RF Job", "Get Status"]) -> (w1398:string[])
                }
              }
            }
            frame 53 {
              # "Load RF Job"
              n633 = case shown="True" "Save RF Scan Report" {
                tunnel: w1402 -> [w1403 w1407]
                tunnel: [w1403 w1406] -> w1401
                frame False {
                }
                frame True {
                  n634 = local write "Save RF Scan Report"(FALSE ("CCA Mode")) -> ()
                  n635 = Build Array (concatenate)(w1407, string[] ["Save RF Scan Report", "Get Status"]) -> (w1406:string[])
                }
              }
            }
            frame 54 {
              # "Update CCA"
              n636 = Compound Arithmetic op=OR("TelemGetStatus", "TelemGetIdentity", "TelemGetGenCals", "TelemGetZarlinkTrim1", "TelemTuneMICS", "TelemOpenLeadLimits", "TelemReset", "TelemStorage") -> (w1416:bool)
              n637 = case shown="True" w1416 {
                tunnel: w1418 -> [w1419 w1433]
                tunnel: [w1419 w1432] -> w1417
                tunnel: "TelemGetStatus" -> [_ w1427]
                tunnel: "TelemGetIdentity" -> [_ w1428]
                tunnel: "TelemGetGenCals" -> [_ w1429]
                tunnel: "TelemGetZarlinkTrim1" -> [_ w1430]
                tunnel: "TelemTuneMICS" -> [_ w1423]
                tunnel: "TelemOpenLeadLimits" -> [_ w1422]
                tunnel: "TelemReset" -> [_ w1421]
                tunnel: "TelemStorage" -> [_ w1420]
                frame False {
                }
                frame True {
                  w1424 = FALSE ("CCA Mode")
                  n638 = Build Array(w1427, w1428, w1429, w1430, w1423, w1422, w1421, w1420) -> (w1426:bool[])
                  n639 = Boolean Array To Number(Boolean array=w1426) -> (number=w1425:u32)
                  n640 = local write "TelemGetZarlinkTrim1"(w1424) -> ()
                  n641 = case shown="32" w1425 {
                    frame 0, Default {
                      n642 = One Button Dialog(message="Telem Driver QuickButton Error!!") -> ()  [unwired: 1 in, 1 out]
                    }
                    frame 1 {
                      n643 = local write "Parameters"("" ("Parameters")) -> ()
                      n644 = local write "Command"(Typedef_Command_List."Get xPG Status" ("Command")) -> ()
                    }
                    frame 2 {
                      n645 = local write "Parameters"("" ("Parameters")) -> ()
                      n646 = local write "Command"(Typedef_Command_List."Get xPG Identity" ("Command")) -> ()
                    }
                    frame 4 {
                      n647 = local write "Parameters"("" ("Parameters")) -> ()
                      n648 = local write "Command"(Typedef_Command_List."Get General Calibration" ("Command")) -> ()
                    }
                    frame 8 {
                      n649 = local write "Parameters"("List=1" ("Parameters")) -> ()
                      n650 = local write "Command"(Typedef_Command_List."Get Trim List" ("Command")) -> ()
                    }
                    frame 16 {
                      n651 = local write "Parameters"("" ("Parameters")) -> ()
                      n652 = local write "Command"(Typedef_Command_List."Tune MICS" ("Command")) -> ()
                    }
                    frame 32 {
                      n653 = local write "Parameters"("currentLimit[CH01]=15000\ncurrentLimit[CH02]=15000\ncurrentLimit[CH03]=15000\ncurrentLimit[CH04]=15000\ncurrentLimit[CH05]=15000\ncurrentLimit[CH06]=15000\ncurrentLimit[CH07]=15000\ncurrentLimit[CH08]=15000\ncurrentLimit[CH09]=15000\ncurrentLimit[CH10]=15000\ncurrentLimit[CH11]=15000\ncurrentLimit[CH12]=15000\ncurrentLimit[CH13]=15000\ncurrentLimit[CH14]=15000\ncurrentLimit[CH15]=15000\ncurrentLimit[CH16]=15000\ncurrentLimit[CH17]=15000\ncurrentLimit[CH18]=15000\ncurrentLimit[CH19]=15000\ncurrentLimit[CH20]=15000\ncurrentLimit[CH21]=15000\ncurrentLimit[CH22]=15000\ncurrentLimit[CH23]=15000\ncurrentLimit[CH24]=15000\ncurrentLimit[CH25]=15000\ncurrentLimit[CH26]=15000\nchargeLimit[CH01]=22500\nchargeLimit[CH02]=22500\nchargeLimit[CH03]=22500\nchargeLimit[CH04]=22500\nchargeLimit[CH05]=22500\nchargeLimit[CH06]=22500\nchargeLimit[CH07]=22500\nchargeLimit[CH08]=22500\nchargeLimit[CH09]=22500\nchargeLimit[CH10]=22500\nchargeLimit[CH11]=22500\nchargeLimit[CH12]=22500\nchargeLimit[CH13]=22500\nchargeLimit[CH14]=22500\nchargeLimit[CH15]=22500\nchargeLimit[CH16]=22500\nchargeLimit[CH17]=22500\nchargeLimit[CH18]=22500\nchargeLimit[CH19]=22500\nchargeLimit[CH20]=22500\nchargeLimit[CH21]=22500\nchargeLimit[CH22]=22500\nchargeLimit[CH23]=22500\nchargeLimit[CH24]=22500\nchargeLimit[CH25]=22500\nchargeLimit[CH26]=22500" ("Parameters")) -> ()
                      n654 = local write "Command"(Typedef_Command_List."Set Lead Limits" ("Command")) -> ()
                    }
                    frame 64 {
                      n655 = local write "Parameters"("" ("Parameters")) -> ()
                      n656 = local write "Command"(Typedef_Command_List."Reset xPG" ("Command")) -> ()
                    }
                    frame 128 {
                      n657 = local write "Parameters"("" ("Parameters")) -> ()
                      n658 = local write "Command"(Typedef_Command_List."Enter Storage Mode" ("Command")) -> ()
                    }
                  }
                  n659 = local write "TelemGetIdentity"(w1424) -> ()
                  n660 = local write "TelemGetGenCals"(w1424) -> ()
                  n661 = local write "TelemGetStatus"(w1424) -> ()
                  n662 = local write "TelemOpenLeadLimits"(w1424) -> ()
                  n663 = local write "TelemTuneMICS"(w1424) -> ()
                  n664 = local write "TelemStorage"(w1424) -> ()
                  n665 = local write "TelemReset"(w1424) -> ()
                  n666 = Build Array (concatenate)(w1433, string[] ["Telem Driver", "Get Status"]) -> (w1432:string[])
                }
              }
            }
          }
        }
        n667 = Wait (ms)(milliseconds to wait=u32 100) -> ()  [unwired: 1 out]
        n668 = Array Size(array=w913) -> (size(s)=w912:i32)
        n669 = Greater?(x=w912, y=1) -> (0:w910:bool)
        n670 = property on="Busy Flag" class="Str"("Visible"=w910) -> ()  [unwired: 2 in, 2 out]
        n671 = property on="RFScanStat" class="Clust (strict)"("DisabledEnum"=T23."Disabled and Grayed Out" ("Disabled")) -> ()  [unwired: 2 in, 2 out]
        n672 = local write "RFST"(u8 0) -> ()
      }
      frame "Get Status" {
        n673 = local read "SESSION CONTROL"() -> (w1462:T3)
        n674 = invoke on="Detected MICS IDs" class="LstBox (strict)" method="Get DblClk Row"() -> ("Get DblClk Row"=w1459:i32)  [unwired: 3 in, 2 out]
        n675 = property on="Detected MICS IDs" class="LstBox (strict)"() -> ("Item Names"=w1465:string[])  [unwired: 2 in, 2 out]
        n676 = Tick Count (ms)() -> (millisecond timer value=w1478:u32)
        n677 = flat-sequence {
          tunnel: w1477 -> [w1597]
          tunnel: [w1597] -> w1476
          frame #0 {
            n678 = Wait (ms)(milliseconds to wait=u32 20) -> ()  [unwired: 1 out]
          }
        }
        n679 = property on="Busy Flag" class="Str"("Visible"=FALSE) -> ()  [unwired: 2 in, 2 out]
        n680 = local write "Tick Count"(w1478) -> ()
        n681 = call "MICSD Status.vi"("VISA Resource Name"=w1480, "error in (no error)"=w1476) -> ("Data Status"=→"DATA STATUS":T5, "dup VISA Resource Name"=w1467:refnum<visa-resource-name>, "Status Flags"=w1483:T6, "Link Status"=→"LINK STATUS":T7, "Link Quality"=w1453:T4, "error out"=w1475:errorcluster)  [unwired: 7 in, 1 out]
        "LINK QUALITY" <- w1453
        "STATUS FLAGS" <- w1483
        "LINK QUALITY MONITOR" <- w1453
        n682 = Equal?(x=w1459, y=-2) -> (x = y?=w1456:bool)
        n683 = Index Array(array=w1465, index=w1459) -> (element=w1464:string)
        n684 = Unbundle By Name(w1483) -> ("ERROR_OCCURRED"=→"ERROR":bool, "IDLE"=→"IDLE":bool, "IN_SESSION"=w1455:bool)
        "SESSION" <- w1455
        n685 = Hexadecimal String To Number(string=w1464) -> (number=w1463:u32)  [unwired: 2 in, 1 out]
        n686 = Bundle By Name(cluster=w1462, "TARGET MICS ID"=w1463) -> (w1461:T3)
        n687 = Unbundle By Name(w1453) -> ("Corrected Blocks"=→"Corrected Blocks":u16, "CRC Errors"=→"CRC Errors":u16)
        n688 = Unbundle By Name(w1453) -> ("MAX_RETRIES"=→"MAX_RETRIES":bool)
        n689 = Or(x=w1456, y=w1455) -> (x .or. y?=w1457:bool)
        n690 = Or(x="Get VBAT Cont", y="Get VBAT Single") -> (x .or. y?=w1471:bool)
        n691 = Select(t=w1462, s=w1457, f=w1461) -> (s? t:f=w1460:T3)
        n692 = local write "SESSION CONTROL"(w1460) -> ()
        n693 = Unbundle By Name(w1460) -> ("TARGET MICS ID"=w1466:u32)
        n694 = flat-sequence {
          tunnel: w1475 -> [w1595]
          tunnel: [w1595] -> w1469
          frame #0 {
            n695 = Wait (ms)(milliseconds to wait=u32 20) -> ()  [unwired: 1 out]
          }
        }
        n696 = And(x=w1455, y=w1471) -> (x .and. y?=w1470:bool)
        n697 = while {
          tunnel: w1470 -> [w1494]
          tunnel: w1467 -> [w1491]
          tunnel: w1466 -> [w1490]
          shift-right: [w1492] -> w1468
          shift-left: w1469 -> [w1493]
          stop <- w1489 stop-if-true
          n698 = local read "VBAT Cal"() -> (w1487:dbl)
          n699 = Greater Than 0?(x=w1487) -> (x > 0?=w1488:bool)
          n700 = case shown="True" w1494 {
            tunnel: w1493 -> [w1497 w1503]
            tunnel: [w1497 w1504] -> w1492
            tunnel: w1491 -> [_ w1502]
            tunnel: w1487 -> [_ w1499]
            tunnel: w1488 -> [_ w1501]
            tunnel: w1490 -> [_ w1500]
            tunnel: [TRUE w1498] -> w1489
            frame False {
              n701 = local write "Get VBAT Cont"(FALSE ("Get VBAT Cont")) -> ()
            }
            frame True {
              n702 = case shown="True" w1501 {
                tunnel: [w1530 w1539] -> w1504
                tunnel: w1503 -> [w1531 w1538]
                tunnel: w1502 -> [w1525 w1537]
                tunnel: w1500 -> [w1526 _]
                tunnel: w1499 -> [_ w1536]
                tunnel: [FALSE TRUE] -> w1498
                frame False {
                  w1505 = 51060  # WARN Threshold ideal ohms
                  w1510 = 1.0  # Default T1 CF
                  w1516 = 16  # WARN Threshold (40C)
                  n703 = Bundle By Name(cluster=T21 {"Command"=enum."Get xPG Status", "Function"=enum."Downlink Only", "MICS_ID"=0, "EXID"=16773121, "Use Local"=FALSE, "Transceive Delay mS"=200.0, "CP_DATA IN"=[], "Parameters"=""} ("Input"), "Command"=Typedef_Command_List."Get General Calibration", "Function"=T22."Transceive (DN -> UP)", "MICS_ID"=w1526) -> (w1533:T21)
                  n704 = call "Zarlink Telemetry.vi"("error in (no error)"=w1531, "Input"=w1533, "MICS Dongle Address"=w1525) -> ("error out"=w1530:errorcluster, "Output"=w1534:T28)  [unwired: 6 in, 1 out]
                  n705 = Unbundle By Name(w1534) -> ("Data"=w1517:string)
                  n706 = Pick Line(multi-line string=w1517, line index=w1516) -> (output string=w1515:string)  [unwired: 1 in]
                  n707 = Pick Line(multi-line string=w1517, line index=43) -> (output string=w1524:string)  [unwired: 1 in]
                  n708 = Match Pattern(string=w1524, regular expression="=0x") -> (after substring=w1522:string)  [unwired: 1 in, 3 out]
                  n709 = Match Pattern(string=w1515, regular expression="=0x") -> (after substring=w1513:string)  [unwired: 1 in, 3 out]
                  n710 = Hexadecimal String To Number(string=w1522) -> (number=w1521:u32)  [unwired: 2 in, 1 out]
                  n711 = Hexadecimal String To Number(string=w1513) -> (number=w1509:u32)  [unwired: 2 in, 1 out]
                  n712 = Divide(x=3.85, y=w1521) -> (x/y=→"VBAT Cal":dbl)
                  n713 = Multiply(x=u32 4, y=w1509) -> (x*y=w1506:u32)
                  n714 = Divide(x=w1505, y=w1506) -> (x/y=w1507:dbl)
                  n715 = Greater Than 0?(x=w1509) -> (x > 0?=w1512:bool)
                  "Temp Cal" <- w1512
                  n716 = Select(t=w1507, s=w1512, f=w1510) -> (s? t:f=→"T1 Cal Factor":dbl)
                }
                frame True {
                  n717 = stacked-sequence {
                    seq-local: [w1540 _] -> [_ w1584]
                    tunnel: [_ w1592] -> w1539
                    tunnel: w1538 -> [w1573 _]
                    tunnel: w1537 -> [w1571 w1583]
                    tunnel: w1536 -> [w1569 _]
                    frame #0 {
                      w1564 = "=" ("regular expression")
                      n718 = call "MICSD Telem Driver.vi"("VISA Resource Name"=w1571, "Command"=Typedef_Command_List."Charging Control", "error in (no error)"=w1573) -> ("Data"=w1543:string, "error out"=w1572:errorcluster)  [unwired: 10 in, 5 out]
                      "Charging Status" <- w1543
                      n719 = Pick Line(multi-line string=w1543, line index=0) -> (output string=w1559:string)  [unwired: 1 in]
                      n720 = Pick Line(multi-line string=w1543, line index=3) -> (output string=w1565:string)  [unwired: 1 in]
                      n721 = Pick Line(multi-line string=w1543, line index=2) -> (output string=w1552:string)  [unwired: 1 in]
                      n722 = Pick Line(multi-line string=w1543, line index=2) -> (output string=w1544:string)  [unwired: 1 in]
                      n723 = call "MICSD Telem Driver.vi"("VISA Resource Name"=w1571, "Command"=Typedef_Command_List."Get VBAT", "error in (no error)"=w1572) -> ("Data"=w1576:string, "error out"=w1540:errorcluster)  [unwired: 10 in, 5 out]
                      n724 = Match Pattern(string=w1552, regular expression="=") -> (after substring=w1551:string)  [unwired: 1 in, 3 out]
                      n725 = Match Pattern(string=w1544, regular expression="=YES") -> (offset past match=w1542:i32)  [unwired: 1 in, 3 out]
                      n726 = Match Pattern(string=w1559, regular expression="-") -> (after substring=w1558:string)  [unwired: 1 in, 3 out]
                      n727 = Match Pattern(string=w1565, regular expression=w1564) -> (after substring=w1563:string)  [unwired: 1 in, 3 out]
                      n728 = Greater Than 0?(x=w1542) -> (x > 0?=→"Charge/Temp Warning":bool)
                      n729 = Decimal String To Number(string=w1551) -> (number=w1550:i32)  [unwired: 2 in, 1 out]
                      n730 = Match Pattern(string=w1576, regular expression=w1564) -> (after substring=w1575:string)  [unwired: 1 in, 3 out]
                      n731 = Decimal String To Number(string=w1558) -> (number=w1557:i32)  [unwired: 2 in, 1 out]
                      n732 = Decimal String To Number(string=w1563) -> (number=→"VRECT Input Power":i32)  [unwired: 2 in, 1 out]
                      n733 = Decrement(x=w1550) -> (x-1=w1547:i32)
                      n734 = local write "Get VBAT Single"(FALSE ("Get VBAT Single")) -> ()
                      n735 = Decimal String To Number(string=w1575) -> (number=w1574:i32)  [unwired: 2 in, 1 out]
                      "ADC Counts" <- w1574
                      n736 = Pick Line(multi-line string="NORMAL\nWARN\nCRITICAL\nABORT", line index=w1547) -> (output string=→"Reported Temperature Status":string)  [unwired: 1 in]
                      n737 = Pick Line(multi-line string="OFF\nPRECOND\nCC-FAST\nCC-SLOW\nDONE\nERROR\nIND (6)\nIND (7)", line index=w1557) -> (output string=→"Reported Charging Status":string)  [unwired: 1 in]
                      n738 = Multiply(x=w1574, y=w1569) -> (x*y=→"VBAT (Volts)" →"Battery Status (Volts)":dbl)
                    }
                    frame #1 {
                      n739 = call "MICSD Telem Driver.vi"("VISA Resource Name"=w1583, "Command"=Typedef_Command_List."Diagnostic Data", "Parameters"="command=0\nselect=3", "error in (no error)"=w1584) -> ("Data"=w1591:string, "error out"=w1592:errorcluster)  [unwired: 9 in, 5 out]
                      n740 = Scan From String(format string="ThermBias=%d ThermInput=%d ThermOffset=%d", input string=w1591) -> (output 1=w1580:u16, output 2=w1579:u16, output 3=w1578:u16)  [unwired: 5 in, 3 out]
                      "Input" <- w1579
                      "Bias" <- w1580
                      "Offset" <- w1578
                      n741 = Subtract(x=w1579, y=w1578) -> (x-y=w1588:u16)
                      n742 = Subtract(x=w1580, y=w1579) -> (x-y=w1589:u16)
                      n743 = Divide(x=w1588, y=w1589) -> (x/y=w1587:dbl)
                      n744 = Multiply(x=w1587, y=47000.0) -> (x*y=w1582:dbl)
                      "T1 Ohms" <- w1582
                      n745 = call "Thermistor, SP21629.vi"("resistance (ohms)"=w1582) -> ("temperature (C)"=→"Thermometer" →"TEMP (°C)" →"Temperature History":dbl)  [unwired: 9 in, 1 out]
                    }
                  }
                }
              }
            }
          }
        }
      }
      frame "Get Device Data" {
        n746 = local read "SESSION CONTROL"() -> (w1604:T3)
        n747 = Unbundle By Name(w1604) -> ("TARGET MICS ID"=w1603:u32)
        n748 = Not(x="ConstGetAll") -> (.not. x?=w1600:bool)
        n749 = while {
          tunnel: w1600 -> [w1620]
          tunnel: "DevDataTabs" -> [w1619]
          tunnel: w1603 -> [w1624]
          shift-right: [w1611] -> w1605
          shift-left: w1606 -> [w1613]
          tunnel: w1602 -> [w1623]
          tunnel: [w1623] -> w1601
          tunnel: 12 ("y") -> [w1622]
          i -> [w1618]
          stop <- w1627 stop-if-true
          n750 = Greater?(x=w1618, y=w1622) -> (0:w1621:bool)
          n751 = call <vilib>:"Set Busy.vi"("error in (no error)"=w1613) -> ("error out"=w1612:errorcluster)  [unwired: 9 in, 1 out]
          n752 = Select(t=w1619, s=w1620, f=w1618) -> (s? t:f=w1626:u32)
          n753 = case shown="3" w1626 {
            tunnel: w1612 -> [w1640 w1699 w1751 w1762 w1773 w1784 w1795 w1804 w1846 w1890 w1901 w1912 w1946 w2001]
            tunnel: [w1646 w1686 w1750 w1761 w1772 w1783 w1794 w1803 w1845 w1889 w1900 w1911 w1945 w2000] -> w1610
            tunnel: T21 {"Command"=enum."Get xPG Status", "Function"=enum."Transceive (DN -> UP)", "MICS_ID"=0, "EXID"=16773121, "Use Local"=FALSE, "Transceive Delay mS"=200.0, "CP_DATA IN"=[], "Parameters"=""} ("Input") -> [w1641 w1687 w1752 w1763 w1774 w1785 w1796 w1805 w1847 w1891 w1902 w1913 w1947 w2002]
            tunnel: w1624 -> [w1630 w1688 w1745 w1757 w1768 w1779 w1790 w1802 w1844 w1885 w1896 w1910 w1944 w1999]
            tunnel: w1623 -> [w1638 w1690 w1744 w1756 w1767 w1778 w1789 w1801 w1843 w1884 w1895 w1909 w1943 w1998]
            tunnel: w1620 -> [_ _ _ _ _ _ _ w1800 w1842 _ _ _ w1942 w1997]
            tunnel: [w1636 w1693 w1742 w1753 w1764 w1775 w1786 w1797 w1839 w1881 w1892 w1907 w1939 w1994] -> w1616
            tunnel: [w1637 w1694 w1743 w1754 w1765 w1776 w1787 w1798 w1840 w1882 w1893 w1908 w1940 w1995] -> w1615
            frame 0 {
              # "Read Activity Log"
              n754 = Bundle(cluster=w1641, "Command"=Typedef_Command_List."Get Log Range", "MICS_ID"=w1630, "Parameters"="Log=1") -> (w1645:T21)  [unwired: 5 in]
              n755 = call "Zarlink Telemetry.vi"("error in (no error)"=w1640, "Input"=w1645, "MICS Dongle Address"=w1638) -> ("error out"=w1639:errorcluster, "Output"=w1644:T28)  [unwired: 6 in, 1 out]
              n756 = Unbundle(w1644) -> ("Response Token"=w1634:string, "Response Code"=w1633:string, "Data"=w1631:string)  [unwired: 3 out]
              n757 = Concatenate Strings(w1634, " - ", w1633) -> (w1632:string)
              n758 = local write "Response"(w1632) -> ()
              n759 = while {
                tunnel: w1630 -> [w1681]
                tunnel: [w1675] -> w1637
                tunnel: [w1676] -> w1636
                tunnel: w1641 -> [w1680]
                tunnel: w1638 -> [w1678]
                shift-right: [w1667] -> w1646
                shift-left: w1639 -> [w1679]
                shift-right: [w1672] -> w1629
                shift-left: w1631 -> [w1673]
                shift-right: [w1649] -> _
                shift-left: i64 0 -> [w1651]
                stop <- w1658 stop-if-true
                w1648 = 42
                w1668 = "\r\n"
                # "Read Activity Log"
                n760 = Number To Decimal String(number=w1651) -> (decimal integer string=w1669:string)  [unwired: 1 in]
                n761 = Concatenate Strings("Log=1\nSerial=" ("Parameters"), w1669) -> (w1671:string)
                n762 = Bundle(cluster=w1680, "Command"=Typedef_Command_List."Read Log", "MICS_ID"=w1681, "Parameters"=w1671) -> (w1684:T21)  [unwired: 5 in]
                n763 = call "Zarlink Telemetry.vi"("error in (no error)"=w1679, "Input"=w1684, "MICS Dongle Address"=w1678) -> ("error out"=w1666:errorcluster, "Output"=w1683:T28)  [unwired: 6 in, 1 out]
                n764 = Unbundle(w1683) -> ("Response Token"=w1676:string, "Response Code"=w1675:string, "Data"=w1652:string)  [unwired: 3 out]
                n765 = Pick Line(multi-line string=w1652, line index=i64 1 ("default (0 I32)")) -> (output string=w1662:string)  [unwired: 1 in]
                n766 = Pick Line(multi-line string=w1652, line index=i64 2 ("default (0 I32)")) -> (output string=w1655:string)  [unwired: 1 in]
                n767 = Match Pattern(string=w1662, regular expression="Count=") -> (after substring=w1663:string)  [unwired: 1 in, 3 out]
                n768 = Match Pattern(string=w1655, regular expression="Serial=") -> (after substring=w1656:string)  [unwired: 1 in, 3 out]
                n769 = Concatenate Strings(w1676, " - ", w1675) -> (w1674:string)
                n770 = local write "Response"(w1674) -> ()
                n771 = Decimal String To Number(string=w1663, default (0L)=i64 -1 ("default (0 I32)")) -> (number=w1657:i64)  [unwired: 1 in, 1 out]
                n772 = Decimal String To Number(string=w1656, default (0L)=i64 0 ("default (0 I32)")) -> (number=w1650:i64)  [unwired: 1 in, 1 out]
                n773 = Less Than 0?(x=w1657) -> (x < 0?=w1665:bool)
                n774 = Less?(x=w1657, y=w1648) -> (x < y?=w1658:bool)
                n775 = Add(x=w1648, y=w1650) -> (x+y=w1649:i64)
                n776 = Concatenate Strings(w1673, w1668, w1668, w1652) -> (w1672:string)
                n777 = Select(t=errorcluster {"status"=TRUE, "code"=100, "source"="Invalid \"Log Count\" received from device, Activity Log"}, s=w1665, f=w1666) -> (s? t:f=w1667:errorcluster)
              }
              "Activity Log" <- w1629
            }
            frame 1 {
              # "Read Error Log"
              n778 = Bundle(cluster=w1687, "Command"=Typedef_Command_List."Get Log Range", "MICS_ID"=w1688, "Parameters"="Log=0") -> (w1703:T21)  [unwired: 5 in]
              n779 = call "Zarlink Telemetry.vi"("error in (no error)"=w1699, "Input"=w1703, "MICS Dongle Address"=w1690) -> ("error out"=w1689:errorcluster, "Output"=w1702:T28)  [unwired: 6 in, 1 out]
              n780 = Unbundle(w1702) -> ("Response Token"=w1697:string, "Response Code"=w1696:string, "Data"=w1691:string)  [unwired: 3 out]
              n781 = Concatenate Strings(w1697, " - ", w1696) -> (w1695:string)
              n782 = local write "Response"(w1695) -> ()
              n783 = while {
                tunnel: w1688 -> [w1738]
                tunnel: [w1732] -> w1694
                tunnel: [w1733] -> w1693
                tunnel: w1687 -> [w1737]
                tunnel: w1690 -> [w1735]
                shift-right: [w1724] -> w1686
                shift-left: w1689 -> [w1736]
                shift-right: [w1729] -> w1692
                shift-left: w1691 -> [w1730]
                shift-right: [w1706] -> _
                shift-left: i64 0 -> [w1708]
                stop <- w1715 stop-if-true
                w1705 = 42
                w1725 = "\r\n"
                # "Read Error Log"
                n784 = Number To Decimal String(number=w1708) -> (decimal integer string=w1726:string)  [unwired: 1 in]
                n785 = Concatenate Strings("Log=0\nSerial=" ("Parameters"), w1726) -> (w1728:string)
                n786 = Bundle(cluster=w1737, "Command"=Typedef_Command_List."Read Log", "MICS_ID"=w1738, "Parameters"=w1728) -> (w1741:T21)  [unwired: 5 in]
                n787 = call "Zarlink Telemetry.vi"("error in (no error)"=w1736, "Input"=w1741, "MICS Dongle Address"=w1735) -> ("error out"=w1723:errorcluster, "Output"=w1740:T28)  [unwired: 6 in, 1 out]
                n788 = Unbundle(w1740) -> ("Response Token"=w1733:string, "Response Code"=w1732:string, "Data"=w1709:string)  [unwired: 3 out]
                n789 = Pick Line(multi-line string=w1709, line index=i64 1 ("default (0 I32)")) -> (output string=w1719:string)  [unwired: 1 in]
                n790 = Pick Line(multi-line string=w1709, line index=i64 2 ("default (0 I32)")) -> (output string=w1712:string)  [unwired: 1 in]
                n791 = Match Pattern(string=w1719, regular expression="Count=") -> (after substring=w1720:string)  [unwired: 1 in, 3 out]
                n792 = Match Pattern(string=w1712, regular expression="Serial=") -> (after substring=w1713:string)  [unwired: 1 in, 3 out]
                n793 = Concatenate Strings(w1733, " - ", w1732) -> (w1731:string)
                n794 = local write "Response"(w1731) -> ()
                n795 = Decimal String To Number(string=w1720, default (0L)=i64 -1 ("default (0 I32)")) -> (number=w1714:i64)  [unwired: 1 in, 1 out]
                n796 = Decimal String To Number(string=w1713, default (0L)=i64 0 ("default (0 I32)")) -> (number=w1707:i64)  [unwired: 1 in, 1 out]
                n797 = Less Than 0?(x=w1714) -> (x < 0?=w1722:bool)
                n798 = Less?(x=w1714, y=w1705) -> (x < y?=w1715:bool)
                n799 = Add(x=w1705, y=w1707) -> (x+y=w1706:i64)
                n800 = Concatenate Strings(w1730, w1725, w1725, w1709) -> (w1729:string)
                n801 = Select(t=errorcluster {"status"=TRUE, "code"=100, "source"="Invalid \"Log Count\" received from device, Error Log"}, s=w1722, f=w1723) -> (s? t:f=w1724:errorcluster)
              }
              "Error Log" <- w1692
            }
            frame 2 {
              n802 = Bundle(cluster=w1752, "Command"=Typedef_Command_List."Get xPG Identity", "MICS_ID"=w1745) -> (w1749:T21)  [unwired: 6 in]
              n803 = call "Zarlink Telemetry.vi"("error in (no error)"=w1751, "Input"=w1749, "MICS Dongle Address"=w1744) -> ("error out"=w1750:errorcluster, "Output"=w1748:T28)  [unwired: 6 in, 1 out]
              n804 = Unbundle(w1748) -> ("Response Token"=w1742:string, "Response Code"=w1743:string, "Data"=→"xPG Identity Data":string)  [unwired: 3 out]
            }
            frame 3 {
              n805 = Bundle(cluster=w1763, "Command"=Typedef_Command_List."Get General Calibration", "MICS_ID"=w1757) -> (w1760:T21)  [unwired: 6 in]
              n806 = call "Zarlink Telemetry.vi"("error in (no error)"=w1762, "Input"=w1760, "MICS Dongle Address"=w1756) -> ("error out"=w1761:errorcluster, "Output"=w1759:T28)  [unwired: 6 in, 1 out]
              n807 = Unbundle(w1759) -> ("Response Token"=w1753:string, "Response Code"=w1754:string, "Data"=→"General Calibration Data":string)  [unwired: 3 out]
            }
            frame 4, Default {
              n808 = Bundle(cluster=w1774, "Command"=Typedef_Command_List."Get Pulse Constants", "MICS_ID"=w1768) -> (w1771:T21)  [unwired: 6 in]
              n809 = call "Zarlink Telemetry.vi"("error in (no error)"=w1773, "Input"=w1771, "MICS Dongle Address"=w1767) -> ("error out"=w1772:errorcluster, "Output"=w1770:T28)  [unwired: 6 in, 1 out]
              n810 = Unbundle(w1770) -> ("Response Token"=w1764:string, "Response Code"=w1765:string, "Data"=→"Pulse Constants Data":string)  [unwired: 3 out]
            }
            frame 5 {
              n811 = Bundle(cluster=w1785, "Command"=Typedef_Command_List."Get Program Constants", "MICS_ID"=w1779) -> (w1782:T21)  [unwired: 6 in]
              n812 = call "Zarlink Telemetry.vi"("error in (no error)"=w1784, "Input"=w1782, "MICS Dongle Address"=w1778) -> ("error out"=w1783:errorcluster, "Output"=w1781:T28)  [unwired: 6 in, 1 out]
              n813 = Unbundle(w1781) -> ("Response Token"=w1775:string, "Response Code"=w1776:string, "Data"=→"Program Constants Data":string)  [unwired: 3 out]
            }
            frame 6 {
              n814 = Bundle(cluster=w1796, "Command"=Typedef_Command_List."Get Stim Asic HV Calibrations", "MICS_ID"=w1790) -> (w1793:T21)  [unwired: 6 in]
              n815 = call "Zarlink Telemetry.vi"("error in (no error)"=w1795, "Input"=w1793, "MICS Dongle Address"=w1789) -> ("error out"=w1794:errorcluster, "Output"=w1792:T28)  [unwired: 6 in, 1 out]
              n816 = Unbundle(w1792) -> ("Response Token"=w1786:string, "Response Code"=w1787:string, "Data"=→"HV Calibrations Data":string)  [unwired: 3 out]
            }
            frame 7 {
              n817 = while {
                tunnel: w1805 -> [w1826]
                tunnel: w1802 -> [w1820]
                tunnel: w1801 -> [w1819]
                shift-right: [w1824] -> w1803
                shift-left: w1804 -> [w1825]
                tunnel: w1800 -> [w1815]
                tunnel: "ChanCalTabs" -> [w1810]
                tunnel: [w1807] -> w1798
                tunnel: [w1806] -> w1797
                i -> [w1811]
                stop <- w1814 stop-if-true
                n818 = Select(t=w1810, s=w1815, f=w1811) -> (s? t:f=w1813:u32)
                n819 = Greater?(x=w1811, y=2) -> (0:w1817:bool)
                n820 = case shown="3" w1813 {
                  tunnel: [Typedef_Command_List."Get Channel Calibrations" ("Command") Typedef_Command_List."Get Channel Calibrations" ("Command") Typedef_Command_List."Get Channel Calibrations" ("Command") Typedef_Command_List."Get Channel Calibrations" ("Command")] -> w1821
                  tunnel: ["List=0" ("Parameters") "List=1" ("Parameters") "List=2" ("Parameters") "List=3" ("Parameters")] -> w1816
                  frame 0, Default {
                  }
                  frame 1 {
                  }
                  frame 2 {
                  }
                  frame 3 {
                  }
                }
                n821 = Or(x=w1817, y=w1815) -> (x .or. y?=w1814:bool)
                n822 = Bundle(cluster=w1826, "Command"=w1821, "MICS_ID"=w1820, "Parameters"=w1816) -> (w1823:T21)  [unwired: 5 in]
                n823 = call "Zarlink Telemetry.vi"("error in (no error)"=w1825, "Input"=w1823, "MICS Dongle Address"=w1819) -> ("error out"=w1824:errorcluster, "Output"=w1822:T28)  [unwired: 6 in, 1 out]
                n824 = Unbundle(w1822) -> ("Response Token"=w1806:string, "Response Code"=w1807:string, "Data"=w1812:string)  [unwired: 3 out]
                n825 = case shown="0, Default" w1813 {
                  tunnel: w1812 -> [w1827 w1828 w1829 w1830]
                  frame 0, Default {
                    "Channel Cals 0-3mA" <- w1827
                  }
                  frame 1 {
                    "Channel Cals 3-6mA" <- w1828
                  }
                  frame 2 {
                    "Channel Cals 6-9mA" <- w1829
                  }
                  frame 3 {
                    "Channel Cals 9-15mA" <- w1830
                  }
                }
                n826 = Concatenate Strings(w1806, " - ", w1807) -> (w1808:string)
                n827 = local write "Response"(w1808) -> ()
              }
            }
            frame 8 {
              n828 = while {
                tunnel: w1847 -> [w1868]
                tunnel: w1844 -> [w1862]
                tunnel: w1843 -> [w1861]
                shift-right: [w1866] -> w1845
                shift-left: w1846 -> [w1867]
                tunnel: w1842 -> [w1857]
                tunnel: "TrimListTabs" -> [w1852]
                tunnel: [w1849] -> w1840
                tunnel: [w1848] -> w1839
                i -> [w1853]
                stop <- w1856 stop-if-true
                n829 = Select(t=w1852, s=w1857, f=w1853) -> (s? t:f=w1855:u32)
                n830 = Greater?(x=w1853, y=2) -> (0:w1859:bool)
                n831 = case shown="0, Default" w1855 {
                  tunnel: [Typedef_Command_List."Get Trim List" ("Command") Typedef_Command_List."Get Trim List" ("Command") Typedef_Command_List."Get Trim List" ("Command") Typedef_Command_List."Get Trim List" ("Command")] -> w1863
                  tunnel: ["List=0" ("Parameters") "List=1" ("Parameters") "List=2" ("Parameters") "List=3" ("Parameters")] -> w1858
                  frame 0, Default {
                  }
                  frame 1 {
                  }
                  frame 2 {
                  }
                  frame 3 {
                  }
                }
                n832 = Or(x=w1859, y=w1857) -> (x .or. y?=w1856:bool)
                n833 = Bundle(cluster=w1868, "Command"=w1863, "MICS_ID"=w1862, "Parameters"=w1858) -> (w1865:T21)  [unwired: 5 in]
                n834 = call "Zarlink Telemetry.vi"("error in (no error)"=w1867, "Input"=w1865, "MICS Dongle Address"=w1861) -> ("error out"=w1866:errorcluster, "Output"=w1864:T28)  [unwired: 6 in, 1 out]
                n835 = Unbundle(w1864) -> ("Response Token"=w1848:string, "Response Code"=w1849:string, "Data"=w1854:string)  [unwired: 3 out]
                n836 = case shown="0, Default" w1855 {
                  tunnel: w1854 -> [w1869 w1870 w1871 w1872]
                  frame 0, Default {
                    "Trim List 0" <- w1869
                  }
                  frame 1 {
                    "Trim List 1" <- w1870
                  }
                  frame 2 {
                    "Trim List 2" <- w1871
                  }
                  frame 3 {
                    "Trim List 3" <- w1872
                  }
                }
                n837 = Concatenate Strings(w1848, " - ", w1849) -> (w1850:string)
                n838 = local write "Response"(w1850) -> ()
              }
            }
            frame 9 {
              n839 = Bundle(cluster=w1891, "Command"=Typedef_Command_List."Get Lead Limits", "MICS_ID"=w1885) -> (w1888:T21)  [unwired: 6 in]
              n840 = call "Zarlink Telemetry.vi"("error in (no error)"=w1890, "Input"=w1888, "MICS Dongle Address"=w1884) -> ("error out"=w1889:errorcluster, "Output"=w1887:T28)  [unwired: 6 in, 1 out]
              n841 = Unbundle(w1887) -> ("Response Token"=w1881:string, "Response Code"=w1882:string, "Data"=→"Lead Limits":string)  [unwired: 3 out]
            }
            frame 10 {
              n842 = Bundle(cluster=w1902, "Command"=Typedef_Command_List."Get Configurable Device Parameters", "MICS_ID"=w1896) -> (w1899:T21)  [unwired: 6 in]
              n843 = call "Zarlink Telemetry.vi"("error in (no error)"=w1901, "Input"=w1899, "MICS Dongle Address"=w1895) -> ("error out"=w1900:errorcluster, "Output"=w1898:T28)  [unwired: 6 in, 1 out]
              n844 = Unbundle(w1898) -> ("Response Token"=w1892:string, "Response Code"=w1893:string, "Data"=→"Configurable Device Params":string)  [unwired: 3 out]
            }
            frame 11 {
              n845 = for {
                N: 14 -> [_]
                tunnel: w1913 -> [w1938]
                tunnel: w1912 -> [w1937]
                tunnel: [w1936] -> w1911
                tunnel: w1910 -> [w1932]
                tunnel: w1909 -> [w1931]
                tunnel: [w1919] -> w1908
                tunnel: [w1920] -> w1907
                shift-right: [w1926] -> w1903
                shift-left: "Event Counters Read=14\r\n" -> [w1927]
                tunnel: "COUNTER_X_TEST=\nCOUNTER_PRECHARGE_COMPLETE=\nCOUNTER_CHARGE_COMPLETE=\nCOUNTER_STORAGE_MODE=\nCOUNTER_RUNTIME_SECS_PROG_1=\nCOUNTER_RUNTIME_SECS_PROG_2=\nCOUNTER_RUNTIME_SECS_PROG_3=\nCOUNTER_RUNTIME_SECS_PROG_4=\nCOUNTER_RUNTIME_SECS_PROG_5=\nCOUNTER_RUNTIME_SECS_PROG_6=\nCOUNTER_RUNTIME_SECS_PROG_7=\nCOUNTER_RUNTIME_SECS_PROG_8=\nCOUNTER_RUNTIME_SECS_PROG_9=\nCOUNTER_RUNTIME_SECS_PROG_10=\nCOUNTER_BATTERY_DEPLETION=\nCOUNTER_EVENT_QUEUE_MAX=" -> [w1925]
                i -> [w1924]
                n846 = Increment(x=w1924) -> (x+1=w1917:i32)
                n847 = Pick Line(multi-line string=w1925, line index=w1917) -> (output string=w1923:string)  [unwired: 1 in]
                n848 = Number To Decimal String(number=w1917) -> (decimal integer string=w1928:string)  [unwired: 1 in]
                n849 = Concatenate Strings("Counter=" ("Parameters"), w1928) -> (w1929:string)
                n850 = Bundle(cluster=w1938, "Command"=Typedef_Command_List."Get Counter", "MICS_ID"=w1932, "Parameters"=w1929) -> (w1935:T21)  [unwired: 5 in]
                n851 = call "Zarlink Telemetry.vi"("error in (no error)"=w1937, "Input"=w1935, "MICS Dongle Address"=w1931) -> ("error out"=w1936:errorcluster, "Output"=w1934:T28)  [unwired: 6 in, 1 out]
                n852 = Unbundle(w1934) -> ("Response Token"=w1920:string, "Response Code"=w1919:string, "Data"=w1915:string)  [unwired: 3 out]
                n853 = Match Pattern(string=w1915, regular expression="eventCount=") -> (after substring=w1914:string)  [unwired: 1 in, 3 out]
                n854 = Concatenate Strings(w1920, " - ", w1919) -> (w1918:string)
                n855 = local write "Response"(w1918) -> ()
                n856 = Concatenate Strings(w1927, "\r\n", w1923, w1914) -> (w1926:string)
              }
              "Event Counters Data" <- w1903
            }
            frame 12 {
              n857 = while {
                tunnel: w1947 -> [w1968]
                tunnel: w1944 -> [w1962]
                tunnel: w1943 -> [w1961]
                shift-right: [w1966] -> w1945
                shift-left: w1946 -> [w1967]
                tunnel: w1942 -> [w1957]
                tunnel: "CPDataTabs" -> [w1952]
                tunnel: [w1950] -> w1940
                tunnel: [w1949] -> w1939
                i -> [w1953]
                stop <- w1956 stop-if-true
                n858 = Select(t=w1952, s=w1957, f=w1953) -> (s? t:f=w1955:u32)
                n859 = Greater?(x=w1953, y=6) -> (0:w1959:bool)
                n860 = case shown="0, Default" w1955 {
                  tunnel: [Typedef_Command_List."Get CP Data" ("Command") Typedef_Command_List."Get CP Data" ("Command") Typedef_Command_List."Get CP Data" ("Command") Typedef_Command_List."Get CP Data" ("Command") Typedef_Command_List."Get CP Data" ("Command") Typedef_Command_List."Get CP Data" ("Command") Typedef_Command_List."Get CP Data" ("Command") Typedef_Command_List."Get CP Data" ("Command")] -> w1963
                  tunnel: ["List=0" ("Parameters") "List=1" ("Parameters") "List=2" ("Parameters") "List=3" ("Parameters") "List=4" ("Parameters") "List=5" ("Parameters") "List=6" ("Parameters") "List=7" ("Parameters")] -> w1958
                  frame 0, Default {
                  }
                  frame 1 {
                  }
                  frame 2 {
                  }
                  frame 3 {
                  }
                  frame 4 {
                  }
                  frame 5 {
                  }
                  frame 6 {
                  }
                  frame 7 {
                  }
                }
                n861 = Or(x=w1959, y=w1957) -> (x .or. y?=w1956:bool)
                n862 = Bundle(cluster=w1968, "Command"=w1963, "MICS_ID"=w1962, "Parameters"=w1958) -> (w1965:T21)  [unwired: 5 in]
                n863 = call "Zarlink Telemetry.vi"("error in (no error)"=w1967, "Input"=w1965, "MICS Dongle Address"=w1961) -> ("error out"=w1966:errorcluster, "Output"=w1964:T28)  [unwired: 6 in, 1 out]
                n864 = Unbundle(w1964) -> ("Response Token"=w1949:string, "Response Code"=w1950:string, "Data"=w1954:string)  [unwired: 3 out]
                n865 = case shown="0, Default" w1955 {
                  tunnel: w1954 -> [w1969 w1970 w1971 w1972 w1973 w1974 w1975 w1976]
                  frame 0, Default {
                    "CP Data 0" <- w1969
                  }
                  frame 1 {
                    "CP Data 1" <- w1970
                  }
                  frame 2 {
                    "CP Data 2" <- w1971
                  }
                  frame 3 {
                    "CP Data 3" <- w1972
                  }
                  frame 4 {
                    "CP Data 4" <- w1973
                  }
                  frame 5 {
                    "CP Data 5" <- w1974
                  }
                  frame 6 {
                    "CP Data 6" <- w1975
                  }
                  frame 7 {
                    "CP Data 7" <- w1976
                  }
                }
                n866 = Concatenate Strings(w1949, " - ", w1950) -> (w1948:string)
                n867 = local write "Response"(w1948) -> ()
              }
            }
            frame 13 {
              n868 = while {
                tunnel: w2002 -> [w2023]
                tunnel: w1999 -> [w2018]
                tunnel: w1998 -> [w2017]
                shift-right: [w2021] -> w2000
                shift-left: w2001 -> [w2022]
                tunnel: w1997 -> [w2013]
                tunnel: "ProgramData" -> [w2008]
                tunnel: [w2004] -> w1995
                tunnel: [w2003] -> w1994
                i -> [w2009]
                stop <- w2012 stop-if-true
                n869 = Select(t=w2008, s=w2013, f=w2009) -> (s? t:f=w2011:u32)
                n870 = Greater?(x=w2009, y=8) -> (0:w2015:bool)
                n871 = case shown="9" w2011 {
                  tunnel: ["List=1" ("Parameters") "List=2" ("Parameters") "List=3" ("Parameters") "List=4" ("Parameters") "List=5" ("Parameters") "List=6" ("Parameters") "List=7" ("Parameters") "List=8" ("Parameters") "List=9" ("Parameters") "List=10" ("Parameters")] -> w2014
                  frame 0, Default {
                  }
                  frame 1 {
                  }
                  frame 2 {
                  }
                  frame 3 {
                  }
                  frame 4 {
                  }
                  frame 5 {
                  }
                  frame 6 {
                  }
                  frame 7 {
                  }
                  frame 8 {
                  }
                  frame 9 {
                  }
                }
                n872 = Or(x=w2015, y=w2013) -> (x .or. y?=w2012:bool)
                n873 = Bundle(cluster=w2023, "Command"=Typedef_Command_List."Get Program Definition", "MICS_ID"=w2018, "Parameters"=w2014) -> (w2020:T21)  [unwired: 5 in]
                n874 = call "Zarlink Telemetry.vi"("error in (no error)"=w2022, "Input"=w2020, "MICS Dongle Address"=w2017) -> ("error out"=w2021:errorcluster, "Output"=w2019:T28)  [unwired: 6 in, 1 out]
                n875 = Unbundle(w2019) -> ("Response Token"=w2003:string, "Response Code"=w2004:string, "Data"=w2010:string)  [unwired: 3 out]
                n876 = case shown="9" w2011 {
                  tunnel: w2010 -> [w2024 w2025 w2026 w2027 w2028 w2029 w2030 w2031 w2032 w2033]
                  frame 0, Default {
                    "Program Data 1" <- w2024
                  }
                  frame 1 {
                    "Program Data 2" <- w2025
                  }
                  frame 2 {
                    "Program Data 3" <- w2026
                  }
                  frame 3 {
                    "Program Data 4" <- w2027
                  }
                  frame 4 {
                    "Program Data 5" <- w2028
                  }
                  frame 5 {
                    "Program Data 6" <- w2029
                  }
                  frame 6 {
                    "Program Data 7" <- w2030
                  }
                  frame 7 {
                    "Program Data 8" <- w2031
                  }
                  frame 8 {
                    "Program Data 9" <- w2032
                  }
                  frame 9 {
                    "Program Data 10" <- w2033
                  }
                }
                n877 = Concatenate Strings(w2003, " - ", w2004) -> (w2005:string)
                n878 = local write "Response"(w2005) -> ()
              }
              n879 = local write "ConstGetAll"(FALSE ("ConstGetAll")) -> ()
            }
          }
          n880 = Or(x=w1621, y=w1620) -> (x .or. y?=w1627:bool)
          n881 = Concatenate Strings(w1616, " - ", w1615) -> (w1614:string)
          n882 = local write "Response"(w1614) -> ()
          n883 = call <vilib>:"Unset Busy.vi"("error in (no error)"=w1610) -> ("error out"=w1611:errorcluster)  [unwired: 10 in]
        }
      }
      frame "Set Device Data" {
        (unwired) u8[] [] ("CP_DATA IN")
        n884 = local read "DevDataTabs"() -> (w2044:T14)
        n885 = local read "SESSION CONTROL"() -> (w2051:T3)
        n886 = Unbundle By Name(w2051) -> ("TARGET MICS ID"=w2050:u32)
        n887 = Not(x="ConstSetAll") -> (.not. x?=w2046:bool)
        n888 = while {
          tunnel: w2046 -> [w2066]
          tunnel: w2044 -> [w2065]
          tunnel: w2050 -> [w2070]
          shift-right: [w2057] -> w2052
          shift-left: w2053 -> [w2059]
          tunnel: w2049 -> [w2069]
          tunnel: [w2069] -> w2048
          tunnel: 12 ("y") -> [w2068]
          i -> [w2064]
          stop <- w2073 stop-if-true
          n889 = Greater?(x=w2064, y=w2068) -> (0:w2067:bool)
          n890 = call <vilib>:"Set Busy.vi"("error in (no error)"=w2059) -> ("error out"=w2058:errorcluster)  [unwired: 9 in, 1 out]
          n891 = Select(t=w2065, s=w2066, f=w2064) -> (s? t:f=w2072:u32)
          n892 = case shown="8" w2072 {
            selector: w2072 -> [_ _ _ _ _ w2126 w2163 _ _ w2220 _]
            tunnel: w2058 -> [w2083 w2094 w2104 w2114 w2124 w2133 w2170 w2208 w2218 w2227 w2273]
            tunnel: [w2082 w2093 w2103 w2113 w2123 w2132 w2169 w2207 w2217 w2226 w2272] -> w2056
            tunnel: T21 {"Command"=enum."Get xPG Status", "Function"=enum."Transceive (DN -> UP)", "MICS_ID"=0, "EXID"=16773121, "Use Local"=FALSE, "Transceive Delay mS"=200.0, "CP_DATA IN"=[], "Parameters"=""} ("Input") -> [w2084 w2095 w2105 w2115 w2125 w2134 w2171 w2209 w2219 w2228 w2274]
            tunnel: w2070 -> [w2078 w2089 w2099 w2109 w2119 w2131 w2168 w2203 w2213 w2225 w2271]
            tunnel: w2069 -> [w2077 w2088 w2098 w2108 w2118 w2130 w2167 w2202 w2212 w2224 w2270]
            tunnel: w2066 -> [_ _ _ _ _ w2129 w2166 _ _ w2223 w2269]
            tunnel: [w2075 w2086 w2096 w2106 w2116 w2127 w2164 w2200 w2210 w2221 w2267] -> w2062
            tunnel: [w2076 w2087 w2097 w2107 w2117 w2128 w2165 w2201 w2211 w2222 w2268] -> w2061
            frame 2 {
              n893 = local read "xPG Identity Data"() -> (w2074:string)
              n894 = Bundle(cluster=w2084, "Command"=Typedef_Command_List."Set xPG Identity", "MICS_ID"=w2078, "Parameters"=w2074) -> (w2081:T21)  [unwired: 5 in]
              n895 = call "Zarlink Telemetry.vi"("error in (no error)"=w2083, "Input"=w2081, "MICS Dongle Address"=w2077) -> ("error out"=w2082:errorcluster, "Output"=w2080:T28)  [unwired: 6 in, 1 out]
              n896 = Unbundle(w2080) -> ("Response Token"=w2075:string, "Response Code"=w2076:string)  [unwired: 4 out]
            }
            frame 3 {
              n897 = local read "General Calibration Data"() -> (w2085:string)
              n898 = Bundle(cluster=w2095, "Command"=Typedef_Command_List."Set General Calibration", "MICS_ID"=w2089, "Parameters"=w2085) -> (w2092:T21)  [unwired: 5 in]
              n899 = call "Zarlink Telemetry.vi"("error in (no error)"=w2094, "Input"=w2092, "MICS Dongle Address"=w2088) -> ("error out"=w2093:errorcluster, "Output"=w2091:T28)  [unwired: 6 in, 1 out]
              n900 = Unbundle(w2091) -> ("Response Token"=w2086:string, "Response Code"=w2087:string)  [unwired: 4 out]
            }
            frame 4, Default {
              n901 = Bundle(cluster=w2105, "Command"=Typedef_Command_List."Get Pulse Constants", "MICS_ID"=w2099) -> (w2102:T21)  [unwired: 6 in]
              n902 = call "Zarlink Telemetry.vi"("error in (no error)"=w2104, "Input"=w2102, "MICS Dongle Address"=w2098) -> ("error out"=w2103:errorcluster, "Output"=w2101:T28)  [unwired: 6 in, 1 out]
              n903 = Unbundle(w2101) -> ("Response Token"=w2096:string, "Response Code"=w2097:string)  [unwired: 4 out]
            }
            frame 5 {
              n904 = Bundle(cluster=w2115, "Command"=Typedef_Command_List."Get Program Constants", "MICS_ID"=w2109) -> (w2112:T21)  [unwired: 6 in]
              n905 = call "Zarlink Telemetry.vi"("error in (no error)"=w2114, "Input"=w2112, "MICS Dongle Address"=w2108) -> ("error out"=w2113:errorcluster, "Output"=w2111:T28)  [unwired: 6 in, 1 out]
              n906 = Unbundle(w2111) -> ("Response Token"=w2106:string, "Response Code"=w2107:string)  [unwired: 4 out]
            }
            frame 6 {
              n907 = Bundle(cluster=w2125, "Command"=Typedef_Command_List."Get Stim Asic HV Calibrations", "MICS_ID"=w2119) -> (w2122:T21)  [unwired: 6 in]
              n908 = call "Zarlink Telemetry.vi"("error in (no error)"=w2124, "Input"=w2122, "MICS Dongle Address"=w2118) -> ("error out"=w2123:errorcluster, "Output"=w2121:T28)  [unwired: 6 in, 1 out]
              n909 = Unbundle(w2121) -> ("Response Token"=w2116:string, "Response Code"=w2117:string)  [unwired: 4 out]
            }
            frame 7 {
              n910 = while {
                tunnel: w2134 -> [w2154]
                tunnel: w2131 -> [w2148]
                tunnel: w2130 -> [w2147]
                shift-right: [w2152] -> w2132
                shift-left: w2133 -> [w2153]
                tunnel: w2129 -> [w2143]
                tunnel: w2126 -> [w2139]
                tunnel: [w2136] -> w2128
                tunnel: [w2135] -> w2127
                i -> [w2140]
                stop <- w2142 stop-if-true
                n911 = Select(t=w2139, s=w2143, f=w2140) -> (s? t:f=w2141:u32)
                n912 = Greater?(x=w2140, y=2) -> (0:w2145:bool)
                n913 = case shown="0, Default" w2141 {
                  tunnel: [Typedef_Command_List."Get Channel Calibrations" ("Command") Typedef_Command_List."Get Channel Calibrations" ("Command") Typedef_Command_List."Get Channel Calibrations" ("Command") Typedef_Command_List."Get Channel Calibrations" ("Command")] -> w2149
                  tunnel: ["List=0" ("Parameters") "List=1" ("Parameters") "List=2" ("Parameters") "List=3" ("Parameters")] -> w2144
                  frame 0, Default {
                  }
                  frame 1 {
                  }
                  frame 2 {
                  }
                  frame 3 {
                  }
                }
                n914 = Or(x=w2145, y=w2143) -> (x .or. y?=w2142:bool)
                n915 = Bundle(cluster=w2154, "Command"=w2149, "MICS_ID"=w2148, "Parameters"=w2144) -> (w2151:T21)  [unwired: 5 in]
                n916 = call "Zarlink Telemetry.vi"("error in (no error)"=w2153, "Input"=w2151, "MICS Dongle Address"=w2147) -> ("error out"=w2152:errorcluster, "Output"=w2150:T28)  [unwired: 6 in, 1 out]
                n917 = Unbundle(w2150) -> ("Response Token"=w2135:string, "Response Code"=w2136:string)  [unwired: 4 out]
                n918 = Concatenate Strings(w2135, " - ", w2136) -> (w2137:string)
                n919 = local write "Response"(w2137) -> ()
              }
            }
            frame 8 {
              n920 = while {
                tunnel: w2171 -> [w2191]
                tunnel: w2168 -> [w2185]
                tunnel: w2167 -> [w2184]
                shift-right: [w2189] -> w2169
                shift-left: w2170 -> [w2190]
                tunnel: w2166 -> [w2180]
                tunnel: w2163 -> [w2176]
                tunnel: [w2173] -> w2165
                tunnel: [w2172] -> w2164
                i -> [w2177]
                stop <- w2179 stop-if-true
                n921 = Select(t=w2176, s=w2180, f=w2177) -> (s? t:f=w2178:u32)
                n922 = Greater?(x=w2177, y=2) -> (0:w2182:bool)
                n923 = case shown="0, Default" w2178 {
                  tunnel: [Typedef_Command_List."Get Trim List" ("Command") Typedef_Command_List."Get Trim List" ("Command") Typedef_Command_List."Get Trim List" ("Command") Typedef_Command_List."Get Trim List" ("Command")] -> w2186
                  tunnel: ["List=0" ("Parameters") "List=1" ("Parameters") "List=2" ("Parameters") "List=3" ("Parameters")] -> w2181
                  frame 0, Default {
                  }
                  frame 1 {
                  }
                  frame 2 {
                  }
                  frame 3 {
                  }
                }
                n924 = Or(x=w2182, y=w2180) -> (x .or. y?=w2179:bool)
                n925 = Bundle(cluster=w2191, "Command"=w2186, "MICS_ID"=w2185, "Parameters"=w2181) -> (w2188:T21)  [unwired: 5 in]
                n926 = call "Zarlink Telemetry.vi"("error in (no error)"=w2190, "Input"=w2188, "MICS Dongle Address"=w2184) -> ("error out"=w2189:errorcluster, "Output"=w2187:T28)  [unwired: 6 in, 1 out]
                n927 = Unbundle(w2187) -> ("Response Token"=w2172:string, "Response Code"=w2173:string)  [unwired: 4 out]
                n928 = Concatenate Strings(w2172, " - ", w2173) -> (w2174:string)
                n929 = local write "Response"(w2174) -> ()
              }
            }
            frame 9 {
              n930 = Bundle(cluster=w2209, "Command"=Typedef_Command_List."Get Lead Limits", "MICS_ID"=w2203) -> (w2206:T21)  [unwired: 6 in]
              n931 = call "Zarlink Telemetry.vi"("error in (no error)"=w2208, "Input"=w2206, "MICS Dongle Address"=w2202) -> ("error out"=w2207:errorcluster, "Output"=w2205:T28)  [unwired: 6 in, 1 out]
              n932 = Unbundle(w2205) -> ("Response Token"=w2200:string, "Response Code"=w2201:string)  [unwired: 4 out]
            }
            frame 10 {
              n933 = Bundle(cluster=w2219, "Command"=Typedef_Command_List."Get Configurable Device Parameters", "MICS_ID"=w2213) -> (w2216:T21)  [unwired: 6 in]
              n934 = call "Zarlink Telemetry.vi"("error in (no error)"=w2218, "Input"=w2216, "MICS Dongle Address"=w2212) -> ("error out"=w2217:errorcluster, "Output"=w2215:T28)  [unwired: 6 in, 1 out]
              n935 = Unbundle(w2215) -> ("Response Token"=w2210:string, "Response Code"=w2211:string)  [unwired: 4 out]
            }
            frame 12 {
              n936 = while {
                tunnel: w2228 -> [w2248]
                tunnel: w2225 -> [w2242]
                tunnel: w2224 -> [w2241]
                shift-right: [w2246] -> w2226
                shift-left: w2227 -> [w2247]
                tunnel: w2223 -> [w2237]
                tunnel: w2220 -> [w2233]
                tunnel: [w2231] -> w2222
                tunnel: [w2230] -> w2221
                i -> [w2234]
                stop <- w2236 stop-if-true
                n937 = Select(t=w2233, s=w2237, f=w2234) -> (s? t:f=w2235:u32)
                n938 = Greater?(x=w2234, y=6) -> (0:w2239:bool)
                n939 = case shown="0, Default" w2235 {
                  tunnel: [Typedef_Command_List."Get CP Data" ("Command") Typedef_Command_List."Get CP Data" ("Command") Typedef_Command_List."Get CP Data" ("Command") Typedef_Command_List."Get CP Data" ("Command") Typedef_Command_List."Get CP Data" ("Command") Typedef_Command_List."Get CP Data" ("Command") Typedef_Command_List."Get CP Data" ("Command") Typedef_Command_List."Get CP Data" ("Command")] -> w2243
                  tunnel: ["List=0" ("Parameters") "List=1" ("Parameters") "List=2" ("Parameters") "List=3" ("Parameters") "List=4" ("Parameters") "List=5" ("Parameters") "List=6" ("Parameters") "List=7" ("Parameters")] -> w2238
                  frame 0, Default {
                  }
                  frame 1 {
                  }
                  frame 2 {
                  }
                  frame 3 {
                  }
                  frame 4 {
                  }
                  frame 5 {
                  }
                  frame 6 {
                  }
                  frame 7 {
                  }
                }
                n940 = Or(x=w2239, y=w2237) -> (x .or. y?=w2236:bool)
                n941 = Bundle(cluster=w2248, "Command"=w2243, "MICS_ID"=w2242, "Parameters"=w2238) -> (w2245:T21)  [unwired: 5 in]
                n942 = call "Zarlink Telemetry.vi"("error in (no error)"=w2247, "Input"=w2245, "MICS Dongle Address"=w2241) -> ("error out"=w2246:errorcluster, "Output"=w2244:T28)  [unwired: 6 in, 1 out]
                n943 = Unbundle(w2244) -> ("Response Token"=w2230:string, "Response Code"=w2231:string)  [unwired: 4 out]
                n944 = Concatenate Strings(w2230, " - ", w2231) -> (w2229:string)
                n945 = local write "Response"(w2229) -> ()
              }
            }
            frame 13 {
              n946 = local read "ProgramData"() -> (w2265:T17)
              n947 = while {
                tunnel: w2274 -> [w2294]
                tunnel: w2271 -> [w2289]
                tunnel: w2270 -> [w2288]
                shift-right: [w2292] -> w2272
                shift-left: w2273 -> [w2293]
                tunnel: w2269 -> [w2284]
                tunnel: w2265 -> [w2280]
                tunnel: [w2276] -> w2268
                tunnel: [w2275] -> w2267
                i -> [w2281]
                stop <- w2283 stop-if-true
                n948 = Select(t=w2280, s=w2284, f=w2281) -> (s? t:f=w2282:u32)
                n949 = Greater?(x=w2281, y=8) -> (0:w2286:bool)
                n950 = case shown="9" w2282 {
                  tunnel: ["List=1" ("Parameters") "List=2" ("Parameters") "List=3" ("Parameters") "List=4" ("Parameters") "List=5" ("Parameters") "List=6" ("Parameters") "List=7" ("Parameters") "List=8" ("Parameters") "List=9" ("Parameters") "List=10" ("Parameters")] -> w2285
                  frame 0, Default {
                  }
                  frame 1 {
                  }
                  frame 2 {
                  }
                  frame 3 {
                  }
                  frame 4 {
                  }
                  frame 5 {
                  }
                  frame 6 {
                  }
                  frame 7 {
                  }
                  frame 8 {
                  }
                  frame 9 {
                  }
                }
                n951 = Or(x=w2286, y=w2284) -> (x .or. y?=w2283:bool)
                n952 = Bundle(cluster=w2294, "Command"=Typedef_Command_List."Get Program Definition", "MICS_ID"=w2289, "Parameters"=w2285) -> (w2291:T21)  [unwired: 5 in]
                n953 = call "Zarlink Telemetry.vi"("error in (no error)"=w2293, "Input"=w2291, "MICS Dongle Address"=w2288) -> ("error out"=w2292:errorcluster, "Output"=w2290:T28)  [unwired: 6 in, 1 out]
                n954 = Unbundle(w2290) -> ("Response Token"=w2275:string, "Response Code"=w2276:string)  [unwired: 4 out]
                n955 = Concatenate Strings(w2275, " - ", w2276) -> (w2277:string)
                n956 = local write "Response"(w2277) -> ()
              }
              n957 = local write "ConstSetAll"(FALSE ("ConstGetAll")) -> ()
            }
          }
          n958 = Or(x=w2067, y=w2066) -> (x .or. y?=w2073:bool)
          n959 = Concatenate Strings(w2062, " - ", w2061) -> (w2060:string)
          n960 = local write "Response"(w2060) -> ()
          n961 = call <vilib>:"Unset Busy.vi"("error in (no error)"=w2056) -> ("error out"=w2057:errorcluster)  [unwired: 10 in]
        }
      }
      frame "Clear Device Data" {
        w2305 = ""
        n962 = local write "Event Counters Data"(w2305) -> ()
        n963 = local write "Configurable Device Params"(w2305) -> ()
        n964 = local write "Channel Cals 0-3mA"(w2305) -> ()
        n965 = local write "Channel Cals 3-6mA"(w2305) -> ()
        n966 = local write "Channel Cals 6-9mA"(w2305) -> ()
        n967 = local write "Channel Cals 9-15mA"(w2305) -> ()
        n968 = local write "General Calibration Data"(w2305) -> ()
        n969 = local write "Program Constants Data"(w2305) -> ()
        n970 = local write "HV Calibrations Data"(w2305) -> ()
        n971 = local write "Pulse Constants Data"(w2305) -> ()
        n972 = local write "Lead Limits"(w2305) -> ()
        n973 = local write "Activity Log"(w2305) -> ()
        n974 = local write "xPG Identity Data"(w2305) -> ()
        n975 = local write "Error Log"(w2305) -> ()
        n976 = local write "Program Data 1"(w2305) -> ()
        n977 = local write "Program Data 2"(w2305) -> ()
        n978 = local write "Program Data 3"(w2305) -> ()
        n979 = local write "Program Data 4"(w2305) -> ()
        n980 = local write "Program Data 5"(w2305) -> ()
        n981 = local write "Program Data 6"(w2305) -> ()
        n982 = local write "Program Data 7"(w2305) -> ()
        n983 = local write "Program Data 8"(w2305) -> ()
        n984 = local write "Program Data 9"(w2305) -> ()
        n985 = local write "Program Data 10"(w2305) -> ()
        n986 = local write "Trim List 0"(w2305) -> ()
        n987 = local write "Trim List 1"(w2305) -> ()
        n988 = local write "Trim List 2"(w2305) -> ()
        n989 = local write "Trim List 3"(w2305) -> ()
        n990 = local write "CP Data 0"(w2305) -> ()
        n991 = local write "CP Data 1"(w2305) -> ()
        n992 = local write "CP Data 2"(w2305) -> ()
        n993 = local write "CP Data 3"(w2305) -> ()
        n994 = local write "CP Data 4"(w2305) -> ()
        n995 = local write "CP Data 5"(w2305) -> ()
        n996 = local write "CP Data 6"(w2305) -> ()
        n997 = local write "CP Data 7"(w2305) -> ()
      }
      frame "Save All Device Data" {
        n998 = Get Date/Time In Seconds() -> (seconds since 1Jan1904=w2311:timestamp)
        n999 = Get Date/Time String(seconds (now)=w2311) -> (date string=w2315:string, time string=w2314:string)  [unwired: 2 in]
        n1000 = Concatenate Strings(w2315, " - ", w2314) -> (w2312:string)
        n1001 = for {
          N: 5 -> [_]
          shift-right: [w2325] -> _
          shift-left: "" -> [w2326]
          shift-right: [w2323] -> w2316
          shift-left: w2318 -> [w2324]
          tunnel: w2312 -> [w2322]
          i -> [w2327]
          n1002 = case shown="4" w2327 {
            tunnel: w2326 -> [w2340 w2353 w2368 w2383 w2385]
            tunnel: [w2339 w2352 w2367 w2382 w2385] -> w2325
            tunnel: w2324 -> [w2338 w2351 w2366 w2381 w2387]
            tunnel: [w2337 w2350 w2365 w2380 w2386] -> w2323
            tunnel: w2322 -> [w2328 _ _ _ _]
            frame 0, Default {
              n1003 = local read "Configurable Device Params"() -> (w2335:string)
              n1004 = local read "General Calibration Data"() -> (w2336:string)
              n1005 = local read "Program Constants Data"() -> (w2332:string)
              n1006 = local read "Pulse Constants Data"() -> (w2333:string)
              n1007 = local read "Event Counters Data"() -> (w2334:string)
              n1008 = local read "HV Calibrations Data"() -> (w2331:string)
              n1009 = local read "xPG Identity Data"() -> (w2329:string)
              n1010 = local read "Lead Limits"() -> (w2330:string)
              n1011 = Format Into String(format string="[Full_Device_Save]\r\n\r\nAlgoStim Telemetry Tool\r\nSave Date: %s\r\n\r\n[xPG_Identity_Info]\r\n\r\n%s\r\n\r\n[General_Calibration_Data]\r\n\r\n%s\r\n\r\n[Configurable_Device_Parameters_Data]\r\n\r\n%s\r\n\r\n[Event_Counters_Data]\r\n\r\n%s\r\n\r\n[Pulse_Constants_Data]\r\n\r\n%s\r\n\r\n[Program_Constants_Data]\r\n\r\n%s\r\n\r\n[HV_Calibration_Data]\r\n\r\n%s\r\n\r\n[Lead_Limits_Data]\r\n\r\n%s\r\n\r\n", initial string=w2340, error in=w2338, w2328, w2329, w2336, w2335, w2334, w2333, w2332, w2331, w2330) -> (resulting string=w2339:string, error out=w2337:errorcluster)
            }
            frame 1 {
              n1012 = local read "Channel Cals 9-15mA"() -> (w2346:string)
              n1013 = local read "Channel Cals 0-3mA"() -> (w2349:string)
              n1014 = local read "Channel Cals 3-6mA"() -> (w2348:string)
              n1015 = local read "Channel Cals 6-9mA"() -> (w2347:string)
              n1016 = local read "Trim List 0"() -> (w2345:string)
              n1017 = local read "Trim List 1"() -> (w2344:string)
              n1018 = local read "Trim List 2"() -> (w2343:string)
              n1019 = local read "Trim List 3"() -> (w2342:string)
              n1020 = Format Into String(format string="[Channel_Calibration_Data_0-3mA]\r\n\r\n%s\r\n\r\n[Channel_Calibration_Data_3-6mA]\r\n\r\n%s\r\n\r\n[Channel_Calibration_Data_6-9mA]\r\n\r\n%s\r\n\r\n[Channel_Calibration_Data_9-15mA]\r\n\r\n%s\r\n\r\n[Trim_List_Data_0]\r\n\r\n%s\r\n\r\n[Trim_List_Data_1]\r\n\r\n%s\r\n\r\n[Trim_List_Data_2]\r\n\r\n%s\r\n\r\n[Trim_List_Data_3]\r\n\r\n%s\r\n\r\n", initial string=w2353, error in=w2351, w2349, w2348, w2347, w2346, w2345, w2344, w2343, w2342) -> (resulting string=w2352:string, error out=w2350:errorcluster)
            }
            frame 2 {
              n1021 = local read "Program Data 10"() -> (w2355:string)
              n1022 = local read "Program Data 1"() -> (w2364:string)
              n1023 = local read "Program Data 2"() -> (w2363:string)
              n1024 = local read "Program Data 3"() -> (w2362:string)
              n1025 = local read "Program Data 4"() -> (w2361:string)
              n1026 = local read "Program Data 5"() -> (w2360:string)
              n1027 = local read "Program Data 6"() -> (w2359:string)
              n1028 = local read "Program Data 7"() -> (w2358:string)
              n1029 = local read "Program Data 8"() -> (w2357:string)
              n1030 = local read "Program Data 9"() -> (w2356:string)
              n1031 = Format Into String(format string="[Patient_Program_Data_1]\r\n\r\n%s\r\n\r\n[Patient_Program_Data_2]\r\n\r\n%s\r\n\r\n[Patient_Program_Data_3]\r\n\r\n%s\r\n\r\n[Patient_Program_Data_4]\r\n\r\n%s\r\n\r\n[Patient_Program_Data_5]\r\n\r\n%s\r\n\r\n[Patient_Program_Data_6]\r\n\r\n%s\r\n\r\n[Patient_Program_Data_7]\r\n\r\n%s\r\n\r\n[Patient_Program_Data_8]\r\n\r\n%s\r\n\r\n[Patient_Program_Data_9]\r\n\r\n%s\r\n\r\n[Patient_Program_Data_10]\r\n\r\n%s\r\n\r\n", initial string=w2368, error in=w2366, w2364, w2363, w2362, w2361, w2360, w2359, w2358, w2357, w2356, w2355) -> (resulting string=w2367:string, error out=w2365:errorcluster)
            }
            frame 3 {
              n1032 = local read "Activity Log"() -> (w2371:string)
              n1033 = local read "CP Data 0"() -> (w2379:string)
              n1034 = local read "CP Data 1"() -> (w2378:string)
              n1035 = local read "CP Data 2"() -> (w2377:string)
              n1036 = local read "CP Data 3"() -> (w2376:string)
              n1037 = local read "CP Data 4"() -> (w2375:string)
              n1038 = local read "CP Data 5"() -> (w2374:string)
              n1039 = local read "CP Data 6"() -> (w2373:string)
              n1040 = local read "CP Data 7"() -> (w2372:string)
              n1041 = local read "Error Log"() -> (w2370:string)
              n1042 = Format Into String(format string="[CP_Data_0]\r\n\r\n%s\r\n\r\n[CP_Data_1]\r\n\r\n%s\r\n\r\n[CP_Data_2]\r\n\r\n%s\r\n\r\n[CP_Data_3]\r\n\r\n%s\r\n\r\n[CP_Data_4]\r\n\r\n%s\r\n\r\n[CP_Data_5]\r\n\r\n%s\r\n\r\n[CP_Data_6]\r\n\r\n%s\r\n\r\n[CP_Data_7]\r\n\r\n%s\r\n\r\n[Activity_Log]\r\n\r\n%s\r\n\r\n[Error_Log]\r\n\r\n%s\r\n\r\n[*** END OF FILE ***]\r\n\r\n", initial string=w2383, error in=w2381, w2379, w2378, w2377, w2376, w2375, w2374, w2373, w2372, w2371, w2370) -> (resulting string=w2382:string, error out=w2380:errorcluster)
            }
            frame 4 {
              n1043 = Open/Create/Replace File(error in=w2387, prompt="Save \"All Device Data\"", operation (0:open)=T26."replace or create with confirmation", access (0:read/write)=enum16{"read/write", "read-only", "write-only"}."write-only") -> (refnum out=w2390:refnum<file>, cancelled=w2389:bool, error out=w2391:errorcluster)  [unwired: 2 in]
              n1044 = case shown="False" w2389 {
                tunnel: w2391 -> [w2399 w2404]
                tunnel: w2390 -> [w2398 _]
                tunnel: w2385 -> [w2395 _]
                tunnel: [w2394 w2404] -> w2386
                frame False {
                  n1045 = Write to Text File(file (use dialog)=w2398, text=w2395, error in=w2399) -> (refnum out=w2396:refnum<file>, error out=w2397:errorcluster)  [unwired: 1 in, 1 out]
                  n1046 = case shown="No Error" w2397 {
                    selector: w2397 -> [w2402 w2403]
                    tunnel: w2396 -> [w2401 _]
                    tunnel: [w2400 w2403] -> w2394
                    frame No Error {
                      n1047 = Close File(refnum=w2401, error in=w2402) -> (error out=w2400:errorcluster)  [unwired: 1 out]
                    }
                    frame Error {
                    }
                  }
                }
                frame True {
                }
              }
            }
          }
        }
      }
      frame "Load All Device Data" {
        n1048 = Read from Text File(prompt (Open existing file)="Select a \"Device Full Save\" File:", count=-1, error in=w2412) -> (refnum out=w2413:refnum<file>, text=w2406:string[], cancelled=w2410:bool, error out=w2414:errorcluster)  [unwired: 1 in]
        n1049 = case shown="No Error" w2414 {
          selector: w2414 -> [w2976 w2977]
          tunnel: w2413 -> [w2975 _]
          tunnel: [w2974 w2977] -> w2409
          frame No Error {
            n1050 = Close File(refnum=w2975, error in=w2976) -> (error out=w2974:errorcluster)  [unwired: 1 out]
          }
          frame Error {
          }
        }
        n1051 = Unbundle By Name(w2409) -> ("status"=w2408:bool)
        n1052 = Or(x=w2408, y=w2410) -> (x .or. y?=w2407:bool)
        n1053 = case shown="False" w2407 {
          tunnel: [w2426 w2973] -> w2415
          tunnel: w2406 -> [w2424 _]
          tunnel: w2409 -> [w2425 w2973]
          frame False {
            n1054 = for {
              shift-right: [w2434] -> w2426
              shift-left: w2425 -> [w2434]
              tunnel: w2424 -> [w2433] mode=indexing
              tunnel: w2424 -> [w2432]
              shift-right: [w2430] -> w2422
              shift-left: 0 ("x+1") -> [w2431]
              i -> [w2439]
              n1055 = Increment(x=w2439) -> (x+1=w2438:i32)
              n1056 = call <vilib>:"Trim Whitespace.vi"("string"=w2433) -> ("trimmed string"=w2435:string)  [unwired: 1 in]
              n1057 = Increment(x=w2438) -> (x+1=w2437:i32)
              n1058 = case shown="\"[Pulse_Constants_Data]\"" w2435 {
                tunnel: w2432 -> [_ w2448 w2463 w2479 w2496 w2512 w2527 w2544 w2560 w2576 w2591 w2607 w2623 w2640 w2656 w2671 w2687 w2703 w2720 w2736 w2752 w2767 w2782 w2799 w2815 w2831 w2847 w2864 w2879 w2895 w2910 w2928 w2945 w2961]
                tunnel: w2437 -> [_ w2446 w2461 w2477 w2493 w2510 w2525 w2542 w2558 w2574 w2589 w2605 w2622 w2638 w2654 w2669 w2685 w2701 w2718 w2734 w2750 w2765 w2780 w2797 w2813 w2829 w2845 w2862 w2877 w2893 w2909 w2926 w2943 w2959]
                tunnel: "" -> [_ w2447 w2462 w2478 w2494 w2511 w2526 w2543 w2559 w2575 w2590 w2606 w2624 w2639 w2655 w2670 w2686 w2702 w2719 w2735 w2751 w2766 w2781 w2798 w2814 w2830 w2846 w2863 w2878 w2894 w2911 w2927 w2944 w2960]
                tunnel: w2431 -> [w2440 w2442 w2458 w2474 w2490 w2506 w2522 w2538 w2554 w2570 w2586 w2602 w2618 w2634 w2650 w2666 w2682 w2698 w2714 w2730 w2746 w2762 w2778 w2794 w2810 w2826 w2842 w2858 w2874 w2890 w2906 w2923 w2940 w2957]
                tunnel: [w2440 w2443 w2459 w2475 w2491 w2507 w2523 w2539 w2555 w2571 w2587 w2603 w2619 w2635 w2651 w2667 w2683 w2699 w2715 w2731 w2747 w2763 w2779 w2795 w2811 w2827 w2843 w2859 w2875 w2891 w2907 w2924 w2941 w2958] -> w2430
                tunnel: "\r\n" -> [_ w2441 w2457 w2473 w2489 w2505 w2521 w2537 w2553 w2569 w2585 w2601 w2617 w2633 w2649 w2665 w2681 w2697 w2713 w2729 w2745 w2761 w2777 w2793 w2809 w2825 w2841 w2857 w2873 w2889 w2905 w2922 w2939 w2956]
                frame "0", "NO MATCH", Default {
                }
                frame "[xPG_Identity_Info]" {
                  n1059 = for {
                    N: 3 -> [_]
                    tunnel: w2446 -> [w2455]
                    shift-right: [w2451] -> w2445
                    shift-left: w2447 -> [w2452]
                    tunnel: w2448 -> [w2453]
                    tunnel: w2441 -> [w2449]
                    i -> [w2456]
                    n1060 = Add(x=w2456, y=w2455) -> (x+y=w2454:i32)
                    n1061 = Index Array(array=w2453, index=w2454) -> (element=w2450:string)
                    n1062 = Concatenate Strings(w2452, w2450, w2449) -> (w2451:string)
                  }
                  n1063 = local write "xPG Identity Data"(w2445) -> ()
                  n1064 = Increment(x=w2442) -> (x+1=w2443:i32)
                }
                frame "[General_Calibration_Data]" {
                  n1065 = for {
                    N: 55 -> [_]
                    tunnel: w2461 -> [w2471]
                    shift-right: [w2467] -> w2460
                    shift-left: w2462 -> [w2468]
                    tunnel: w2463 -> [w2469]
                    tunnel: w2457 -> [w2465]
                    i -> [w2472]
                    n1066 = Add(x=w2472, y=w2471) -> (x+y=w2470:i32)
                    n1067 = Index Array(array=w2469, index=w2470) -> (element=w2466:string)
                    n1068 = Concatenate Strings(w2468, w2466, w2465) -> (w2467:string)
                  }
                  n1069 = local write "General Calibration Data"(w2460) -> ()
                  n1070 = Increment(x=w2458) -> (x+1=w2459:i32)
                }
                frame "[Configurable_Device_Parameters_Data]" {
                  n1071 = for {
                    N: 23 -> [_]
                    tunnel: w2477 -> [w2487]
                    shift-right: [w2483] -> w2476
                    shift-left: w2478 -> [w2484]
                    tunnel: w2479 -> [w2485]
                    tunnel: w2473 -> [w2481]
                    i -> [w2488]
                    n1072 = Add(x=w2488, y=w2487) -> (x+y=w2486:i32)
                    n1073 = Index Array(array=w2485, index=w2486) -> (element=w2482:string)
                    n1074 = Concatenate Strings(w2484, w2482, w2481) -> (w2483:string)
                  }
                  n1075 = local write "Configurable Device Params"(w2476) -> ()
                  n1076 = Increment(x=w2474) -> (x+1=w2475:i32)
                }
                frame "[Pulse_Constants_Data]" {
                  n1077 = for {
                    N: 17 -> [_]
                    tunnel: w2493 -> [w2503]
                    shift-right: [w2499] -> w2492
                    shift-left: w2494 -> [w2500]
                    tunnel: w2496 -> [w2501]
                    tunnel: w2489 -> [w2497]
                    i -> [w2504]
                    n1078 = Add(x=w2504, y=w2503) -> (x+y=w2502:i32)
                    n1079 = Index Array(array=w2501, index=w2502) -> (element=w2498:string)
                    n1080 = Concatenate Strings(w2500, w2498, w2497) -> (w2499:string)
                  }
                  n1081 = local write "Pulse Constants Data"(w2492) -> ()
                  n1082 = Increment(x=w2490) -> (x+1=w2491:i32)
                }
                frame "[Program_Constants_Data]" {
                  n1083 = for {
                    N: 64 -> [_]
                    tunnel: w2510 -> [w2519]
                    shift-right: [w2515] -> w2509
                    shift-left: w2511 -> [w2516]
                    tunnel: w2512 -> [w2517]
                    tunnel: w2505 -> [w2513]
                    i -> [w2520]
                    n1084 = Add(x=w2520, y=w2519) -> (x+y=w2518:i32)
                    n1085 = Index Array(array=w2517, index=w2518) -> (element=w2514:string)
                    n1086 = Concatenate Strings(w2516, w2514, w2513) -> (w2515:string)
                  }
                  n1087 = local write "Program Constants Data"(w2509) -> ()
                  n1088 = Increment(x=w2506) -> (x+1=w2507:i32)
                }
                frame "[HV_Calibration_Data]" {
                  n1089 = for {
                    N: 64 -> [_]
                    tunnel: w2525 -> [w2535]
                    shift-right: [w2531] -> w2524
                    shift-left: w2526 -> [w2532]
                    tunnel: w2527 -> [w2533]
                    tunnel: w2521 -> [w2529]
                    i -> [w2536]
                    n1090 = Add(x=w2536, y=w2535) -> (x+y=w2534:i32)
                    n1091 = Index Array(array=w2533, index=w2534) -> (element=w2530:string)
                    n1092 = Concatenate Strings(w2532, w2530, w2529) -> (w2531:string)
                  }
                  n1093 = local write "HV Calibrations Data"(w2524) -> ()
                  n1094 = Increment(x=w2522) -> (x+1=w2523:i32)
                }
                frame "[Lead_Limits_Data]" {
                  n1095 = for {
                    N: 52 -> [_]
                    tunnel: w2542 -> [w2551]
                    shift-right: [w2547] -> w2541
                    shift-left: w2543 -> [w2548]
                    tunnel: w2544 -> [w2549]
                    tunnel: w2537 -> [w2545]
                    i -> [w2552]
                    n1096 = Add(x=w2552, y=w2551) -> (x+y=w2550:i32)
                    n1097 = Index Array(array=w2549, index=w2550) -> (element=w2546:string)
                    n1098 = Concatenate Strings(w2548, w2546, w2545) -> (w2547:string)
                  }
                  n1099 = local write "Lead Limits"(w2541) -> ()
                  n1100 = Increment(x=w2538) -> (x+1=w2539:i32)
                }
                frame "[Channel_Calibration_Data_0-3mA]" {
                  n1101 = for {
                    N: 53 -> [_]
                    tunnel: w2558 -> [w2567]
                    shift-right: [w2563] -> w2557
                    shift-left: w2559 -> [w2564]
                    tunnel: w2560 -> [w2565]
                    tunnel: w2553 -> [w2561]
                    i -> [w2568]
                    n1102 = Add(x=w2568, y=w2567) -> (x+y=w2566:i32)
                    n1103 = Index Array(array=w2565, index=w2566) -> (element=w2562:string)
                    n1104 = Concatenate Strings(w2564, w2562, w2561) -> (w2563:string)
                  }
                  n1105 = local write "Channel Cals 0-3mA"(w2557) -> ()
                  n1106 = Increment(x=w2554) -> (x+1=w2555:i32)
                }
                frame "[Channel_Calibration_Data_3-6mA]" {
                  n1107 = for {
                    N: 53 -> [_]
                    tunnel: w2574 -> [w2583]
                    shift-right: [w2579] -> w2573
                    shift-left: w2575 -> [w2580]
                    tunnel: w2576 -> [w2581]
                    tunnel: w2569 -> [w2577]
                    i -> [w2584]
                    n1108 = Add(x=w2584, y=w2583) -> (x+y=w2582:i32)
                    n1109 = Index Array(array=w2581, index=w2582) -> (element=w2578:string)
                    n1110 = Concatenate Strings(w2580, w2578, w2577) -> (w2579:string)
                  }
                  n1111 = local write "Channel Cals 3-6mA"(w2573) -> ()
                  n1112 = Increment(x=w2570) -> (x+1=w2571:i32)
                }
                frame "[Channel_Calibration_Data_6-9mA]" {
                  n1113 = for {
                    N: 53 -> [_]
                    tunnel: w2589 -> [w2599]
                    shift-right: [w2595] -> w2592
                    shift-left: w2590 -> [w2596]
                    tunnel: w2591 -> [w2597]
                    tunnel: w2585 -> [w2593]
                    i -> [w2600]
                    n1114 = Add(x=w2600, y=w2599) -> (x+y=w2598:i32)
                    n1115 = Index Array(array=w2597, index=w2598) -> (element=w2594:string)
                    n1116 = Concatenate Strings(w2596, w2594, w2593) -> (w2595:string)
                  }
                  n1117 = local write "Channel Cals 6-9mA"(w2592) -> ()
                  n1118 = Increment(x=w2586) -> (x+1=w2587:i32)
                }
                frame "[Channel_Calibration_Data_9-15mA]" {
                  n1119 = for {
                    N: 53 -> [_]
                    tunnel: w2605 -> [w2615]
                    shift-right: [w2611] -> w2608
                    shift-left: w2606 -> [w2612]
                    tunnel: w2607 -> [w2613]
                    tunnel: w2601 -> [w2609]
                    i -> [w2616]
                    n1120 = Add(x=w2616, y=w2615) -> (x+y=w2614:i32)
                    n1121 = Index Array(array=w2613, index=w2614) -> (element=w2610:string)
                    n1122 = Concatenate Strings(w2612, w2610, w2609) -> (w2611:string)
                  }
                  n1123 = local write "Channel Cals 9-15mA"(w2608) -> ()
                  n1124 = Increment(x=w2602) -> (x+1=w2603:i32)
                }
                frame "[Patient_Program_Data_1]" {
                  n1125 = for {
                    N: 213 -> [_]
                    tunnel: w2622 -> [w2631]
                    shift-right: [w2627] -> w2621
                    shift-left: w2624 -> [w2628]
                    tunnel: w2623 -> [w2629]
                    tunnel: w2617 -> [w2625]
                    i -> [w2632]
                    n1126 = Add(x=w2632, y=w2631) -> (x+y=w2630:i32)
                    n1127 = Index Array(array=w2629, index=w2630) -> (element=w2626:string)
                    n1128 = Concatenate Strings(w2628, w2626, w2625) -> (w2627:string)
                  }
                  n1129 = local write "Program Data 1"(w2621) -> ()
                  n1130 = Increment(x=w2618) -> (x+1=w2619:i32)
                }
                frame "[Patient_Program_Data_2]" {
                  n1131 = for {
                    N: 213 -> [_]
                    tunnel: w2638 -> [w2647]
                    shift-right: [w2643] -> w2637
                    shift-left: w2639 -> [w2644]
                    tunnel: w2640 -> [w2645]
                    tunnel: w2633 -> [w2641]
                    i -> [w2648]
                    n1132 = Add(x=w2648, y=w2647) -> (x+y=w2646:i32)
                    n1133 = Index Array(array=w2645, index=w2646) -> (element=w2642:string)
                    n1134 = Concatenate Strings(w2644, w2642, w2641) -> (w2643:string)
                  }
                  n1135 = local write "Program Data 2"(w2637) -> ()
                  n1136 = Increment(x=w2634) -> (x+1=w2635:i32)
                }
                frame "[Patient_Program_Data_3]" {
                  n1137 = for {
                    N: 213 -> [_]
                    tunnel: w2654 -> [w2663]
                    shift-right: [w2659] -> w2653
                    shift-left: w2655 -> [w2660]
                    tunnel: w2656 -> [w2661]
                    tunnel: w2649 -> [w2657]
                    i -> [w2664]
                    n1138 = Add(x=w2664, y=w2663) -> (x+y=w2662:i32)
                    n1139 = Index Array(array=w2661, index=w2662) -> (element=w2658:string)
                    n1140 = Concatenate Strings(w2660, w2658, w2657) -> (w2659:string)
                  }
                  n1141 = local write "Program Data 3"(w2653) -> ()
                  n1142 = Increment(x=w2650) -> (x+1=w2651:i32)
                }
                frame "[Patient_Program_Data_4]" {
                  n1143 = for {
                    N: 213 -> [_]
                    shift-right: [w2676] -> w2672
                    shift-left: w2670 -> [w2677]
                    tunnel: w2671 -> [w2678]
                    tunnel: w2669 -> [w2674]
                    tunnel: w2665 -> [w2673]
                    i -> [w2680]
                    n1144 = Add(x=w2680, y=w2674) -> (x+y=w2679:i32)
                    n1145 = Index Array(array=w2678, index=w2679) -> (element=w2675:string)
                    n1146 = Concatenate Strings(w2677, w2675, w2673) -> (w2676:string)
                  }
                  n1147 = local write "Program Data 4"(w2672) -> ()
                  n1148 = Increment(x=w2666) -> (x+1=w2667:i32)
                }
                frame "[Patient_Program_Data_5]" {
                  n1149 = for {
                    N: 213 -> [_]
                    shift-right: [w2692] -> w2688
                    shift-left: w2686 -> [w2693]
                    tunnel: w2687 -> [w2694]
                    tunnel: w2685 -> [w2690]
                    tunnel: w2681 -> [w2689]
                    i -> [w2696]
                    n1150 = Add(x=w2696, y=w2690) -> (x+y=w2695:i32)
                    n1151 = Index Array(array=w2694, index=w2695) -> (element=w2691:string)
                    n1152 = Concatenate Strings(w2693, w2691, w2689) -> (w2692:string)
                  }
                  n1153 = local write "Program Data 5"(w2688) -> ()
                  n1154 = Increment(x=w2682) -> (x+1=w2683:i32)
                }
                frame "[Patient_Program_Data_6]" {
                  n1155 = for {
                    N: 213 -> [_]
                    tunnel: w2701 -> [w2711]
                    shift-right: [w2707] -> w2704
                    shift-left: w2702 -> [w2708]
                    tunnel: w2703 -> [w2709]
                    tunnel: w2697 -> [w2705]
                    i -> [w2712]
                    n1156 = Add(x=w2712, y=w2711) -> (x+y=w2710:i32)
                    n1157 = Index Array(array=w2709, index=w2710) -> (element=w2706:string)
                    n1158 = Concatenate Strings(w2708, w2706, w2705) -> (w2707:string)
                  }
                  n1159 = local write "Program Data 6"(w2704) -> ()
                  n1160 = Increment(x=w2698) -> (x+1=w2699:i32)
                }
                frame "[Patient_Program_Data_7]" {
                  n1161 = for {
                    N: 213 -> [_]
                    tunnel: w2718 -> [w2727]
                    shift-right: [w2723] -> w2717
                    shift-left: w2719 -> [w2724]
                    tunnel: w2720 -> [w2725]
                    tunnel: w2713 -> [w2721]
                    i -> [w2728]
                    n1162 = Add(x=w2728, y=w2727) -> (x+y=w2726:i32)
                    n1163 = Index Array(array=w2725, index=w2726) -> (element=w2722:string)
                    n1164 = Concatenate Strings(w2724, w2722, w2721) -> (w2723:string)
                  }
                  n1165 = local write "Program Data 7"(w2717) -> ()
                  n1166 = Increment(x=w2714) -> (x+1=w2715:i32)
                }
                frame "[Patient_Program_Data_8]" {
                  n1167 = for {
                    N: 213 -> [_]
                    tunnel: w2734 -> [w2743]
                    shift-right: [w2739] -> w2733
                    shift-left: w2735 -> [w2740]
                    tunnel: w2736 -> [w2741]
                    tunnel: w2729 -> [w2737]
                    i -> [w2744]
                    n1168 = Add(x=w2744, y=w2743) -> (x+y=w2742:i32)
                    n1169 = Index Array(array=w2741, index=w2742) -> (element=w2738:string)
                    n1170 = Concatenate Strings(w2740, w2738, w2737) -> (w2739:string)
                  }
                  n1171 = local write "Program Data 8"(w2733) -> ()
                  n1172 = Increment(x=w2730) -> (x+1=w2731:i32)
                }
                frame "[Patient_Program_Data_9]" {
                  n1173 = for {
                    N: 213 -> [_]
                    tunnel: w2750 -> [w2759]
                    shift-right: [w2755] -> w2749
                    shift-left: w2751 -> [w2756]
                    tunnel: w2752 -> [w2757]
                    tunnel: w2745 -> [w2753]
                    i -> [w2760]
                    n1174 = Add(x=w2760, y=w2759) -> (x+y=w2758:i32)
                    n1175 = Index Array(array=w2757, index=w2758) -> (element=w2754:string)
                    n1176 = Concatenate Strings(w2756, w2754, w2753) -> (w2755:string)
                  }
                  n1177 = local write "Program Data 9"(w2749) -> ()
                  n1178 = Increment(x=w2746) -> (x+1=w2747:i32)
                }
                frame "[Patient_Program_Data_10]" {
                  n1179 = for {
                    N: 213 -> [_]
                    tunnel: w2765 -> [w2775]
                    shift-right: [w2771] -> w2764
                    shift-left: w2766 -> [w2772]
                    tunnel: w2767 -> [w2773]
                    tunnel: w2761 -> [w2769]
                    i -> [w2776]
                    n1180 = Add(x=w2776, y=w2775) -> (x+y=w2774:i32)
                    n1181 = Index Array(array=w2773, index=w2774) -> (element=w2770:string)
                    n1182 = Concatenate Strings(w2772, w2770, w2769) -> (w2771:string)
                  }
                  n1183 = local write "Program Data 10"(w2764) -> ()
                  n1184 = Increment(x=w2762) -> (x+1=w2763:i32)
                }
                frame "[CP_Data_0]" {
                  n1185 = for {
                    N: 257 -> [_]
                    tunnel: w2780 -> [w2791]
                    shift-right: [w2787] -> w2784
                    shift-left: w2781 -> [w2788]
                    tunnel: w2782 -> [w2789]
                    tunnel: w2777 -> [w2785]
                    i -> [w2792]
                    n1186 = Add(x=w2792, y=w2791) -> (x+y=w2790:i32)
                    n1187 = Index Array(array=w2789, index=w2790) -> (element=w2786:string)
                    n1188 = Concatenate Strings(w2788, w2786, w2785) -> (w2787:string)
                  }
                  n1189 = local write "CP Data 0"(w2784) -> ()
                  n1190 = Increment(x=w2778) -> (x+1=w2779:i32)
                }
                frame "[CP_Data_1]" {
                  n1191 = for {
                    N: 257 -> [_]
                    tunnel: w2797 -> [w2807]
                    shift-right: [w2803] -> w2796
                    shift-left: w2798 -> [w2804]
                    tunnel: w2799 -> [w2805]
                    tunnel: w2793 -> [w2801]
                    i -> [w2808]
                    n1192 = Add(x=w2808, y=w2807) -> (x+y=w2806:i32)
                    n1193 = Index Array(array=w2805, index=w2806) -> (element=w2802:string)
                    n1194 = Concatenate Strings(w2804, w2802, w2801) -> (w2803:string)
                  }
                  n1195 = local write "CP Data 1"(w2796) -> ()
                  n1196 = Increment(x=w2794) -> (x+1=w2795:i32)
                }
                frame "[CP_Data_2]" {
                  n1197 = for {
                    N: 257 -> [_]
                    tunnel: w2813 -> [w2823]
                    shift-right: [w2819] -> w2812
                    shift-left: w2814 -> [w2820]
                    tunnel: w2815 -> [w2821]
                    tunnel: w2809 -> [w2817]
                    i -> [w2824]
                    n1198 = Add(x=w2824, y=w2823) -> (x+y=w2822:i32)
                    n1199 = Index Array(array=w2821, index=w2822) -> (element=w2818:string)
                    n1200 = Concatenate Strings(w2820, w2818, w2817) -> (w2819:string)
                  }
                  n1201 = local write "CP Data 2"(w2812) -> ()
                  n1202 = Increment(x=w2810) -> (x+1=w2811:i32)
                }
                frame "[CP_Data_3]" {
                  n1203 = for {
                    N: 257 -> [_]
                    tunnel: w2829 -> [w2839]
                    shift-right: [w2835] -> w2828
                    shift-left: w2830 -> [w2836]
                    tunnel: w2831 -> [w2837]
                    tunnel: w2825 -> [w2833]
                    i -> [w2840]
                    n1204 = Add(x=w2840, y=w2839) -> (x+y=w2838:i32)
                    n1205 = Index Array(array=w2837, index=w2838) -> (element=w2834:string)
                    n1206 = Concatenate Strings(w2836, w2834, w2833) -> (w2835:string)
                  }
                  n1207 = local write "CP Data 3"(w2828) -> ()
                  n1208 = Increment(x=w2826) -> (x+1=w2827:i32)
                }
                frame "[CP_Data_4]" {
                  n1209 = for {
                    N: 257 -> [_]
                    tunnel: w2845 -> [w2855]
                    shift-right: [w2851] -> w2844
                    shift-left: w2846 -> [w2852]
                    tunnel: w2847 -> [w2853]
                    tunnel: w2841 -> [w2849]
                    i -> [w2856]
                    n1210 = Add(x=w2856, y=w2855) -> (x+y=w2854:i32)
                    n1211 = Index Array(array=w2853, index=w2854) -> (element=w2850:string)
                    n1212 = Concatenate Strings(w2852, w2850, w2849) -> (w2851:string)
                  }
                  n1213 = local write "CP Data 4"(w2844) -> ()
                  n1214 = Increment(x=w2842) -> (x+1=w2843:i32)
                }
                frame "[CP_Data_5]" {
                  n1215 = for {
                    N: 257 -> [_]
                    tunnel: w2862 -> [w2871]
                    shift-right: [w2867] -> w2861
                    shift-left: w2863 -> [w2868]
                    tunnel: w2864 -> [w2869]
                    tunnel: w2857 -> [w2865]
                    i -> [w2872]
                    n1216 = Add(x=w2872, y=w2871) -> (x+y=w2870:i32)
                    n1217 = Index Array(array=w2869, index=w2870) -> (element=w2866:string)
                    n1218 = Concatenate Strings(w2868, w2866, w2865) -> (w2867:string)
                  }
                  n1219 = local write "CP Data 5"(w2861) -> ()
                  n1220 = Increment(x=w2858) -> (x+1=w2859:i32)
                }
                frame "[CP_Data_6]" {
                  n1221 = for {
                    N: 257 -> [_]
                    tunnel: w2877 -> [w2887]
                    shift-right: [w2883] -> w2876
                    shift-left: w2878 -> [w2884]
                    tunnel: w2879 -> [w2885]
                    tunnel: w2873 -> [w2881]
                    i -> [w2888]
                    n1222 = Add(x=w2888, y=w2887) -> (x+y=w2886:i32)
                    n1223 = Index Array(array=w2885, index=w2886) -> (element=w2882:string)
                    n1224 = Concatenate Strings(w2884, w2882, w2881) -> (w2883:string)
                  }
                  n1225 = local write "CP Data 6"(w2876) -> ()
                  n1226 = Increment(x=w2874) -> (x+1=w2875:i32)
                }
                frame "[CP_Data_7]" {
                  n1227 = for {
                    N: 257 -> [_]
                    tunnel: w2893 -> [w2903]
                    shift-right: [w2900] -> w2896
                    shift-left: w2894 -> [w2901]
                    tunnel: w2895 -> [w2898]
                    tunnel: w2889 -> [w2897]
                    i -> [w2904]
                    n1228 = Add(x=w2904, y=w2903) -> (x+y=w2902:i32)
                    n1229 = Index Array(array=w2898, index=w2902) -> (element=w2899:string)
                    n1230 = Concatenate Strings(w2901, w2899, w2897) -> (w2900:string)
                  }
                  n1231 = local write "CP Data 7"(w2896) -> ()
                  n1232 = Increment(x=w2890) -> (x+1=w2891:i32)
                }
                frame "[Trim_List_Data_0]" {
                  n1233 = while {
                    tunnel: w2909 -> [w2914]
                    shift-right: [w2915] -> w2908
                    shift-left: w2911 -> [w2918]
                    tunnel: w2910 -> [w2917]
                    tunnel: w2905 -> [w2912]
                    i -> [w2916]
                    stop <- w2921 stop-if-true
                    n1234 = Add(x=w2916, y=w2914) -> (x+y=w2919:i32)
                    n1235 = Index Array(array=w2917, index=w2919) -> (element=w2913:string)
                    n1236 = Concatenate Strings(w2918, w2913, w2912) -> (w2915:string)
                    n1237 = call <vilib>:"Trim Whitespace.vi"("string"=w2913) -> ("trimmed string"=w2920:string)  [unwired: 1 in]
                    n1238 = Empty String/Path?(string/path=w2920) -> (empty?=w2921:bool)
                  }
                  n1239 = local write "Trim List 0"(w2908) -> ()
                  n1240 = Increment(x=w2906) -> (x+1=w2907:i32)
                }
                frame "[Trim_List_Data_1]" {
                  n1241 = while {
                    tunnel: w2926 -> [w2931]
                    shift-right: [w2932] -> w2925
                    shift-left: w2927 -> [w2935]
                    tunnel: w2928 -> [w2934]
                    tunnel: w2922 -> [w2929]
                    i -> [w2933]
                    stop <- w2938 stop-if-true
                    n1242 = Add(x=w2933, y=w2931) -> (x+y=w2936:i32)
                    n1243 = Index Array(array=w2934, index=w2936) -> (element=w2930:string)
                    n1244 = Concatenate Strings(w2935, w2930, w2929) -> (w2932:string)
                    n1245 = call <vilib>:"Trim Whitespace.vi"("string"=w2930) -> ("trimmed string"=w2937:string)  [unwired: 1 in]
                    n1246 = Empty String/Path?(string/path=w2937) -> (empty?=w2938:bool)
                  }
                  n1247 = local write "Trim List 1"(w2925) -> ()
                  n1248 = Increment(x=w2923) -> (x+1=w2924:i32)
                }
                frame "[Trim_List_Data_2]" {
                  n1249 = while {
                    tunnel: w2943 -> [w2948]
                    shift-right: [w2949] -> w2942
                    shift-left: w2944 -> [w2952]
                    tunnel: w2945 -> [w2951]
                    tunnel: w2939 -> [w2946]
                    i -> [w2950]
                    stop <- w2955 stop-if-true
                    n1250 = Add(x=w2950, y=w2948) -> (x+y=w2953:i32)
                    n1251 = Index Array(array=w2951, index=w2953) -> (element=w2947:string)
                    n1252 = Concatenate Strings(w2952, w2947, w2946) -> (w2949:string)
                    n1253 = call <vilib>:"Trim Whitespace.vi"("string"=w2947) -> ("trimmed string"=w2954:string)  [unwired: 1 in]
                    n1254 = Empty String/Path?(string/path=w2954) -> (empty?=w2955:bool)
                  }
                  n1255 = local write "Trim List 2"(w2942) -> ()
                  n1256 = Increment(x=w2940) -> (x+1=w2941:i32)
                }
                frame "[Trim_List_Data_3]" {
                  n1257 = while {
                    tunnel: w2959 -> [w2965]
                    shift-right: [w2966] -> w2962
                    shift-left: w2960 -> [w2969]
                    tunnel: w2961 -> [w2968]
                    tunnel: w2956 -> [w2963]
                    i -> [w2967]
                    stop <- w2972 stop-if-true
                    n1258 = Add(x=w2967, y=w2965) -> (x+y=w2970:i32)
                    n1259 = Index Array(array=w2968, index=w2970) -> (element=w2964:string)
                    n1260 = Concatenate Strings(w2969, w2964, w2963) -> (w2966:string)
                    n1261 = call <vilib>:"Trim Whitespace.vi"("string"=w2964) -> ("trimmed string"=w2971:string)  [unwired: 1 in]
                    n1262 = Empty String/Path?(string/path=w2971) -> (empty?=w2972:bool)
                  }
                  n1263 = local write "Trim List 3"(w2962) -> ()
                  n1264 = Increment(x=w2957) -> (x+1=w2958:i32)
                }
              }
            }
            n1265 = Equal?(x=w2422, y=33) -> (x = y?=w2420:bool)
            n1266 = case shown="False" w2420 {
              tunnel: ["The correct number of Full Device Save records were found and loaded." ("message") "The Loading Operation did not find the correct number of Full Device Save records!  Check for any missing data in the Device Data fields." ("message")] -> w2419
              frame True {
              }
              frame False {
              }
            }
            n1267 = One Button Dialog(message=w2419) -> ()  [unwired: 1 in, 1 out]
          }
          frame True {
          }
        }
      }
      frame "Build Pat Prog String" {
        n1268 = local read "PatStim"() -> (w2981:T10)
        n1269 = for {
          N: 5 -> [_]
          tunnel: w2981 -> [w2988]
          shift-right: [w2987] -> w2980
          shift-left: "" -> [w2986]
          i -> [w2989]
          n1270 = case shown="4" w2989 {
            tunnel: w2988 -> [w3027 w3038 w3060 w3082 w3104]
            tunnel: [w2997 w3041 w3063 w3085 w3107] -> w2987
            tunnel: w2986 -> [w2991 w3040 w3062 w3084 w3106]
            frame 0, Default {
              n1271 = Unbundle By Name(w3027) -> ("Program Number"=w3025:u8, "Program Defined"=w2994:bool, "Program Disabled"=w2995:bool, "Program Name"=w3024:string, "Allowed Freq Indexes"=w3023:u8[], "Default Freq Index"=w3013:u8, "PA.Defined"=w3012:bool, "PB.Defined"=w3011:bool, "PC.Defined"=w3010:bool, "PD.Defined"=w3009:bool)
              n1272 = local write "Patient Program String"(w2991) -> ()
              n1273 = Boolean To (0,1)(Boolean=w2994) -> (0, 1=w2993:i16)
              n1274 = Boolean To (0,1)(Boolean=w2995) -> (0, 1=w2992:i16)
              n1275 = Array To Cluster(array=w3023) -> (cluster=w3022:T29)
              n1276 = Boolean To (0,1)(Boolean=w3012) -> (0, 1=w2998:i16)
              n1277 = Boolean To (0,1)(Boolean=w3011) -> (0, 1=w3006:i16)
              n1278 = Boolean To (0,1)(Boolean=w3010) -> (0, 1=w3007:i16)
              n1279 = Boolean To (0,1)(Boolean=w3009) -> (0, 1=w3008:i16)
              n1280 = Logical Shift(y=i8 1, x=w3006) -> (x << y=w2999:i16)
              n1281 = Logical Shift(y=i8 2, x=w3007) -> (x << y=w3000:i16)
              n1282 = Logical Shift(y=i8 3, x=w3008) -> (x << y=w3001:i16)
              n1283 = Decrement(x=w3013) -> (x-1=w2990:u8)
              n1284 = Compound Arithmetic op=ADD(w2998, w2999, w3000, w3001) -> (w3002:i16)
              n1285 = To Unsigned Byte Integer(number=w3002) -> (unsigned 8bit integer=w2996:u8)
              n1286 = Unbundle(w3022) -> ("Allowed Freq Indexes[0]"=w3021:u8, "Allowed Freq Indexes[1]"=w3020:u8, "Allowed Freq Indexes[2]"=w3019:u8, "Allowed Freq Indexes[3]"=w3018:u8, "Allowed Freq Indexes[4]"=w3017:u8, "Allowed Freq Indexes[5]"=w3016:u8, "Allowed Freq Indexes[6]"=w3015:u8, "Allowed Freq Indexes[7]"=w3014:u8)
              n1287 = Format Into String(format string="ProgramNumber=%d\r\nProgramDefined=%d\r\nProgramDisabled=%d\r\nProgramName=%s\r\nAllowedFrequencies[0]=0x%02x\r\nAllowedFrequencies[1]=0x%02x\r\nAllowedFrequencies[2]=0x%02x\r\nAllowedFrequencies[3]=0x%02x\r\nAllowedFrequencies[4]=0x%02x\r\nAllowedFrequencies[5]=0x%02x\r\nAllowedFrequencies[6]=0x%02x\r\nAllowedFrequencies[7]=0x%02x\r\nProgramFrequencyIndex=%d\r\nDefinedPulseMap=0x%02x\r\n", w3025, w2993, w2992, w3024, w3021, w3020, w3019, w3018, w3017, w3016, w3015, w3014, w2990, w2996) -> (resulting string=w2997:string)  [unwired: 2 in, 1 out]
            }
            frame 1 {
              n1288 = Unbundle By Name(w3038) -> ("PA.Pulse Name"=w3037:string, "PA.Amp Low Limit (uA)"=w3036:u16, "PA.Amp Step (uA)"=w3035:u16, "PA.Amp Step Index"=w3034:u16, "PA.PW Low Limit (uS)"=w3033:u16, "PA.PW High Limit (uS)"=w3032:u16, "PA.PW Default (uS)"=w3031:u16, "PA.Amplitudes"=w3030:i8[])
              n1289 = for {
                tunnel: w3030 -> [w3049] mode=indexing
                shift-right: [w3047] -> w3029
                shift-left: "" -> [w3048]
                i -> [w3045]
                n1290 = To Byte Integer(number=w3049) -> (8bit integer=w3043:i8)
                n1291 = Increment(x=w3045) -> (x+1=w3044:i32)
                n1292 = Format Into String(format string="ElectrodeAmpPercentPA[CH%02d]=%d\\r\\n", initial string=w3048, w3044, w3043) -> (resulting string=w3047:string)  [unwired: 1 in, 1 out]
              }
              n1293 = Format Into String(format string="PulseNamePA=%s\r\nAmplitudeLowLimitPA=%d\r\nAmplitudeStepPA=%d\r\nAmplitudeStepIndexPA=%d\r\nPulseWidthLowLimitPA=%d\r\nPulseWidthHighLimitPA=%d\r\nPulseWidthPA=%d\r\n%s", w3037, w3036, w3035, w3034, w3033, w3032, w3031, w3029) -> (resulting string=w3039:string)  [unwired: 2 in, 1 out]
              n1294 = Concatenate Strings(w3040, w3039) -> (w3041:string)
            }
            frame 2 {
              n1295 = Unbundle By Name(w3060) -> ("PB.Pulse Name"=w3059:string, "PB.Amp Low Limit (uA)"=w3058:u16, "PB.Amp Step (uA)"=w3057:u16, "PB.Amp Step Index"=w3056:u16, "PB.PW Low Limit (uS)"=w3055:u16, "PB.PW High Limit (uS)"=w3054:u16, "PB.PW Default (uS)"=w3053:u16, "PB.Amplitudes"=w3052:i8[])
              n1296 = for {
                tunnel: w3052 -> [w3071] mode=indexing
                shift-right: [w3069] -> w3051
                shift-left: "" -> [w3070]
                i -> [w3067]
                n1297 = To Byte Integer(number=w3071) -> (8bit integer=w3065:i8)
                n1298 = Increment(x=w3067) -> (x+1=w3066:i32)
                n1299 = Format Into String(format string="ElectrodeAmpPercentPB[CH%02d]=%d\\r\\n", initial string=w3070, w3066, w3065) -> (resulting string=w3069:string)  [unwired: 1 in, 1 out]
              }
              n1300 = Format Into String(format string="PulseNamePB=%s\r\nAmplitudeLowLimitPB=%d\r\nAmplitudeStepPB=%d\r\nAmplitudeStepIndexPB=%d\r\nPulseWidthLowLimitPB=%d\r\nPulseWidthHighLimitPB=%d\r\nPulseWidthPB=%d\r\n%s", w3059, w3058, w3057, w3056, w3055, w3054, w3053, w3051) -> (resulting string=w3061:string)  [unwired: 2 in, 1 out]
              n1301 = Concatenate Strings(w3062, w3061) -> (w3063:string)
            }
            frame 3 {
              n1302 = Unbundle By Name(w3082) -> ("PC.Pulse Name"=w3081:string, "PC.Amp Low Limit (uA)"=w3080:u16, "PC.Amp Step (uA)"=w3079:u16, "PC.Amp Step Index"=w3078:u16, "PC.PW Low Limit (uS)"=w3077:u16, "PC.PW High Limit (uS)"=w3076:u16, "PC.PW Default (uS)"=w3075:u16, "PC.Amplitudes"=w3074:i8[])
              n1303 = for {
                tunnel: w3074 -> [w3093] mode=indexing
                shift-right: [w3091] -> w3073
                shift-left: "" -> [w3092]
                i -> [w3089]
                n1304 = To Byte Integer(number=w3093) -> (8bit integer=w3087:i8)
                n1305 = Increment(x=w3089) -> (x+1=w3088:i32)
                n1306 = Format Into String(format string="ElectrodeAmpPercentPC[CH%02d]=%d\\r\\n", initial string=w3092, w3088, w3087) -> (resulting string=w3091:string)  [unwired: 1 in, 1 out]
              }
              n1307 = Format Into String(format string="PulseNamePC=%s\r\nAmplitudeLowLimitPC=%d\r\nAmplitudeStepPC=%d\r\nAmplitudeStepIndexPC=%d\r\nPulseWidthLowLimitPC=%d\r\nPulseWidthHighLimitPC=%d\r\nPulseWidthPC=%d\r\n%s", w3081, w3080, w3079, w3078, w3077, w3076, w3075, w3073) -> (resulting string=w3083:string)  [unwired: 2 in, 1 out]
              n1308 = Concatenate Strings(w3084, w3083) -> (w3085:string)
            }
            frame 4 {
              n1309 = Unbundle By Name(w3104) -> ("PD.Pulse Name"=w3103:string, "PD.Amp Low Limit (uA)"=w3102:u16, "PD.Amp Step (uA)"=w3101:u16, "PD.Amp Step Index"=w3100:u16, "PD.PW Low Limit (uS)"=w3099:u16, "PD.PW High Limit (uS)"=w3098:u16, "PD.PW Default (uS)"=w3097:u16, "PD.Amplitudes"=w3096:i8[])
              n1310 = for {
                tunnel: w3096 -> [w3115] mode=indexing
                shift-right: [w3113] -> w3095
                shift-left: "" -> [w3114]
                i -> [w3111]
                n1311 = To Byte Integer(number=w3115) -> (8bit integer=w3109:i8)
                n1312 = Increment(x=w3111) -> (x+1=w3110:i32)
                n1313 = Format Into String(format string="ElectrodeAmpPercentPD[CH%02d]=%d\\r\\n", initial string=w3114, w3110, w3109) -> (resulting string=w3113:string)  [unwired: 1 in, 1 out]
              }
              n1314 = Format Into String(format string="PulseNamePD=%s\r\nAmplitudeLowLimitPD=%d\r\nAmplitudeStepPD=%d\r\nAmplitudeStepIndexPD=%d\r\nPulseWidthLowLimitPD=%d\r\nPulseWidthHighLimitPD=%d\r\nPulseWidthPD=%d\r\n%s", w3103, w3102, w3101, w3100, w3099, w3098, w3097, w3095) -> (resulting string=w3105:string)  [unwired: 2 in, 1 out]
              n1315 = Concatenate Strings(w3106, w3105) -> (w3107:string)
            }
          }
        }
        n1316 = local write "Patient Program String"(w2980) -> ()
      }
      frame "Downlink Patient Program" {
        n1317 = call "MICSD Telem Driver.vi"("VISA Resource Name"=w3116, "Command"=Typedef_Command_List."Set Program Definition", "Parameters"="Patient Program String", "error in (no error)"=w3124) -> ("Response Token"=w3121:string, "Response Code"=w3120:string, "error out"=w3123:errorcluster)  [unwired: 9 in, 4 out]
        n1318 = Concatenate Strings(w3121, " - ", w3120) -> (w3119:string)
        n1319 = local write "Response"(w3119) -> ()
      }
      frame "Set Program Active" {
        n1320 = local read "PatStim"() -> (w3128:T10)
        n1321 = Unbundle By Name(w3128) -> ("Program Number"=w3127:u8)
        n1322 = Format Into String(format string="Program=%d", w3127) -> (resulting string=w3130:string)  [unwired: 2 in, 1 out]
        n1323 = call "MICSD Telem Driver.vi"("VISA Resource Name"=w3131, "Command"=Typedef_Command_List."Select Program", "Parameters"=w3130, "error in (no error)"=w3138) -> ("Response Token"=w3135:string, "Response Code"=w3134:string, "error out"=w3137:errorcluster)  [unwired: 9 in, 4 out]
        n1324 = Concatenate Strings(w3135, " - ", w3134) -> (w3133:string)
        n1325 = local write "Response"(w3133) -> ()
      }
      frame "Start Patient Stim" {
        n1326 = call "MICSD Telem Driver.vi"("VISA Resource Name"=w3142, "Command"=Typedef_Command_List."xPG Stimulation", "Parameters"="StimState=1" ("format string"), "error in (no error)"=w3149) -> ("Response Token"=w3146:string, "Response Code"=w3145:string, "error out"=w3148:errorcluster)  [unwired: 9 in, 4 out]
        n1327 = Concatenate Strings(w3146, " - ", w3145) -> (w3144:string)
        n1328 = local write "Response"(w3144) -> ()
      }
      frame "Stop Stimulation" {
        n1329 = call "MICSD Telem Driver.vi"("VISA Resource Name"=w3153, "Command"=Typedef_Command_List."xPG Stimulation", "Parameters"="StimState=0" ("format string"), "error in (no error)"=w3160) -> ("Response Token"=w3157:string, "Response Code"=w3156:string, "error out"=w3159:errorcluster)  [unwired: 9 in, 4 out]
        n1330 = Concatenate Strings(w3157, " - ", w3156) -> (w3155:string)
        n1331 = local write "Response"(w3155) -> ()
      }
      frame "Get BS Error" {
        n1332 = case shown="\"Name\"" "BaseStationInfo" {
          tunnel: [T27."Get Device Type" ("Command") T27."Get Device Name" ("Command") T27."Get Device Version" ("Command") T27."Get Device Error" ("Command")] -> w3163
          frame "Type", Default {
          }
          frame "Name" {
          }
          frame "Version" {
          }
          frame "Error" {
          }
        }
        n1333 = call "MICSD Get Info.vi"("error in (no error)"=w3169, "Command"=w3163, "VISA Resource Name"=w3168) -> ("error out"=w3167:errorcluster, "Response"=→"BASE STATION INFO":string, "dup VISA Resource Name"=w3166:refnum<visa-resource-name>)  [unwired: 6 in]
      }
      frame "Get RSSI Base 400" {
        n1334 = local read "Working MICS Config"() -> (w3181:T20)
        n1335 = Unbundle By Name(w3181) -> ("Normal_Comm.RF_Channel"=w3180:u8)
        n1336 = Greater Than 0?(x="Base 400MHz RSSI Mode") -> (x > 0?=w3177:bool)
        n1337 = call "MICSD Do RSSI.vi"("Use Averaging?(T)"=w3177, "error in (no error)"=w3185, "Measurement Type"="Measurement Type", "Channel"=w3180, "VISA Resource Name"=w3182) -> ("error out"=w3184:errorcluster, "RSSI"=→"RSSI Base 400":u16, "dup VISA Resource Name"=w3183:refnum<visa-resource-name>)  [unwired: 4 in]
      }
      frame "Get RSSI Remote 400" {
        n1338 = local read "Working MICS Config"() -> (w3194:T20)
        n1339 = Unbundle By Name(w3194) -> ("Normal_Comm.RF_Channel"=w3193:u8)
        n1340 = Greater Than 0?(x="Remote 400MHz RSSI Mode") -> (x > 0?=w3192:bool)
        n1341 = call "MICSD Do RSSI.vi"("Execute on Remote?(F)"=TRUE, "Use Averaging?(T)"=w3192, "error in (no error)"=w3198, "Measurement Type"=T19."INT_RSSI_INT_ADC (2)", "Channel"=w3193, "VISA Resource Name"=w3195) -> ("error out"=w3197:errorcluster, "RSSI"=→"RSSI Remote 400":u16, "dup VISA Resource Name"=w3196:refnum<visa-resource-name>)  [unwired: 3 in]
      }
      frame "Save Pat Program" {
        n1342 = Open/Create/Replace File(error in=w3202, prompt="Save Patient Program", operation (0:open)=T26."replace or create with confirmation", access (0:read/write)=enum16{"read/write", "read-only", "write-only"}."write-only") -> (refnum out=w3204:refnum<file>, cancelled=w3203:bool, error out=w3205:errorcluster)  [unwired: 2 in]
        n1343 = case shown="False" w3203 {
          tunnel: w3205 -> [w3215 _]
          tunnel: w3204 -> [w3214 _]
          frame False {
            n1344 = local read "PatStim"() -> (w3211:T10)
            n1345 = Write to Binary File(file (use dialog)=w3214, data=w3211, error in=w3215) -> (refnum out=w3212:refnum<file>, error out=w3213:errorcluster)  [unwired: 3 in, 1 out]
            n1346 = case shown="No Error" w3213 {
              selector: w3213 -> [w3217 _]
              tunnel: w3212 -> [w3216 _]
              frame No Error {
                n1347 = Close File(refnum=w3216, error in=w3217) -> ()  [unwired: 2 out]
              }
              frame Error {
              }
            }
          }
          frame True {
          }
        }
      }
      frame "Load Pat Program" {
        n1348 = Open/Create/Replace File(error in=w3222, prompt="Load Patient Program", access (0:read/write)=enum16{"read/write", "read-only", "write-only"}."read-only") -> (refnum out=w3219:refnum<file>, cancelled=w3218:bool, error out=w3220:errorcluster)  [unwired: 3 in]
        n1349 = case shown="False" w3218 {
          tunnel: w3220 -> [w3232 _]
          tunnel: w3219 -> [w3231 _]
          frame False {
            n1350 = local read "PatStim"() -> (w3230:T10)
            n1351 = Read from Binary File(5:w3230, 8:w3232, 11:w3231) -> (0:w3229:errorcluster, 2:w3228:T10, 3:w3227:refnum<file>)  [unwired: 3 in, 1 out]
            n1352 = case shown="No Error" w3229 {
              selector: w3229 -> [w3234 _]
              tunnel: w3228 -> [w3235 _]
              tunnel: w3227 -> [w3233 _]
              frame No Error {
                n1353 = local write "PatStim"(w3235) -> ()
                n1354 = Close File(refnum=w3233, error in=w3234) -> ()  [unwired: 2 out]
              }
              frame Error {
              }
            }
          }
          frame True {
          }
        }
      }
      frame "Set Attenuator" {
        n1355 = case shown="\"Zero\"" "AttenMode" {
          tunnel: "Attenuation (dB)" -> [w3254 w3256 w3260 _]
          tunnel: [w3254 w3257 w3259 0.0 ("Attenuation (dB)")] -> w3241
          tunnel: enum16{"Null", "Increment", "Decrement", "Zero"}."Null" ("AttenMode") -> [w3253 w3255 w3258 w3261]
          tunnel: [w3253 w3255 w3258 w3261] -> w3237
          frame "Null", Default {
          }
          frame "Increment" {
            n1356 = Increment(x=w3256) -> (x+1=w3257:dbl)
          }
          frame "Decrement" {
            n1357 = Decrement(x=w3260) -> (x-1=w3259:dbl)
          }
          frame "Zero" {
          }
        }
        n1358 = local write "AttenMode"(w3237) -> ()
        n1359 = In Range and Coerce(upper limit=31.75, x=w3241, lower limit=0.0) -> (coerced(x)=w3240:dbl)  [unwired: 1 out]
        n1360 = Multiply(x=w3240, y=4.0) -> (x*y=w3245:dbl)
        n1361 = local write "Attenuation (dB)"(w3240) -> ()
        n1362 = To Unsigned Byte Integer(number=w3245) -> (unsigned 8bit integer=w3244:u8)
        n1363 = call "MICSD Set Attenuator.vi"("error in (no error)"=w3250, "Attenuation"=w3244, "VISA Resource Name"=w3249) -> ("error out"=w3248:errorcluster, "dup VISA Resource Name"=w3247:refnum<visa-resource-name>)  [unwired: 7 in]
      }
      frame "Set Calibration INFO_D" {
        # "Write Calibration Data to Downlink Buffer"
        n1364 = Initialize Array(u8 255, 64 ("dimension size")) -> (w3272:u8[])
        n1365 = case shown="True" "Enable \"D\" Table" {
          tunnel: w3272 -> [w3293 w3296]
          tunnel: [w3293 w3295] -> w3270
          frame False {
          }
          frame True {
            w3294 = 0
            n1366 = Replace Array Subset(array=w3296, new element=w3294, index=w3294) -> (w3295:u8[])
          }
        }
        n1367 = Replace Array Subset(array=w3270, new element="Valid Entries \"D\"", index=1) -> (w3269:u8[])
        n1368 = for {
          N: "Valid Entries \"D\"" -> [_]
          shift-right: [w3289] -> w3266
          shift-left: w3269 -> [w3288]
          tunnel: "CalData_D" -> [w3282] mode=indexing
          i -> [w3292]
          n1369 = Increment(x=w3292) -> (x+1=w3291:i32)
          n1370 = Index Array(array=w3282, index=2) -> (element=w3280:u8)
          n1371 = Index Array(array=w3282, index=1) -> (element=w3281:u8)
          n1372 = Multiply(x=2, y=w3291) -> (x*y=w3285:i32)
          n1373 = Increment(x=w3285) -> (x+1=w3286:i32)
          n1374 = Replace Array Subset(array=w3288, new element=w3281, index=w3285) -> (w3287:u8[])
          n1375 = Replace Array Subset(array=w3287, new element=w3280, index=w3286) -> (w3289:u8[])
        }
        n1376 = call "MICSD Set Calibration Data.vi"("error in (no error)"=w3279, "Calibration Data"=w3266, "Register"=enum16{"INFO_D", "INFO_C"}."INFO_D", "VISA Resource Name"=w3278) -> ("error out"=w3263:errorcluster, "dup VISA Resource Name"=w3264:refnum<visa-resource-name>)  [unwired: 6 in]
      }
      frame "Set Calibration INFO_C" {
        # "Write Calibration Data to Downlink Buffer"
        n1377 = Initialize Array(u8 255, 64 ("dimension size")) -> (w3307:u8[])
        n1378 = case shown="True" "Enable \"C\" Table" {
          tunnel: w3307 -> [w3327 w3330]
          tunnel: [w3327 w3329] -> w3305
          frame False {
          }
          frame True {
            w3328 = 0
            n1379 = Replace Array Subset(array=w3330, new element=w3328, index=w3328) -> (w3329:u8[])
          }
        }
        n1380 = Replace Array Subset(array=w3305, new element="Valid Entries \"C\"", index=1) -> (w3304:u8[])
        n1381 = for {
          N: "Valid Entries \"C\"" -> [_]
          shift-right: [w3323] -> w3303
          shift-left: w3304 -> [w3322]
          tunnel: "CalData_C" -> [w3316] mode=indexing
          i -> [w3326]
          n1382 = Increment(x=w3326) -> (x+1=w3325:i32)
          n1383 = Index Array(array=w3316, index=2) -> (element=w3314:u8)
          n1384 = Index Array(array=w3316, index=1) -> (element=w3315:u8)
          n1385 = Multiply(x=2, y=w3325) -> (x*y=w3319:i32)
          n1386 = Increment(x=w3319) -> (x+1=w3320:i32)
          n1387 = Replace Array Subset(array=w3322, new element=w3315, index=w3319) -> (w3321:u8[])
          n1388 = Replace Array Subset(array=w3321, new element=w3314, index=w3320) -> (w3323:u8[])
        }
        n1389 = call "MICSD Set Calibration Data.vi"("error in (no error)"=w3313, "Calibration Data"=w3303, "Register"=enum16{"INFO_D", "INFO_C"}."INFO_C", "VISA Resource Name"=w3312) -> ("error out"=w3297:errorcluster, "dup VISA Resource Name"=w3298:refnum<visa-resource-name>)  [unwired: 6 in]
      }
      frame "Get Calibration INFO_D" {
        # "Parse Calibration Data uplink into Panel Matrix"
        n1390 = call "MICSD Get Calibration Data.vi"("error in (no error)"=w3345, "Calibration Register"=enum16{"INFO_D", "INFO_C"}."INFO_D", "VISA Resource Name"=w3344) -> ("error out"=w3342:errorcluster, "Calibration Data"=w3336:u8[], "dup VISA Resource Name"=w3343:refnum<visa-resource-name>)  [unwired: 6 in]
        n1391 = Index Array(array=w3336, index=0) -> (element=w3340:u8)
        n1392 = Equal To 0?(x=w3340) -> (x = 0?=w3339:bool)
        n1393 = local write "Enable \"D\" Table"(w3339) -> ()
        n1394 = Index Array(array=w3336, index=1) -> (element=w3335:u8)
        n1395 = local write "Valid Entries \"D\""(w3335) -> ()
        n1396 = for {
          N: 31 -> [_]
          tunnel: w3336 -> [w3347]
          tunnel: [w3351] -> w3333 mode=indexing
          i -> [w3354]
          n1397 = Increment(x=w3354) -> (x+1=w3356:i32)
          n1398 = Multiply(x=2 ("index"), y=w3356) -> (x*y=w3349:i32)
          n1399 = Increment(x=w3354) -> (x+1=w3348:i32)
          n1400 = Increment(x=w3349) -> (x+1=w3350:i32)
          n1401 = To Unsigned Byte Integer(number=w3348) -> (unsigned 8bit integer=w3346:u8)
          n1402 = Index Array(array=w3347, index=w3349) -> (element=w3353:u8)
          n1403 = Index Array(array=w3347, index=w3350) -> (element=w3352:u8)
          n1404 = Build Array(w3346, w3353, w3352) -> (w3351:u8[])
        }
        n1405 = local write "CalData_D"(w3333) -> ()
      }
      frame "Get Calibration INFO_C" {
        # "Parse Calibration Data uplink into Panel Matrix"
        n1406 = call "MICSD Get Calibration Data.vi"("error in (no error)"=w3371, "Calibration Register"=enum16{"INFO_D", "INFO_C"}."INFO_C", "VISA Resource Name"=w3370) -> ("error out"=w3368:errorcluster, "Calibration Data"=w3362:u8[], "dup VISA Resource Name"=w3369:refnum<visa-resource-name>)  [unwired: 6 in]
        n1407 = Index Array(array=w3362, index=0) -> (element=w3366:u8)
        n1408 = Equal To 0?(x=w3366) -> (x = 0?=w3365:bool)
        n1409 = local write "Enable \"C\" Table"(w3365) -> ()
        n1410 = Index Array(array=w3362, index=1) -> (element=w3361:u8)
        n1411 = local write "Valid Entries \"C\""(w3361) -> ()
        n1412 = for {
          N: 31 -> [_]
          tunnel: w3362 -> [w3373]
          tunnel: [w3377] -> w3359 mode=indexing
          i -> [w3380]
          n1413 = Increment(x=w3380) -> (x+1=w3382:i32)
          n1414 = Multiply(x=2 ("index"), y=w3382) -> (x*y=w3375:i32)
          n1415 = Increment(x=w3380) -> (x+1=w3374:i32)
          n1416 = Increment(x=w3375) -> (x+1=w3376:i32)
          n1417 = To Unsigned Byte Integer(number=w3374) -> (unsigned 8bit integer=w3372:u8)
          n1418 = Index Array(array=w3373, index=w3375) -> (element=w3379:u8)
          n1419 = Index Array(array=w3373, index=w3376) -> (element=w3378:u8)
          n1420 = Build Array(w3372, w3379, w3378) -> (w3377:u8[])
        }
        n1421 = local write "CalData_C"(w3359) -> ()
      }
      frame "Run Calibration" {
        # "* defines to select group 1 cals */\nCAL_WAKEUP_STROBE_OSC     0x01\nCAL_TX_IF_OSC             0x02\nCAL_FM_DETECT_AND_RX_IF   0x04\nCAL_RX_ADC                0x08\nCAL_400_MHZ_TX_102        0x10  \nCAL_400_MHZ_RX_102        0x20\nCAL_400_MHZ_ANT           0x40\nCAL_24_MHZ_CRYSTAL_OSC    0x80\n/* defines to select group 2 cals/\nCAL_2_MHZ_OSC_102         (0x01 << 8) \nCAL_LNA_FREQ_102          (0x02 << 8)"
        n1422 = Build Array("CAL_WAKEUP_STROBE_OSC", "CAL_TX_IF_OSC", "CAL_FM_DETECT_AND_RX_IF", "CAL_RX_ADC", "CAL_400_MHZ_TX", "CAL_400_MHZ_RX", "CAL_400_MHZ_ANT", "CAL_24MHZ_CRYSTAL_OSC") -> (w3384:bool[])
        n1423 = Boolean Array To Number(Boolean array=w3384) -> (number=w3383:u32)
        n1424 = call "MICSD Calibrate.vi"("VISA Resource Name"=w3398, "Execute on Remote?(F)"="Execute on Remote?(F)", "CalSelect1"=w3383, "Channel"="MICS Channel", "error in (no error)"=w3399) -> ("dup VISA Resource Name"=w3397:refnum<visa-resource-name>, "error out"=w3396:errorcluster)  [unwired: 9 in]
        n1425 = flat-sequence {
          tunnel: w3396 -> [w3403]
          tunnel: [w3403] -> w3395
          frame #0 {
            n1426 = Wait (ms)(milliseconds to wait=u32 300) -> ()  [unwired: 1 out]
          }
        }
      }
      frame "Set Register" {
        n1427 = local read "Register"() -> (w3404:u16)
        n1428 = Not Equal?(x=w3404, y=u16 1000) -> (x != y?=w3405:bool)
        n1429 = case shown="True" w3405 {
          tunnel: w3404 -> [_ w3416]
          frame False {
          }
          frame True {
            n1430 = local write "Address"(w3416) -> ()
          }
        }
        n1431 = call "MICSD Set Register.vi"("Execute on Remote?(F)"="Use Remote?", "error in (no error)"=w3413, "Data"="Set Data", "Address"="Address", "VISA Resource Name"=w3412) -> ("error out"=w3408:errorcluster, "dup VISA Resource Name"=w3407:refnum<visa-resource-name>)  [unwired: 5 in]
      }
      frame "2.45GHz Remote RSSI" {
        n1432 = call "MICSD Wakeup RSSI.vi"("error in"=w3422, "RSSI Mode (Single)"="Remote 2.45G RSSI Mode", "VISA Resource Name"=w3419) -> ("error out"=w3421:errorcluster, "Wakeup RSSI"=→"RSSI Remote 2.45":i16, "dup VISA Resource Name"=w3420:refnum<visa-resource-name>)  [unwired: 6 in]
      }
      frame "Wakeup Calibrator Tool" {
        (unwired) u32 230400 ("baud rate (9600)")
        n1433 = call-poly "VISA Configure Serial Port"("VISA resource name"="SECONDARY MICS Dongle Address", "Enable Termination\nChar (T)"=FALSE ("Enable Termination\nChar (T)"), "error in (no error)"=w3429) -> ("VISA resource name out"=w3426:refnum<visa-resource-name>)  [unwired: 11 in, 1 out]
        n1434 = call "MICS Wakeup Calibration Tool.vi"("error in (no error)"=w3429, "SECONDARY MICS Dongle Address"=w3426, "PRIMARY MICS Dongle Address"=w3430) -> ("error out"=w3427:errorcluster, "Trim Settings"=→"Wakeup Cal Results":string)  [unwired: 7 in]
        n1435 = VISA Close(VISA resource name=w3426, error in (no error)=w3427) -> (error out=w3428:errorcluster)
      }
      frame "Get Register" {
        n1436 = Not Equal?(x="Register", y=u16 1000) -> (x != y?=w3436:bool)
        n1437 = case shown="True" w3436 {
          tunnel: "Register" -> [_ w3447]
          frame False {
          }
          frame True {
            n1438 = local write "Address"(w3447) -> ()
          }
        }
        n1439 = local read "Use Remote?"() -> (w3439:bool)
        n1440 = local read "Address"() -> (w3440:u16)
        n1441 = call "MICSD Get Register.vi"("Execute on Remote?(F)"=w3439, "error in (no error)"=w3444, "Address"=w3440, "VISA Resource Name"=w3443) -> ("error out"=w3442:errorcluster, "Data"=→"Get Data" →"Get Data Dec":u8, "dup VISA Resource Name"=w3441:refnum<visa-resource-name>)  [unwired: 5 in]
      }
      frame "ZL Register Mass Read" {
        n1442 = local read "Use Remote?"() -> (w3455:bool)
        n1443 = for {
          N: 255 -> [_]
          tunnel: w3455 -> [w3466]
          shift-right: [w3467] -> w3456
          shift-left: w3457 -> [w3469]
          shift-right: [w3468] -> w3452
          shift-left: w3458 -> [w3470]
          tunnel: [w3464] -> w3451 mode=indexing
          i -> [w3465]
          n1444 = call "MICSD Get Register.vi"("Execute on Remote?(F)"=w3466, "error in (no error)"=w3470, "Address"=w3465, "VISA Resource Name"=w3469) -> ("error out"=w3468:errorcluster, "Data"=w3464:u8, "dup VISA Resource Name"=w3467:refnum<visa-resource-name>)  [unwired: 5 in]
        }
        n1445 = call "MICSD Format Hex Table.vi"("Read Data"=w3451) -> ("String"=w3450:string)  [unwired: 4 in]
        n1446 = Write to Text File(file (use dialog)="File Path", text=w3450, error in=w3452) -> (refnum out=w3448:refnum<file>, error out=w3449:errorcluster)  [unwired: 1 in, 1 out]
        n1447 = case shown="No Error" w3449 {
          selector: w3449 -> [w3462 _]
          tunnel: w3448 -> [w3461 _]
          frame No Error {
            n1448 = Close File(refnum=w3461, error in=w3462) -> ()  [unwired: 2 out]
          }
          frame Error {
            n1449 = One Button Dialog(message="Could not save Register Data to File!!") -> ()  [unwired: 1 in, 1 out]
          }
        }
      }
      frame "Get Attenuator" {
        n1450 = call "MICSD Get Attenuator.vi"("error in (no error)"=w3477, "VISA Resource Name"=w3476) -> ("error out"=w3475:errorcluster, "Attenuation"=w3471:u8, "dup VISA Resource Name"=w3474:refnum<visa-resource-name>)  [unwired: 7 in]
        n1451 = Divide(x=w3471, y=4.0) -> (x/y=w3472:dbl)
        n1452 = local write "Attenuation (dB)"(w3472) -> ()
      }
      frame "Reset Dongle" {
        n1453 = call "MICSD Reset.vi"("error in (no error)"=w3486, "VISA Resource Name"=w3487) -> ("error out"=w3483:errorcluster, "dup VISA Resource Name"=w3484:refnum<visa-resource-name>)  [unwired: 8 in]
        n1454 = local read "Working MICS Config"() -> (w3480:T20)
        n1455 = call "MICSD Config.vi"("error in (no error)"=w3483, "Function"=enum16{"Write Config", "Read Config"}."Write Config", "MICS_Config_In"=w3480, "VISA Resource Name"=w3484) -> ("error out"=w3481:errorcluster, "dup VISA Resource Name"=w3482:refnum<visa-resource-name>)  [unwired: 5 in, 1 out]
      }
      frame "Load Cmd Template" {
        n1456 = local read "Command"() -> (w3495:T8)
        n1457 = call "Telemetry Downlink Templates.vi"("Command"=w3495) -> ("Template String"=w3494:string)  [unwired: 10 in]
        n1458 = local write "Parameters"(w3494) -> ()
      }
      frame "Get CCA" {
        n1459 = local read "BASE STATION RF CONTROL"() -> (w3503:T2)
        n1460 = Unbundle By Name(w3503) -> ("RSSI Measurement"=w3501:u16, "Use Averaging?"=w3502:bool)
        n1461 = call "MICSD Do CCA.vi"("error in (no error)"=w3506, "Use Averaging?"=w3502, "RSSI Mode"=w3501, "VISA Resource Name"=w3505) -> ("error out"=w3504:errorcluster, "CCA Data"=w3498:u16[], "Selected Channel"=w3496:u8, "dup VISA Resource Name"=w3497:refnum<visa-resource-name>)  [unwired: 4 in]
        n1462 = Build Array (concatenate)(u16[] [0] ("CCA Data"), w3498) -> (w3499:u16[])
        n1463 = Bundle By Name(cluster=w3503, "Manual RF CH:"=w3496, "Base Station CCA Results"=w3499) -> (w3507:T2)
        n1464 = local write "BASE STATION RF CONTROL"(w3507) -> ()
      }
      frame "Discharge Control" {
        n1465 = local read "Active"() -> (w3514:i32)
        n1466 = Increment(x=w3514) -> (x+1=w3513:i32)
        n1467 = local write "Active"(w3513) -> ()
        n1468 = case shown="15" w3513 {
          selector: w3513 -> [_ w3518]
          tunnel: [string[] [] ("States Array Out") w3519] -> w3515
          frame 15 {
            n1469 = Tick Count (ms)() -> (millisecond timer value=w3516:u32)
            n1470 = local write "Discharge Delay"(w3516) -> ()
          }
          frame 0, Default {
            n1471 = local read "Discharge"() -> (w3525:T9)
            n1472 = Index Array(array=w3525, index=w3518) -> (element=w3524:T24)
            n1473 = Unbundle By Name(w3524) -> ("Activate"=w3523:bool, "Stop"=w3526:bool, "Discharging"=w3522:bool, "Ready"=w3521:bool, "MICS ID"=w3520:u32)
            n1474 = case shown="False" w3526 {
              tunnel: w3525 -> [w3528 w3553]
              tunnel: w3524 -> [w3529 w3548]
              tunnel: w3523 -> [w3533 _]
              tunnel: w3522 -> [w3532 w3544]
              tunnel: w3521 -> [w3531 _]
              tunnel: w3520 -> [w3530 w3550]
              tunnel: [w3527 w3547] -> w3519
              tunnel: w3518 -> [_ w3546]
              frame False {
                n1475 = case shown="True" w3533 {
                  tunnel: w3532 -> [_ w3539]
                  tunnel: w3531 -> [_ _]
                  tunnel: w3530 -> [_ w3535]
                  tunnel: w3529 -> [_ _]
                  tunnel: w3528 -> [_ _]
                  tunnel: [string[] ["Discharge Control"] ("States Array Out") w3538] -> w3527
                  frame False {
                  }
                  frame True {
                    n1476 = local read "SESSION CONTROL"() -> (w3536:T3)
                    n1477 = Bundle By Name(cluster=w3536, "TARGET MICS ID"=w3535) -> (w3537:T3)
                    n1478 = local write "SESSION CONTROL"(w3537) -> ()
                    n1479 = case shown="True" w3539 {
                      tunnel: [string[] ["Open Session", "Get Status", "Monitor Discharge"] ("States Array Out") string[] ["Open Session", "Start Discharge"] ("States Array Out")] -> w3538
                      frame True {
                        n1480 = Wait (ms)(milliseconds to wait=u32 500) -> ()  [unwired: 1 out]
                        n1481 = local write "Get VBAT Single"(TRUE ("Get VBAT Single")) -> ()
                      }
                      frame False {
                        # "Initiate Discharge"
                      }
                    }
                  }
                }
              }
              frame True {
                w3545 = FALSE ("Activate")
                n1482 = local read "SESSION CONTROL"() -> (w3551:T3)
                n1483 = Bundle By Name(cluster=w3551, "TARGET MICS ID"=w3550) -> (w3549:T3)
                n1484 = local write "SESSION CONTROL"(w3549) -> ()
                n1485 = case shown="False" w3544 {
                  tunnel: [string[] ["Open Session", "Terminate Discharge"] ("States Array Out") string[] ["Discharge Control"] ("States Array Out")] -> w3547
                  frame True {
                  }
                  frame False {
                  }
                }
                n1486 = Bundle By Name(cluster=w3548, "Activate"=w3545, "Stop"=w3545, "Ready"=w3545) -> (w3554:T24)
                n1487 = Replace Array Subset(array=w3553, new element=w3554, index=w3546) -> (w3552:T9)
                n1488 = local write "Discharge"(w3552) -> ()
              }
            }
          }
        }
      }
      frame "Start Discharge" {
        w3572 = u32 200 ("mS")
        n1489 = local read "SESSION CONTROL"() -> (w3611:T3)
        n1490 = Unbundle By Name(w3611) -> ("TARGET MICS ID"=w3609:u32)
        n1491 = Bundle By Name(cluster=T21 {"Command"=enum."Get xPG Status", "Function"=enum."Transceive (DN -> UP)", "MICS_ID"=0, "EXID"=16773121, "Use Local"=FALSE, "Transceive Delay mS"=200.0, "CP_DATA IN"=[], "Parameters"=""} ("Input"), "Command"=Typedef_Command_List."Set Lead Limits", "Parameters"="currentLimit[01]=15000\r\ncurrentLimit[02]=15000\r\ncurrentLimit[03]=15000\r\ncurrentLimit[04]=15000\r\ncurrentLimit[05]=15000\r\ncurrentLimit[06]=15000\r\ncurrentLimit[07]=15000\r\ncurrentLimit[08]=15000\r\ncurrentLimit[09]=15000\r\ncurrentLimit[10]=15000\r\ncurrentLimit[11]=15000\r\ncurrentLimit[12]=15000\r\ncurrentLimit[13]=15000\r\ncurrentLimit[14]=15000\r\ncurrentLimit[15]=15000\r\ncurrentLimit[16]=15000\r\ncurrentLimit[17]=15000\r\ncurrentLimit[18]=15000\r\ncurrentLimit[19]=15000\r\ncurrentLimit[20]=15000\r\ncurrentLimit[21]=15000\r\ncurrentLimit[22]=15000\r\ncurrentLimit[23]=15000\r\ncurrentLimit[24]=15000\r\ncurrentLimit[25]=15000\r\ncurrentLimit[26]=15000\r\nchargeLimit[01]=22500\r\nchargeLimit[02]=22500\r\nchargeLimit[03]=22500\r\nchargeLimit[04]=22500\r\nchargeLimit[05]=22500\r\nchargeLimit[06]=22500\r\nchargeLimit[07]=22500\r\nchargeLimit[08]=22500\r\nchargeLimit[09]=22500\r\nchargeLimit[10]=22500\r\nchargeLimit[11]=22500\r\nchargeLimit[12]=22500\r\nchargeLimit[13]=22500\r\nchargeLimit[14]=22500\r\nchargeLimit[15]=22500\r\nchargeLimit[16]=22500\r\nchargeLimit[17]=22500\r\nchargeLimit[18]=22500\r\nchargeLimit[19]=22500\r\nchargeLimit[20]=22500\r\nchargeLimit[21]=22500\r\nchargeLimit[22]=22500\r\nchargeLimit[23]=22500\r\nchargeLimit[24]=22500\r\nchargeLimit[25]=22500\r\nchargeLimit[26]=22500", "MICS_ID"=w3609) -> (w3606:T21)
        n1492 = call "Zarlink Telemetry.vi"("error in (no error)"=w3603, "Input"=w3606, "MICS Dongle Address"=w3565) -> ("error out"=w3580:errorcluster)  [unwired: 6 in, 2 out]
        n1493 = Bundle By Name(cluster=w3606, "Command"=Typedef_Command_List."Set Pulse Constants", "Parameters"="PassiveInterphaseDelay=100\r\nPassiveRecoveryWidth=2000\r\nPassiveRecoveryHoldoff=1\r\nPassiveCBCWidth=2000\r\nPassiveCBCHoldoff=1\r\nActiveInterphaseDelay=100\r\nActiveRecoveryHoldoff=1\r\nActiveCBCWidth=100\r\nActiveCBCHoldoff=1\r\nKrecsEnabledBitMap=0x1F\r\nIncrementLockoutMsecs=500\r\nStimPhasePSDisableActive=0\r\nUncontrolledSourceSinkEnabled=0") -> (w3601:T21)
        n1494 = call "Simple Wait.vi"("mS"=w3572, "error in"=w3580) -> ("error out"=w3579:errorcluster)  [unwired: 12 in, 1 out]
        n1495 = Bundle By Name(cluster=w3601, "Command"=Typedef_Command_List."Set Background Impedance", "Parameters"="bgiAmplitude=1\nenabled=0") -> (w3597:T21)
        n1496 = Bundle By Name(cluster=w3597, "Command"=Typedef_Command_List."Get General Calibration") -> (w3586:T21)
        n1497 = call "Zarlink Telemetry.vi"("error in (no error)"=w3579, "Input"=w3601, "MICS Dongle Address"=w3565) -> ("error out"=w3602:errorcluster)  [unwired: 6 in, 2 out]
        n1498 = call "Zarlink Telemetry.vi"("error in (no error)"=w3602, "Input"=w3597, "MICS Dongle Address"=w3565) -> ("error out"=w3595:errorcluster)  [unwired: 6 in, 2 out]
        n1499 = call "Zarlink Telemetry.vi"("error in (no error)"=w3595, "Input"=w3586, "MICS Dongle Address"=w3565) -> ("error out"=w3585:errorcluster, "Output"=w3594:T28)  [unwired: 6 in, 1 out]
        n1500 = Unbundle By Name(w3594) -> ("Data"=w3593:string)
        n1501 = Match Pattern(string=w3593, regular expression="vrectMeasurementCal=") -> (before substring=w3590:string, match substring=w3591:string)  [unwired: 1 in, 2 out]
        n1502 = Concatenate Strings(w3590, w3591, "0x5DC") -> (w3588:string)
        n1503 = Bundle By Name(cluster=w3586, "Parameters"=w3588, "Command"=Typedef_Command_List."Set General Calibration") -> (w3584:T21)
        n1504 = Bundle By Name(cluster=w3584, "Parameters"="ProgramNumber=1\r\nProgramDefined=1\r\nProgramDisabled=0\r\nProgramName=SelfDischarge\r\nAllowedFrequencies[0]=0x00\r\nAllowedFrequencies[1]=0x00\r\nAllowedFrequencies[2]=0x00\r\nAllowedFrequencies[3]=0x00\r\nAllowedFrequencies[4]=0x00\r\nAllowedFrequencies[5]=0x00\r\nAllowedFrequencies[6]=0xFF\r\nAllowedFrequencies[7]=0x00\r\nProgramFrequencyIndex=52\r\nDefinedPulseMap=0x01\r\nPulseNamePA=P1\u0000\u0000\u0000\u0000\u0000\u0000\u0000\u0000\u0000\u0000\u0000\u0000\u0000\u0000\r\nAmplitudeLowLimitPA=15000\r\nAmplitudeStepPA=15\r\nAmplitudeStepIndexPA=1\r\nPulseWidthLowLimitPA=200\r\nPulseWidthHighLimitPA=400\r\nPulseWidthPA=350\r\nElectrodeAmpPercentPA[CH01]=0\r\nElectrodeAmpPercentPA[CH02]=0\r\nElectrodeAmpPercentPA[CH03]=0\r\nElectrodeAmpPercentPA[CH04]=0\r\nElectrodeAmpPercentPA[CH05]=0\r\nElectrodeAmpPercentPA[CH06]=0\r\nElectrodeAmpPercentPA[CH07]=0\r\nElectrodeAmpPercentPA[CH08]=0\r\nElectrodeAmpPercentPA[CH09]=0\r\nElectrodeAmpPercentPA[CH10]=0\r\nElectrodeAmpPercentPA[CH11]=0\r\nElectrodeAmpPercentPA[CH12]=0\r\nElectrodeAmpPercentPA[CH13]=0\r\nElectrodeAmpPercentPA[CH14]=100\r\nElectrodeAmpPercentPA[CH15]=-100\r\nElectrodeAmpPercentPA[CH16]=0\r\nElectrodeAmpPercentPA[CH17]=0\r\nElectrodeAmpPercentPA[CH18]=0\r\nElectrodeAmpPercentPA[CH19]=0\r\nElectrodeAmpPercentPA[CH20]=0\r\nElectrodeAmpPercentPA[CH21]=0\r\nElectrodeAmpPercentPA[CH22]=0\r\nElectrodeAmpPercentPA[CH23]=0\r\nElectrodeAmpPercentPA[CH24]=0\r\nElectrodeAmpPercentPA[CH25]=0\r\nElectrodeAmpPercentPA[CH26]=0\r\nPulseNamePB=P2\u0000\u0000\u0000\u0000\u0000\u0000\u0000\u0000\u0000\u0000\u0000\u0000\u0000\u0000\r\nAmplitudeLowLimitPB=10000\r\nAmplitudeStepPB=15\r\nAmplitudeStepIndexPB=1\r\nPulseWidthLowLimitPB=200\r\nPulseWidthHighLimitPB=400\r\nPulseWidthPB=300\r\nElectrodeAmpPercentPB[CH01]=0\r\nElectrodeAmpPercentPB[CH02]=0\r\nElectrodeAmpPercentPB[CH03]=0\r\nElectrodeAmpPercentPB[CH04]=0\r\nElectrodeAmpPercentPB[CH05]=0\r\nElectrodeAmpPercentPB[CH06]=0\r\nElectrodeAmpPercentPB[CH07]=0\r\nElectrodeAmpPercentPB[CH08]=0\r\nElectrodeAmpPercentPB[CH09]=0\r\nElectrodeAmpPercentPB[CH10]=0\r\nElectrodeAmpPercentPB[CH11]=0\r\nElectrodeAmpPercentPB[CH12]=0\r\nElectrodeAmpPercentPB[CH13]=0\r\nElectrodeAmpPercentPB[CH14]=0\r\nElectrodeAmpPercentPB[CH15]=0\r\nElectrodeAmpPercentPB[CH16]=0\r\nElectrodeAmpPercentPB[CH17]=0\r\nElectrodeAmpPercentPB[CH18]=0\r\nElectrodeAmpPercentPB[CH19]=0\r\nElectrodeAmpPercentPB[CH20]=0\r\nElectrodeAmpPercentPB[CH21]=0\r\nElectrodeAmpPercentPB[CH22]=0\r\nElectrodeAmpPercentPB[CH23]=0\r\nElectrodeAmpPercentPB[CH24]=0\r\nElectrodeAmpPercentPB[CH25]=0\r\nElectrodeAmpPercentPB[CH26]=0\r\nPulseNamePC=P3\u0000\u0000\u0000\u0000\u0000\u0000\u0000\u0000\u0000\u0000\u0000\u0000\u0000\u0000\r\nAmplitudeLowLimitPC=5000\r\nAmplitudeStepPC=15\r\nAmplitudeStepIndexPC=1\r\nPulseWidthLowLimitPC=200\r\nPulseWidthHighLimitPC=400\r\nPulseWidthPC=300\r\nElectrodeAmpPercentPC[CH01]=0\r\nElectrodeAmpPercentPC[CH02]=0\r\nElectrodeAmpPercentPC[CH03]=0\r\nElectrodeAmpPercentPC[CH04]=0\r\nElectrodeAmpPercentPC[CH05]=0\r\nElectrodeAmpPercentPC[CH06]=0\r\nElectrodeAmpPercentPC[CH07]=0\r\nElectrodeAmpPercentPC[CH08]=0\r\nElectrodeAmpPercentPC[CH09]=0\r\nElectrodeAmpPercentPC[CH10]=0\r\nElectrodeAmpPercentPC[CH11]=0\r\nElectrodeAmpPercentPC[CH12]=0\r\nElectrodeAmpPercentPC[CH13]=0\r\nElectrodeAmpPercentPC[CH14]=0\r\nElectrodeAmpPercentPC[CH15]=0\r\nElectrodeAmpPercentPC[CH16]=0\r\nElectrodeAmpPercentPC[CH17]=0\r\nElectrodeAmpPercentPC[CH18]=0\r\nElectrodeAmpPercentPC[CH19]=0\r\nElectrodeAmpPercentPC[CH20]=0\r\nElectrodeAmpPercentPC[CH21]=0\r\nElectrodeAmpPercentPC[CH22]=0\r\nElectrodeAmpPercentPC[CH23]=0\r\nElectrodeAmpPercentPC[CH24]=0\r\nElectrodeAmpPercentPC[CH25]=0\r\nElectrodeAmpPercentPC[CH26]=0\r\nPulseNamePD=P4\u0000\u0000\u0000\u0000\u0000\u0000\u0000\u0000\u0000\u0000\u0000\u0000\u0000\u0000\r\nAmplitudeLowLimitPD=2000\r\nAmplitudeStepPD=15\r\nAmplitudeStepIndexPD=1\r\nPulseWidthLowLimitPD=200\r\nPulseWidthHighLimitPD=400\r\nPulseWidthPD=400\r\nElectrodeAmpPercentPD[CH01]=0\r\nElectrodeAmpPercentPD[CH02]=0\r\nElectrodeAmpPercentPD[CH03]=0\r\nElectrodeAmpPercentPD[CH04]=0\r\nElectrodeAmpPercentPD[CH05]=0\r\nElectrodeAmpPercentPD[CH06]=0\r\nElectrodeAmpPercentPD[CH07]=0\r\nElectrodeAmpPercentPD[CH08]=0\r\nElectrodeAmpPercentPD[CH09]=0\r\nElectrodeAmpPercentPD[CH10]=0\r\nElectrodeAmpPercentPD[CH11]=0\r\nElectrodeAmpPercentPD[CH12]=0\r\nElectrodeAmpPercentPD[CH13]=0\r\nElectrodeAmpPercentPD[CH14]=0\r\nElectrodeAmpPercentPD[CH15]=0\r\nElectrodeAmpPercentPD[CH16]=0\r\nElectrodeAmpPercentPD[CH17]=0\r\nElectrodeAmpPercentPD[CH18]=0\r\nElectrodeAmpPercentPD[CH19]=0\r\nElectrodeAmpPercentPD[CH20]=0\r\nElectrodeAmpPercentPD[CH21]=0\r\nElectrodeAmpPercentPD[CH22]=0\r\nElectrodeAmpPercentPD[CH23]=0\r\nElectrodeAmpPercentPD[CH24]=0\r\nElectrodeAmpPercentPD[CH25]=0\r\nElectrodeAmpPercentPD[CH26]=0\r\n", "Command"=Typedef_Command_List."Set Program Definition") -> (w3576:T21)
        n1505 = disable-structure shown="Disabled" {
          disable-tunnel: w3585 -> [w3616 _]
          disable-tunnel: w3584 -> [w3615 _]
          disable-tunnel: [w3614 _] -> w3581
          disable-tunnel: w3565 -> [w3613 _]
          frame Disabled {
            n1506 = call "Zarlink Telemetry.vi"("error in (no error)"=w3616, "Input"=w3615, "MICS Dongle Address"=w3613) -> ("error out"=w3614:errorcluster)  [unwired: 6 in, 2 out]
          }
          frame Enabled {
          }
        }
        n1507 = call "Zarlink Telemetry.vi"("error in (no error)"=w3581, "Input"=w3576, "MICS Dongle Address"=w3565) -> ("error out"=w3578:errorcluster)  [unwired: 6 in, 2 out]
        n1508 = Bundle By Name(cluster=w3576, "Command"=Typedef_Command_List."Select Program", "Parameters"="ProgramNumber=1") -> (w3569:T21)
        n1509 = local read "Discharge"() -> (w3561:T9)
        n1510 = call "Simple Wait.vi"("mS"=w3572, "error in"=w3578) -> ("error out"=w3577:errorcluster)  [unwired: 12 in, 1 out]
        n1511 = local read "Active"() -> (w3562:i32)
        n1512 = call "Zarlink Telemetry.vi"("error in (no error)"=w3577, "Input"=w3569, "MICS Dongle Address"=w3565) -> ("error out"=w3573:errorcluster)  [unwired: 6 in, 2 out]
        n1513 = Bundle By Name(cluster=w3569, "Command"=Typedef_Command_List."xPG Stimulation", "Parameters"="StimState=1") -> (w3570:T21)
        n1514 = Index Array(array=w3561, index=w3562) -> (element=w3564:T24)
        n1515 = call "Simple Wait.vi"("mS"=w3572, "error in"=w3573) -> ("error out"=w3571:errorcluster)  [unwired: 12 in, 1 out]
        n1516 = call "Zarlink Telemetry.vi"("error in (no error)"=w3571, "Input"=w3570, "MICS Dongle Address"=w3565) -> ("error out"=w3566:errorcluster)  [unwired: 6 in, 2 out]
        n1517 = Bundle By Name(cluster=w3564, "Discharging"=TRUE, "Ready"=FALSE, "Activate"=TRUE) -> (w3563:T24)
        n1518 = Replace Array Subset(array=w3561, new element=w3563, index=w3562) -> (w3560:T9)
        n1519 = local write "Discharge"(w3560) -> ()
      }
      frame "Monitor Discharge" {
        n1520 = local read "VBAT (Volts)"() -> (w3620:dbl)
        n1521 = local read "Discharge"() -> (w3624:T9)
        n1522 = local read "Active"() -> (w3622:i32)
        n1523 = Index Array(array=w3624, index=w3622) -> (element=w3625:T24)
        n1524 = Less?(x=w3620, y="Discharge Target") -> (x < y?=w3619:bool)
        n1525 = Bundle By Name(cluster=w3625, "VBAT"=w3620) -> (w3623:T24)
        n1526 = Replace Array Subset(array=w3624, new element=w3623, index=w3622) -> (w3617:T9)
        n1527 = local write "Discharge"(w3617) -> ()
        n1528 = case shown="True" w3619 {
          tunnel: [string[] ["Terminate Discharge"] ("States Array Out") string[] ["Close Session", "Discharge Control"] ("States Array Out")] -> w3618
          frame True {
          }
          frame False {
          }
        }
      }
      frame "Terminate Discharge" {
        w3634 = FALSE ("Activate")
        n1529 = local read "SESSION CONTROL"() -> (w3645:T3)
        n1530 = Unbundle By Name(w3645) -> ("TARGET MICS ID"=w3644:u32)
        n1531 = Bundle By Name(cluster=T21 {"Command"=enum."Get xPG Status", "Function"=enum."Transceive (DN -> UP)", "MICS_ID"=0, "EXID"=16773121, "Use Local"=FALSE, "Transceive Delay mS"=200.0, "CP_DATA IN"=[], "Parameters"=""} ("Input"), "Command"=Typedef_Command_List."xPG Stimulation", "Parameters"="StimState=0", "MICS_ID"=w3644) -> (w3641:T21)
        n1532 = local read "Discharge"() -> (w3635:T9)
        n1533 = local read "Active"() -> (w3637:i32)
        n1534 = call "Zarlink Telemetry.vi"("error in (no error)"=w3647, "Input"=w3641, "MICS Dongle Address"=w3631) -> ("error out"=w3646:errorcluster)  [unwired: 6 in, 2 out]
        n1535 = Index Array(array=w3635, index=w3637) -> (element=w3639:T24)
        n1536 = Bundle By Name(cluster=w3639, "Activate"=w3634, "Discharging"=w3634, "Ready"=TRUE) -> (w3638:T24)
        n1537 = Replace Array Subset(array=w3635, new element=w3638, index=w3637) -> (w3636:T9)
        n1538 = local write "Discharge"(w3636) -> ()
      }
      frame "Wakeup Scan Config" {
        n1539 = local read "Test Job"() -> (w3653:T12)
        n1540 = local write "RFStop"(FALSE ("RFStop")) -> ()
        n1541 = Array Size(array=w3653) -> (size(s)=w3651:i32)
        n1542 = Greater Than 0?(x=w3651) -> (x > 0?=w3652:bool)
        n1543 = case shown="False" w3652 {
          tunnel: [T23."Disabled and Grayed Out" ("Disabled") T23."Enabled" ("Disabled")] -> w3650
          tunnel: [string[] ["Get Status"] string[] ["Wakeup Scan Run"]] -> w3654
          frame False {
            n1544 = One Button Dialog(message="No Job Data!\n\nConfigure or load a Job and try again.") -> ()  [unwired: 1 in, 1 out]
          }
          frame True {
            n1545 = local write "Wakeup Scan Results"("" ("Wakeup Scan Results")) -> ()
          }
        }
        n1546 = property on="RFScanStat" class="Clust (strict)"("DisabledEnum"=w3650) -> ()  [unwired: 2 in, 2 out]
      }
      frame "Wakeup Scan Run" {
        n1547 = Array Size(array=w3667) -> (size(s)=w3666:i32)
        n1548 = while {
          tunnel: w3667 -> [w3704]
          tunnel: w3664 -> [w3697]
          tunnel: w3666 -> [w3677]
          shift-right: [w3689] -> _
          shift-left: w3668 -> [w3681]
          i -> [w3686]
          stop <- w3698 stop-if-true
          n1549 = Index Array(array=w3704, index=w3686) -> (element=w3703:T30)
          n1550 = Unbundle By Name(w3681) -> ("status"=w3680:bool)
          n1551 = local read "Working MICS Config"() -> (w3702:T20)
          n1552 = Unbundle(w3703) -> ("Number of Runs"=w3693:dbl, "2.45G_TX_Pwr"=w3685:T31, "400M_TX_Pwr"=w3676:T32, "Idle Interval, S"=w3671:dbl, "Attenuator, dB"=w3684:dbl, "MICS Chan"=w3683:T33, "Random\nOffset"=w3673:bool)
          n1553 = Bundle By Name(cluster=w3702, "245TX_Power"=w3685, "Normal_Comm.RF_Channel"=w3683) -> (w3701:T20)
          n1554 = local read "RFStop"() -> (w3675:bool)
          n1555 = Increment(x=w3686) -> (x+1=w3679:i32)
          n1556 = Increment(x=w3686) -> (x+1=w3678:i32)
          n1557 = Greater Or Equal?(x=w3679, y=w3677) -> (x >= y?=w3699:bool)
          n1558 = local write "RFST"(1) -> ()
          n1559 = Random Number (0-1)() -> (number: 0 to 1=w3670:dbl)
          n1560 = Divide(x=w3678, y=w3677) -> (x/y=w3694:dbl)
          n1561 = Multiply(x=w3684, y=4.0) -> (x*y=w3692:dbl)
          n1562 = Compound Arithmetic op=OR(w3675, w3699, w3680) -> (w3698:bool)
          n1563 = Add(x=w3671, y=w3670) -> (x+y=w3672:dbl)
          n1564 = call "MICSD Config.vi"("error in (no error)"=w3681, "Function"=enum16{"Write Config", "Read Config"}."Write Config", "MICS_Config_In"=w3701, "VISA Resource Name"=w3697) -> ("error out"=w3696:errorcluster, "dup VISA Resource Name"=w3695:refnum<visa-resource-name>)  [unwired: 5 in, 1 out]
          n1565 = Select(t=w3672, s=w3673, f=w3671) -> (s? t:f=w3674:dbl)
          n1566 = To Unsigned Byte Integer(number=w3692) -> (unsigned 8bit integer=w3690:u8)
          n1567 = case shown="False" w3675 {
            tunnel: w3696 -> [w3719 w3860]
            tunnel: w3695 -> [w3718 _]
            tunnel: w3674 -> [w3717 _]
            tunnel: w3694 -> [w3716 _]
            tunnel: w3693 -> [w3715 _]
            tunnel: w3690 -> [w3714 _]
            tunnel: [w3713 w3860] -> w3689
            tunnel: "Test Job Note" -> [w3712 _]
            tunnel: "Test Device Info (for report):" -> [w3711 _]
            tunnel: w3686 -> [w3710 _]
            tunnel: w3685 -> [w3709 _]
            tunnel: w3684 -> [w3708 _]
            tunnel: w3683 -> [w3707 _]
            tunnel: w3677 -> [w3706 _]
            tunnel: w3676 -> [w3705 _]
            frame False {
              n1568 = stacked-sequence {
                seq-local: [w3735 _] -> [_ w3805]
                seq-local: [w3732 _] -> [_ w3823]
                seq-local: [w3733 _] -> [_ w3822]
                seq-local: [w3724 _] -> [_ w3810]
                seq-local: [w3727 _] -> [_ w3809]
                seq-local: [w3720 _] -> [_ w3801]
                tunnel: w3719 -> [w3728 _]
                tunnel: w3718 -> [w3729 _]
                tunnel: w3717 -> [w3726 w3812]
                tunnel: w3716 -> [w3740 _]
                tunnel: w3715 -> [w3739 w3818]
                tunnel: w3714 -> [w3736 _]
                tunnel: [_ w3805] -> w3713
                tunnel: w3712 -> [_ w3828]
                tunnel: w3711 -> [_ w3827]
                tunnel: w3710 -> [_ w3803]
                tunnel: w3706 -> [_ w3808]
                tunnel: w3709 -> [_ w3816]
                tunnel: w3705 -> [w3722 w3815]
                tunnel: w3708 -> [_ w3814]
                tunnel: w3707 -> [_ w3813]
                frame #0 {
                  # "<--"
                  # "<--"
                  # "Wait \"Interval\" time,\nAttempt \"Open Session\",\nAbort If Successful.\n\nMeasure Elapsed Time of\n\"Open Session\" process"
                  # "<--"
                  # "<--"
                  # "<--"
                  # "<--"
                  # "<--"
                  # "<--"
                  # "<--"
                  # "<--"
                  # "<--"
                  n1569 = case shown="\"1\", Default" w3722 {
                    selector: w3722 -> [_ w3743]
                    tunnel: [w3742 w3747] -> w3731
                    tunnel: [w3741 w3746] -> w3730
                    tunnel: w3729 -> [w3741 w3745]
                    tunnel: w3728 -> [w3742 w3744]
                    frame "Default" {
                    }
                    frame "1", Default {
                      n1570 = call "MICSD Set Register.vi"("error in (no error)"=w3744, "Data"=w3743, "Address"=u16 99, "VISA Resource Name"=w3745) -> ("error out"=w3747:errorcluster, "dup VISA Resource Name"=w3746:refnum<visa-resource-name>)  [unwired: 6 in]
                    }
                  }
                  n1571 = call "MICSD Set Attenuator.vi"("error in (no error)"=w3731, "Attenuation"=w3736, "VISA Resource Name"=w3730) -> ("error out"=w3737:errorcluster, "dup VISA Resource Name"=w3738:refnum<visa-resource-name>)  [unwired: 7 in]
                  n1572 = Multiply(x=w3726, y=1000.0) -> (x*y=w3723:dbl)
                  n1573 = while {
                    tunnel: w3738 -> [w3781]
                    shift-right: [w3764] -> w3735
                    shift-left: w3737 -> [w3780]
                    tunnel: w3739 -> [w3759]
                    tunnel: w3723 -> [w3754]
                    tunnel: [w3767] -> w3732 mode=indexing
                    tunnel: [w3768] -> w3733 mode=indexing
                    tunnel: w3740 -> [w3773]
                    shift-right: [w3750] -> w3727
                    shift-left: u16 0 -> [w3775]
                    shift-right: [w3771] -> _
                    shift-left: 0.0 -> [w3772]
                    tunnel: [w3758] -> w3724
                    tunnel: [w3749] -> w3720
                    i -> [w3777]
                    stop <- w3778 stop-if-true
                    n1574 = Select(t=0.0, s="RFStop", f=w3754) -> (s? t:f=w3753:dbl)
                    n1575 = call "Simple Wait.vi"("mS"=w3753, "error in"=w3780) -> ("error out"=w3765:errorcluster)  [unwired: 12 in, 1 out]
                    n1576 = Increment(x=w3777) -> (x+1=w3751:i32)
                    n1577 = local read "Wait Time (S)"() -> (w3782:u8)
                    n1578 = stacked-sequence {
                      tunnel: w3765 -> [w3795]
                      tunnel: [w3795] -> w3785
                      tunnel: [w3794] -> w3784
                      frame #0 {
                        n1579 = Tick Count (ms)() -> (millisecond timer value=w3794:u32)
                        "RFST" <- 2
                      }
                    }
                    n1580 = Unbundle By Name(w3765) -> ("status"=w3766:bool)
                    n1581 = Divide(x=w3751, y=w3759) -> (x/y=w3774:dbl)
                    n1582 = Greater Or Equal?(x=w3751, y=w3759) -> (x >= y?=w3779:bool)
                    n1583 = local read "Enable WD?"() -> (w3783:bool)
                    n1584 = Compound Arithmetic op=OR("RFStop", w3779, w3766) -> (w3778:bool)
                    n1585 = call "MICSD Start Session.vi"("error in (no error)"=w3785, "Enable Watchdog?(T)"=w3783, "Wait Time (S)"=w3782, "VISA Resource Name"=w3781) -> ("error out"=w3789:errorcluster, "dup VISA Resource Name"=w3788:refnum<visa-resource-name>)  [unwired: 6 in]
                    n1586 = call "MICSD Status.vi"("VISA Resource Name"=w3788, "error in (no error)"=w3789) -> ("dup VISA Resource Name"=w3763:refnum<visa-resource-name>, "Status Flags"=w3786:T6, "error out"=w3787:errorcluster)  [unwired: 7 in, 4 out]
                    n1587 = local write "STATUS FLAGS"(w3786) -> ()
                    n1588 = Unbundle By Name(w3786) -> ("IN_SESSION"=w3768:bool)
                    n1589 = stacked-sequence {
                      tunnel: w3787 -> [w3798]
                      tunnel: [w3798] -> w3762
                      tunnel: [w3797] -> w3792
                      frame #0 {
                        n1590 = local write "RFST"(1) -> ()
                        n1591 = Tick Count (ms)() -> (millisecond timer value=w3797:u32)
                      }
                    }
                    n1592 = Increment(x=w3775) -> (x+1=w3776:u16)
                    n1593 = Subtract(x=w3792, y=w3784) -> (x-y=w3791:u32)
                    n1594 = Select(t=w3775, s=w3768, f=w3776) -> (s? t:f=w3750:u16)
                    n1595 = call "Simple Wait.vi"("mS"=u32 500, "error in"=w3762) -> ("error out"=w3761:errorcluster)  [unwired: 12 in, 1 out]
                    n1596 = Divide(x=w3791, y=u32 1000) -> (x/y=w3767:dbl)
                    n1597 = Add(x=w3772, y=w3767) -> (x+y=w3771:dbl)
                    n1598 = call "MICSD Abort.vi"("error in (no error)"=w3761, "VISA Resource Name"=w3763) -> ("error out"=w3764:errorcluster)  [unwired: 8 in, 1 out]
                    n1599 = Divide(x=w3771, y=w3751) -> (x/y=w3758:dbl)
                    n1600 = local write "Tab Control"(T1."Tools" ("Tab Control")) -> ()
                    n1601 = Subtract(x=w3751, y=w3750) -> (x-y=w3752:i32)
                    n1602 = Bundle(cluster=T13 {"Section"=0.0, "Job"=0.0, "Last Open Session Time, S"=0.0, "Session Verified?"=FALSE, "Average Open Session Time, S"=0.0, "# of Open Session Failures"=0} ("RFScanStat"), "Section"=w3774, "Job"=w3773, "Last Open Session Time, S"=w3767, "Session Verified?"=w3768, "Average Open Session Time, S"=w3758, "# of Open Session Failures"=w3750) -> (→"RFScanStat":T13)
                    n1603 = Divide(x=w3752, y=w3751) -> (x/y=w3749:dbl)
                  }
                }
                frame #1 {
                  # "Construct Report entry"
                  n1604 = Equal To 0?(x=w3803) -> (x = 0?=w3826:bool)
                  n1605 = local read "Wakeup Scan Results"() -> (w3825:string)
                  n1606 = case shown="True" w3826 {
                    tunnel: w3828 -> [_ w3851]
                    tunnel: w3827 -> [_ w3852]
                    tunnel: w3825 -> [w3848 w3859]
                    tunnel: [w3847 w3858] -> w3824
                    tunnel: w3808 -> [_ w3850]
                    tunnel: w3803 -> [w3845 _]
                    frame False {
                      n1607 = Format Into String(format string="[Job Index %d]\r\n", initial string=w3848, w3845) -> (resulting string=w3847:string)  [unwired: 1 in, 1 out]
                    }
                    frame True {
                      n1608 = Get Date/Time In Seconds() -> (seconds since 1Jan1904=w3854:timestamp)
                      n1609 = Get Date/Time String(seconds (now)=w3854) -> (date string=w3857:string, time string=w3856:string)  [unwired: 2 in]
                      n1610 = Concatenate Strings(w3857, " - ", w3856) -> (w3853:string)
                      n1611 = Format Into String(format string="[RF Wakeup Scan Report]\r\n\r\n[Time]: %s\r\n\r\n[Test Device Info]\r\n\r\n%s\r\n\r\n[Test Job Note]\r\n\r\n%s\r\n\r\n[Number of Job Steps]:\t%d\r\n\r\n[Job Index 0]\r\n", initial string=w3859, w3853, w3852, w3851, w3850) -> (resulting string=w3858:string)  [unwired: 1 in, 1 out]
                    }
                  }
                  n1612 = for {
                    tunnel: w3823 -> [w3842] mode=indexing
                    tunnel: w3822 -> [w3837] mode=indexing
                    shift-right: [w3843] -> w3811
                    shift-left: "" -> [w3844]
                    tunnel: [w3836] -> w3821
                    i -> [w3836]
                    n1613 = Select(t="PASS", s=w3837, f="FAIL") -> (s? t:f=w3840:string)
                    n1614 = Format Into String(format string="%d\\t%^.3e\\t%s\\r\\n", initial string=w3844, w3836, w3842, w3840) -> (resulting string=w3843:string)  [unwired: 1 in, 1 out]
                  }
                  n1615 = Not A Number/Path/Refnum?(number/path/refnum=w3801) -> (NaN/Path/Refnum?=w3802:bool)
                  n1616 = Select(t=0.0, s=w3802, f=w3801) -> (s? t:f=w3799:dbl)
                  n1617 = Increment(x=w3821) -> (x+1=w3817:i32)
                  n1618 = Format Into String(format string="# of Runs Expected:\t%d\r\n# of Runs Reported:\t%d\r\n2.45GHz TX Pwr:\t%s dBm\r\n400MHz TX Setting:\t%s\r\nAttenuator:\t%0.2f dB\r\nMICS Channel:\t%s\r\nIdle Interval:\t%0.3f S\r\n[MEASUREMENT DATA]\r\nRun #\tTime to Connect\tSession Check\r\n%sAverage Connect Time:\t%0.3f\r\nNumber of Failed Attempts:\t%d\r\nSuccess Ratio:\t%0.3f\r\n[END Job Index %d]\r\n\r\n", initial string=w3824, w3818, w3817, w3816, w3815, w3814, w3813, w3812, w3811, w3810, w3809, w3799, w3803) -> (resulting string=w3807:string)  [unwired: 1 in, 1 out]
                  n1619 = case shown="Error" w3805 {
                    selector: w3805 -> [_ w3835]
                    tunnel: w3807 -> [w3829 w3833]
                    tunnel: [w3829 w3832] -> w3806
                    tunnel: "ERROR\\r\\nCode: %d\\r\\nMessage: %s\\r\\n\\r\\n" ("format string") -> [_ w3830]
                    frame No Error {
                    }
                    frame Error {
                      n1620 = call <vilib>:"Simple Error Handler.vi"("error in (no error)"=w3835) -> ("code out"=w3831:i32, "source out"=w3834:string)  [unwired: 4 in, 3 out]
                      n1621 = Format Into String(format string=w3830, initial string=w3833, w3831, w3834) -> (resulting string=w3832:string)  [unwired: 1 in, 1 out]
                    }
                  }
                  "Wakeup Scan Results" <- w3806
                }
              }
            }
            frame True {
            }
          }
        }
      }
      frame "Save RF Scan Report" {
        n1622 = call "File Dialog"("start path"=path "C:/RF Scan Reports", "prompt"="Save RF Scan Report", "button label"="Save Report", "default name"="RF Scan Data.txt", "pattern (all files)"="*.txt", "pattern label"="Text Files") -> ("selected path"=w3869:path, "cancelled"=w3863:bool, "error out"=w3862:errorcluster)  [unwired: 6 in, 1 out]
        n1623 = local read "Wakeup Scan Results"() -> (w3873:string)
        n1624 = case shown="False" w3863 {
          tunnel: w3862 -> [w3880 w3885]
          tunnel: w3869 -> [w3879 _]
          tunnel: w3873 -> [w3876 _]
          tunnel: [w3875 w3885] -> w3874
          frame False {
            n1625 = Write to Text File(file (use dialog)=w3879, text=w3876, error in=w3880) -> (refnum out=w3877:refnum<file>, error out=w3878:errorcluster)  [unwired: 1 in, 1 out]
            n1626 = case shown="No Error" w3878 {
              selector: w3878 -> [w3883 w3884]
              tunnel: w3877 -> [w3882 _]
              tunnel: [w3881 w3884] -> w3875
              frame No Error {
                n1627 = Close File(refnum=w3882, error in=w3883) -> (error out=w3881:errorcluster)  [unwired: 1 out]
              }
              frame Error {
              }
            }
          }
          frame True {
          }
        }
      }
      frame "Save RF Job" {
        w3889 = T34 {"Test Job Note"="Test Job Note", "Test Job"=[{"Number of Runs"=5.0, "2.45G_TX_Pwr"=enum."0", "400M_TX_Pwr"=enum."Default", "Idle Interval, S"=5.0, "Attenuator, dB"=0.0, "MICS Chan"=enum."CH 5", "Verify\nSessions"=FALSE}, {"Number of Runs"=5.0, "2.45G_TX_Pwr"=enum."0", "400M_TX_Pwr"=enum."Default", "Idle Interval, S"=5.0, "Attenuator, dB"=2.0, "MICS Chan"=enum."CH 5", "Verify\nSessions"=FALSE}, {"Number of Runs"=5.0, "2.45G_TX_Pwr"=enum."0", "400M_TX_Pwr"=enum."Default", "Idle Interval, S"=5.0, "Attenuator, dB"=4.0, "MICS Chan"=enum."CH 5", "Verify\nSessions"=FALSE}, {"Number of Runs"=5.0, "2.45G_TX_Pwr"=enum."0", "400M_TX_Pwr"=enum."Default", "Idle Interval, S"=5.0, "Attenuator, dB"=6.0, "MICS Chan"=enum."CH 5", "Verify\nSessions"=FALSE}]}  # TestJobType
        n1628 = local read "Test Job Note"() -> (w3888:string)
        n1629 = local read "Test Job"() -> (w3887:T12)
        n1630 = Bundle By Name(cluster=w3889, "Test Job Note"=w3888, "Test Job"=w3887) -> (w3886:T34)
        n1631 = call "File Dialog2"("start path"=path "C:/RF Scan", "prompt"="Save RF Scan Job", "button label"="Save Job", "default name"="RF Scan Job.rfj", "pattern (all files)"="*.rfj", "pattern label"="RF Scan Job Files") -> ("selected path"=w3898:path, "cancelled"=w3892:bool, "error out"=w3891:errorcluster)  [unwired: 6 in, 1 out]
        n1632 = case shown="False" w3892 {
          tunnel: w3891 -> [w3908 w3913]
          tunnel: w3898 -> [w3907 _]
          tunnel: [w3904 w3913] -> w3902
          tunnel: w3886 -> [w3903 _]
          frame False {
            n1633 = Write to Binary File(file (use dialog)=w3907, data=w3903, error in=w3908) -> (refnum out=w3905:refnum<file>, error out=w3906:errorcluster)  [unwired: 3 in, 1 out]
            n1634 = case shown="No Error" w3906 {
              selector: w3906 -> [w3911 w3912]
              tunnel: w3905 -> [w3910 _]
              tunnel: [w3909 w3912] -> w3904
              frame No Error {
                n1635 = Close File(refnum=w3910, error in=w3911) -> (error out=w3909:errorcluster)  [unwired: 1 out]
              }
              frame Error {
              }
            }
          }
          frame True {
          }
        }
      }
      frame "Load RF Job" {
        n1636 = call "File Dialog3"("start path"=path "C:/RF Scan", "prompt"="Load RF Scan Job", "button label"="Load Job", "default name"="RF Scan Job.rfj", "pattern (all files)"="*.rfj", "pattern label"="RF Scan Job Files") -> ("selected path"=w3922:path, "cancelled"=w3916:bool, "error out"=w3915:errorcluster)  [unwired: 6 in, 1 out]
        n1637 = case shown="False" w3916 {
          tunnel: w3915 -> [w3935 w3942]
          tunnel: w3922 -> [w3934 _]
          tunnel: [w3931 w3942] -> w3926
          frame False {
            w3930 = T34 {"Test Job Note"="Test Job Note", "Test Job"=[{"Number of Runs"=5.0, "2.45G_TX_Pwr"=enum."0", "400M_TX_Pwr"=enum."Default", "Idle Interval, S"=5.0, "Attenuator, dB"=0.0, "MICS Chan"=enum."CH 5", "Verify\nSessions"=FALSE}, {"Number of Runs"=5.0, "2.45G_TX_Pwr"=enum."0", "400M_TX_Pwr"=enum."Default", "Idle Interval, S"=5.0, "Attenuator, dB"=2.0, "MICS Chan"=enum."CH 5", "Verify\nSessions"=FALSE}, {"Number of Runs"=5.0, "2.45G_TX_Pwr"=enum."0", "400M_TX_Pwr"=enum."Default", "Idle Interval, S"=5.0, "Attenuator, dB"=4.0, "MICS Chan"=enum."CH 5", "Verify\nSessions"=FALSE}, {"Number of Runs"=5.0, "2.45G_TX_Pwr"=enum."0", "400M_TX_Pwr"=enum."Default", "Idle Interval, S"=5.0, "Attenuator, dB"=6.0, "MICS Chan"=enum."CH 5", "Verify\nSessions"=FALSE}]}  # TestJobType
            n1638 = Read from Binary File(5:w3930, 8:w3935, 11:w3934) -> (0:w3933:errorcluster, 2:w3929:T34, 3:w3932:refnum<file>)  [unwired: 3 in, 1 out]
            n1639 = Unbundle By Name(w3929) -> ("Test Job Note"=w3928:string, "Test Job"=w3927:T35)
            n1640 = case shown="No Error" w3933 {
              selector: w3933 -> [w3940 w3941]
              tunnel: w3932 -> [w3939 _]
              tunnel: [w3938 w3941] -> w3931
              tunnel: w3928 -> [w3937 _]
              tunnel: w3927 -> [w3936 _]
              frame No Error {
                n1641 = local write "Test Job Note"(w3937) -> ()
                n1642 = local write "Test Job"(w3936) -> ()
                n1643 = Close File(refnum=w3939, error in=w3940) -> (error out=w3938:errorcluster)  [unwired: 1 out]
              }
              frame Error {
              }
            }
          }
          frame True {
          }
        }
      }
    }
    n1644 = Or(x="stop", y=w17) -> (x .or. y?=w18:bool)
    "Error Monitor" <- w19
  }
  "error out" <- w10
  n1645 = VISA Close(VISA resource name=w1) -> ()  [unwired: 1 in, 1 out]
